vi "MAIN.vi"() -> ()   [LabVIEW 2015]
doc: "Use this template to create an application that executes repeatedly until you click the Stop button. This template polls the state of the Stop button and does not use events. Use the Top-Level Application template (not available in the Base package) to create a single-loop application with event handling."
uses:
  Control-CDC data.ctl
  Control-IMU data.ctl
  Control-Operation Test State FTS.ctl
  Lib_Bled112 toolkit/type_def/connection_status_bundle.ctl
  Lib_Bled112 toolkit/type_def/address_type.ctl
  Control-BLED Rx (EVENT-Attribute Client).ctl
  Lib_Bled112 toolkit/type_def/message_type.ctl
  Lib_Bled112 toolkit/type_def/message_class.ctl
  sub/Operation mode.ctl
  sub/Linerity State.ctl
  <vilib>/Utility/miscctls.llb/LVPointTypeDef.ctl
  SUB_Load and Save Controls.llb/RWC_Actions.ctl
  <vilib>/Utility/miscctls.llb/LVRowAndColumnTypeDef.ctl
  Type definition/write_mode.ctl
  Control-Operation State Mark10.ctl
  <vilib>/event_ctls.llb/eventvkey.ctl
  sub/File Control/File_Control_mode.ctl
  sub/Power supply/382280_mode.ctl
  <vilib>/Analysis/baseanly.llb/Mean (DBL).vi
  <vilib>/Utility/config.llb/Read Key (String).vi
  <vilib>/Utility/config.llb/Read Key (I32).vi
  Lib_Bled112 toolkit/ble_functions/ble_write_by_handle_uint8array.vi
  <vilib>/Utility/config.llb/Write Key (String).vi
  <vilib>/Utility/config.llb/Write Key (U32).vi
  <vilib>/Utility/config.llb/NI_LVConfig.lvlib
  <vilib>/Analysis/NI_AALBase.lvlib
  <vilib>/Utility/sysdir.llb/System Directory Type.ctl
  <vilib>/Utility/NIReport.llb/NI_report.lvclass
  <vilib>/addons/_office/NI_ReportGenerationToolkit.lvlib
  <vilib>/addons/_office/excel.llb/Excel Easy Table (str).vi
  <vilib>/Utility/NIReport.llb/Excel/NI_Excel.lvclass
  <vilib>/addons/_office/_exclsub.llb/font.ctl
panel:
  in  "PWR OFF":bool
  in  "File Path Done":bool
  in  "Linerity State":T1
  in  "Mode":bool=TRUE
  out "Bat(raw)":u16 format="%04x"
  out "Disconnection ocurrence":refnum<k4>
  out "Test Data table for Load Accuarcy Test":string[][](table)=[["-", "-", "-", "-", "-", "-", "-"], ["-", "-", "-", "-", "-", "-", "-"], ["-", "-", "-", "-", "-", "-", "-"], ["-", "-", "-", "-", "-", "-", "-"], ["-", "-", "-", "-", "-", "-", "-"], ["-", "-", "-", "-", "-", "-", "-"], ["-", "-", "-", "-", "-", "-", "-"], ["-", "-", "-", "-", "-", "-", "-"], ["-", "-", "-", "-", "-", "-", "-"]]
  out "Packet No.":u16
  out "Rx-debug":bool
  out "FTS table index":i32
  out "ms timer 5":u32=38996702
  out "ms timer 4":u32=27271323
  out "ms timer 3":u32=38996702
  in  "Update(ms)":u16=100
  out "ms timer 2":u32=38996702
  out "Rx-ROM":bool
  out "BLE Packet (mon)":u8[](array[numeric])=[119, 32, 48, 163, 32, 0, 45, 32, 53, 143, 30, 162, 83, 32, 86, 151, 32, 67, 185, 208, 89, 94, 66, 75, 91, 193, 107, 187, 98, 158, 102, 165, 208]
  out "Timer-ble log":u32=38996556
  in  "log data1":bool
  out "log ble buf":string
  out "Packet Detect":bool
  out "Disconnected":bool
  out "Rx buf 1":string
  out "Rx Cnt":i32
  out "Rx Packet Structure":T2={"Message Type (Response)"=128, "Payload length"=25, "Command Class (System)"=4, "Message ID"=5, "Connection handle"=0, "Attribute handle"=11, "Attribute type"=1, "Attribute value (data)"=[119, 32, 48, 110, 31, 255, 217, 32, 53, 83, 30, 161, 69, 32, 87, 130, 32, 68, 21, 209]} {"Attribute type" format="%02x" items=["read", "notify", "indicate", "read_by_type", "read_blob", "indicate_rsp_req"]; "Attribute value (data)" format="%02x"; "Attribute handle" format="%04x"; "Connection handle" format="%02x"; "Message ID" format="%02x"; "Message Type (Response)" format="%02x" items=["Command / Response"=0, "Event"=128]; "Command Class (System)" format="%02x" items=["System", "Persistent Store", "Attribute database", "Connection", "Attribute client", "Security Manager", "Generic Access Profile", "Hardware"]}
  out "Device Name":string="GEN4_PERSONA_3rd_jun"
  out "Connection Status":T5={"MAC Address"="F8:B8:54:EF:76:8D", "cnx handle"=0, "cnx flags"=5, "Address Type"=1, "Connection Interval (ms)"=8, "Timeout(ms)"=1000, "Latency"=0, "bonding handle"=255} {"Address Type" items=["Public", "Random"]}
  in  "Log no":string="1" caption="No."
  in  "FTS OP status":T7="Test_Start"
  out "Test profile":string[][](array[string])=[["Load(1)-0lb", "0", "1000", "0", "0"], ["Init(1)-70lb", "70", "1000", "0", "0"], ["Init(2)-140lb", "140", "1000", "0", "0"], ["Init(1)-70lb", "70", "1000", "0", "0"], ["Init(2)-140lb", "140", "1000", "0", "0"], ["Load(1)-0lb", "0", "10000", "1", "1"], ["Load(2)-10lb", "10", "3000", "0", "1"], ["Load(3)-20lb", "20", "3000", "0", "1"], ["Load(4)-40lb", "40", "3000", "0", "1"], ["Load(5)-60lb", "60", "3000", "0", "1"], ["Load(6)-80lb", "80", "3000", "0", "1"]]
  out "log refnum":refnum<file> caption="참조 번호 복제"
  out "ms timer":u32=38996556
  out "Logging No.":u32
  in  "Data Logging":bool caption="Data Logging (Desktop folder)"
  out "RxD":string
  out "Graph timer 2":u32=38996702
  out "Maximize window":bool
  out "Comm err cnt 1":i32
  out "Graph timer 1":u32=38996702
  in  "Setting load":bool=TRUE
  out "ACT-Comm":bool
  in  "Comm con 1":bool
  in  "Port close 1":bool
  in  "Port open 1":bool
  in  "탭-Top":T8(tab)
  in  "CDC Graph plot":bool
  in  "Offset Souce":enum32{"Normal", "Raw"}(radio)
  out "CDC Offet":T9 caption="CDC Offset data" {"Right Wing-C, C6/C0" format="%#.9f"; "Right Wing-B, C5/C0" format="%#.9f"; "Right Wing-A, C4/C0" format="%#.9f"; "Left Wing-C, C3/C0" format="%#.9f"; "Left Wing-B, C2/C0" format="%#.9f"; "Left Wing-A, C1/C0" format="%#.9f"}
  in  "Export graph 1":bool
  in  "Clear graph 1":bool
  out "CDC(PCAP02) Graph":waveform(dbl)[](graph)=[{"t0"=timestamp(3566271640.952271 s since 1904-01-01), "dt"=0.10400000000000001, "Y"=[22878.0]}, {"t0"=timestamp(3566271640.952271 s since 1904-01-01), "dt"=0.10400000000000001, "Y"=[16971.0]}, {"t0"=timestamp(3566271640.952271 s since 1904-01-01), "dt"=0.10400000000000001, "Y"=[23489.0]}, {"t0"=timestamp(3566271640.952271 s since 1904-01-01), "dt"=0.10400000000000001, "Y"=[27579.0]}, {"t0"=timestamp(3566271640.952271 s since 1904-01-01), "dt"=0.10400000000000001, "Y"=[25246.0]}, {"t0"=timestamp(3566271640.952271 s since 1904-01-01), "dt"=0.10400000000000001, "Y"=[26279.0]}, {"t0"=timestamp(3566271640.952271 s since 1904-01-01), "dt"=0.10400000000000001, "Y"=[1.0058650970458984]}, {"t0"=timestamp(3566271640.952271 s since 1904-01-01), "dt"=0.10400000000000001, "Y"=[0.9999599456787109]}, {"t0"=timestamp(3566271640.952271 s since 1904-01-01), "dt"=0.10400000000000001, "Y"=[1.0064787864685059]}, {"t0"=timestamp(3566271640.952271 s since 1904-01-01), "dt"=0.10400000000000001, "Y"=[0.9571785926818848]}, {"t0"=timestamp(3566271640.952271 s since 1904-01-01), "dt"=0.10400000000000001, "Y"=[1.0106620788574219]}, {"t0"=timestamp(3566271640.952271 s since 1904-01-01), "dt"=0.10400000000000001, "Y"=[1.0083107948303223]}]
  out "CDC data":T9 caption="CDC Monitoring data" {"Right Wing-C, C6/C0" format="%#.9f"; "Right Wing-B, C5/C0" format="%#.9f"; "Right Wing-A, C4/C0" format="%#.9f"; "Left Wing-C, C3/C0" format="%#.9f"; "Left Wing-B, C2/C0" format="%#.9f"; "Left Wing-A, C1/C0" format="%#.9f"}
  in  "Offset 1":bool
  out "IMU Offet":T10 caption="IMU Offset data" {"Accelerometer Z" format="%#.9f"; "Accelerometer Y" format="%#.9f"; "Accelerometer X" format="%#.9f"; "Gyroscope Z" format="%#.9f"; "Gyroscope Y" format="%#.9f"; "Gyroscope X" format="%#.9f"}
  out "IMU Graph":waveform(dbl)[](graph)=[{"t0"=timestamp(3566271136.852438 s since 1904-01-01), "dt"=0.108, "Y"=[-1.063125]}, {"t0"=timestamp(3566271136.852438 s since 1904-01-01), "dt"=0.108, "Y"=[0.118125]}, {"t0"=timestamp(3566271136.852438 s since 1904-01-01), "dt"=0.108, "Y"=[0.20125]}, {"t0"=timestamp(3566271136.852438 s since 1904-01-01), "dt"=0.108, "Y"=[-0.014029999999999999]}, {"t0"=timestamp(3566271136.852438 s since 1904-01-01), "dt"=0.108, "Y"=[-0.00366]}, {"t0"=timestamp(3566271136.852438 s since 1904-01-01), "dt"=0.108, "Y"=[1.0149789999999999]}]
  in  "Clear graph 2":bool
  in  "Export graph2":bool
  out "IMU data":T10 caption="IMU Monitoring data" {"Accelerometer Z" format="%#.9f"; "Accelerometer Y" format="%#.9f"; "Accelerometer X" format="%#.9f"; "Gyroscope Z" format="%#.9f"; "Gyroscope Y" format="%#.9f"; "Gyroscope X" format="%#.9f"}
  in  "Offset 2":bool
  out "Full ROM data":bool
  in  "Flash Map":enum32{"Data Map", "Raw Data"}(tab)
  out "ROM Table":string[][](table)=[["Device ID", "-", "-"], ["YEAR", "-", "-"], ["Month", "-", "-"], ["Day", "-", "-"], ["Device Type", "-", "-"], ["Manufacturer ID", "-", "-"], ["Cal_Scale A", "-", "-"], ["Cal_Scale B", "-", "-"], ["Cal_Acc. X", "-", "-"], ["Cal_Acc. Y", "-", "-"], ["Cal_Acc. Z", "-", "-"], ["Cal_Gy. X", "-", "-"], ["Cal_Gy. Y", "-", "-"], ["Cal_Gy. Z", "-", "-"], ["Cal_Vol H", "-", "-"], ["Cal_Vol L", "-", "-"], ["Cal_CDC Off 1", "-", "-"], ["Cal_CDC Off 2", "-", "-"], ["Cal_CDC Off 3", "-", "-"], ["Cal_CDC Off 4", "-", "-"], ["Cal_CDC Off 5", "-", "-"], ["Cal_CDC Off 6", "-", "-"], ["Cal_CDC Off 7", "-", "-"], ["Cal_CDC Off 8", "-", "-"]]
  out "Rx ROM-log":string
  out "ROM Data":T11(array[cluster]) {"Index" format="%02x"; "ROM Data" format="%02x"}
  in  "Operation Mode":T12
  in  "Mode Selection":bool
  in  "Data Log":string
  out "Data_mon(h)":string
  in  "Data(h)":string="\u0001"
  in  "Send":bool
  in  "Handle":u8=16 format="%02x"
  in  "Mode Protocol":enum32{"Normal", "Debugging 1", "Debugging 2"}(tab)
  in  "File path":path
  in  "All Graph data save":bool
  in  "Set Inverval Time":bool
  in  "Grahp Clear":bool
  out "BLE RSSI buf":i16(graph)=-63
  out "BLE RSSI Graph":dbl(graph)=-65.56666666666666
  out "BLE RSSI (dBm)":dbl format="%.1f"
  out "BLE AVG-Interval Graph":dbl(graph)=11.355
  out "BLE Interval Time(ms)":dbl format="%.1f"
  out "BLE Interval buf":u32(graph)=11
  in  "Interval Time":enum16{"10ms", "33ms", "50ms"}(ring)
  out "Port Error":bool
  in  "ADC Linearity Stop":bool
  in  "Power Supply Port":refnum<visa-resource-name>
  out "Linearity monitoring graph":cluster{dbl[], dbl[]}(graph)
  in  "ADC Linearity Start":bool
  in  "Cal/Test select":bool=TRUE
  in  "Head Up":bool
  in  "Load(lb)":dbl=10.0 min=0.0 max=150.0 step=0.1
  in  "Test name":string="Noname"
  out "Load Graph":cluster{dbl[], dbl[]}(graph)
  out "Mark10 Gauge (lb)":dbl format="%.2f"
  out "Test Status":string
  out "Test Data table":string[][](table)=[["-", "-", "-", "-", "-", "-", "-"], ["-", "-", "-", "-", "-", "-", "-"], ["-", "-", "-", "-", "-", "-", "-"], ["-", "-", "-", "-", "-", "-", "-"], ["-", "-", "-", "-", "-", "-", "-"], ["-", "-", "-", "-", "-", "-", "-"], ["-", "-", "-", "-", "-", "-", "-"], ["-", "-", "-", "-", "-", "-", "-"], ["-", "-", "-", "-", "-", "-", "-"]]
  in  "Test Start":bool
  in  "Port-FTS":refnum<visa-resource-name>="COM6" caption="FTS \nCOM port"
  in  "FTS Testing":bool
  out "FTS comm.":bool
  in  "Force Set":bool
  in  "Save":bool
  in  "ROM Table 2":string[][](table)=[["Device ID", "-", "-"], ["YEAR", "-", "-"], ["Month", "-", "-"], ["Day", "-", "-"], ["Device Type", "-", "-"], ["Manufacturer ID", "-", "-"], ["Cal_Scale A", "-", "-"], ["Cal_Scale B", "-", "-"], ["Check sum", "-", "-"], ["Cal_Acc. X", "-", "-"], ["Cal_Acc. Y", "-", "-"], ["Cal_Acc. Z", "-", "-"], ["Cal_Gy. X", "-", "-"], ["Cal_Gy. Y", "-", "-"], ["Cal_Gy. Z", "-", "-"], ["Cal_Vol H", "-", "-"], ["Cal_Vol L", "-", "-"], ["Cal_CDC Off 1", "-", "-"], ["Cal_CDC Off 2", "-", "-"], ["Cal_CDC Off 3", "-", "-"], ["Cal_CDC Off 4", "-", "-"], ["Cal_CDC Off 5", "-", "-"], ["Cal_CDC Off 6", "-", "-"]] caption="ROM Table"
  out "Rx-mon":bool
  out "Comm con status 1":bool caption="Status"
  out "*Board ID1":string="None...." caption="S/N"
  in  "Port-set 1":refnum<visa-resource-name>="COM8" caption="COM port"
  out "Port-act 1":refnum<visa-resource-name>="COM8"
  in  "stop":bool=TRUE
  out "Data trx(led)":bool
  in  "Setting load(led)":bool
  out "status string":string="Ready (available after the communication connection)"
  # "GEN4 PP4 - GUI Program"
  # "Ver. 170428D"
  # "Comm. Connection"
  # "(Connection)"
  # "Serial port"
  # "Reserved"
  # "Gyroscope X"
  # "Gyroscope Y"
  # "Gyro. (dps)"
  # "Gyroscope Z"
  # "Accelerometer X"
  # "Accelerometer Y"
  # "Acc. (g)"
  # "Accelerometer Z"
  # "Unless otherwise specified, Maximum value is 65535(FFFFh)."
  # "* Normal Operation Mode\nHandler : 0x000B\nWrite : 0x69 0x6D 0x74"
  # "* Debugging Mode 1\nHandler : 0x000B\nWrite : 0x4A 0x73 0x50"
  # "* Debugging Mode 2\nHandler : 0x000B\nWrite : 0x4E 0x46 0x54"
  # "Linearity Inspection"
  # "ESM301: 115200bps\nMARK10: 9600bps"
  # "Unless otherwise specified, Maximum value is 65535 (FFFFh)."
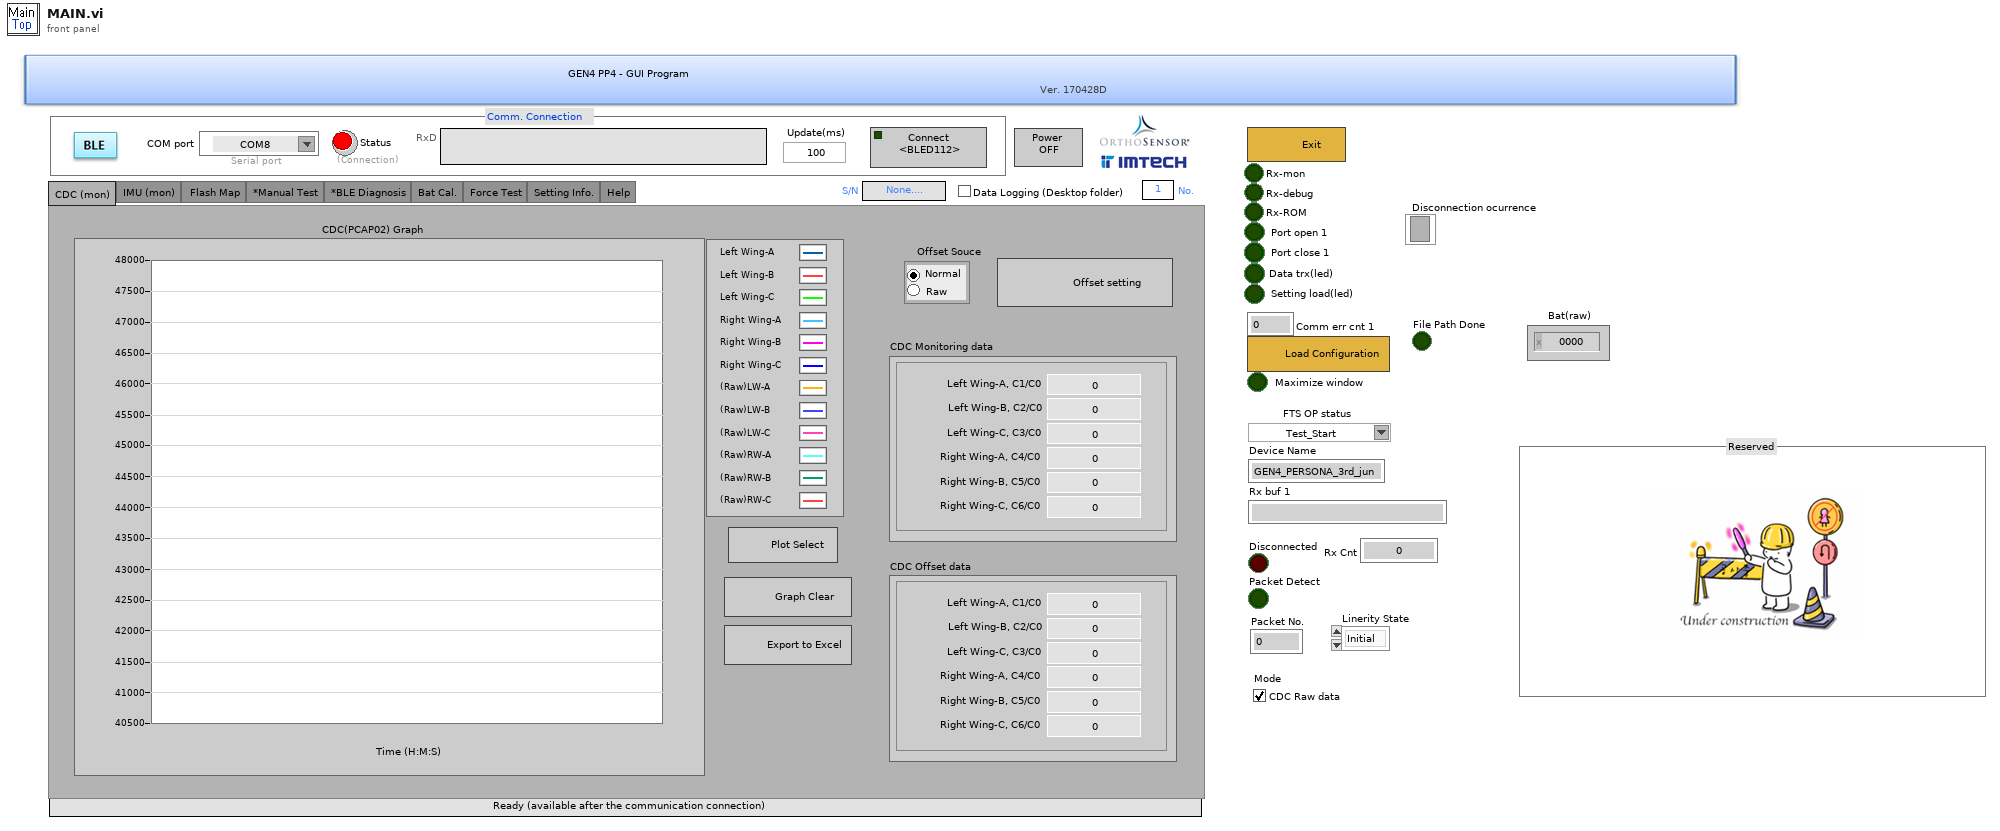
[diagram p1: front panel]
types:
  T1 = typedef "Linerity State.ctl" = enum16{"Initial", "Measurement", "End"}
  T2 = typedef "Control-BLED Rx (EVENT-Attribute Client).ctl" = cluster{"Message Type (Response)":T3, "Payload length":u8, "Command Class (System)":T4, "Message ID":u8, "Connection handle":u8, "Attribute handle":u16, "Attribute type":T4, "Attribute value (data)":u8[]}
  T3 = typedef "message_type.ctl" = u8
  T4 = typedef "message_class.ctl" = u8
  T5 = typedef "connection_status_bundle.ctl" = cluster{"MAC Address":string, "cnx handle":u8, "cnx flags":u8, "Address Type":T6, "Connection Interval (ms)":u16, "Timeout(ms)":u16, "Latency":u16, "bonding handle":u8}
  T6 = typedef "address_type.ctl" = u8
  T7 = typedef "Control-Operation Test State FTS.ctl" = string
  T8 = enum32{"CDC (mon)", "IMU (mon)", "Flash Map ", "*Manual Test", "*BLE Diagnosis", "Bat Cal.", "Force Test", "Setting Info.", "Help"}
  T9 = typedef "Control-CDC data.ctl" = cluster{"Left Wing-A, C1/C0":dbl, "Left Wing-B, C2/C0":dbl, "Left Wing-C, C3/C0":dbl, "Right Wing-A, C4/C0":dbl, "Right Wing-B, C5/C0":dbl, "Right Wing-C, C6/C0":dbl}
  T10 = typedef "Control-IMU data.ctl" = cluster{"Gyroscope X":dbl, "Gyroscope Y":dbl, "Gyroscope Z":dbl, "Accelerometer X":dbl, "Accelerometer Y":dbl, "Accelerometer Z":dbl}
  T11 = cluster{"RxOK":bool, "ROM Data":u8[], "Index":u8}[]
  T12 = typedef "Operation mode.ctl" = enum16{"Normal Operation", "Debugging 1", "Debugging 2"}
  T13 = enum8{"Enabled", "Disabled", "Disabled and Grayed Out"}
  T14 = typedef "RWC_Actions.ctl" = enum16{"Read", "Write", "Read and Create"}
  T15 = enum16{"Always On", "Always Off", "Off While Running"}
  T16 = typedef "LVPointTypeDef.ctl" = cluster{"Horizontal":i16, "Vertical":i16}
  T17 = cluster{"RxOK":bool, "ROM Data":u8[], "Index":u8}
  T18 = typedef "LVRowAndColumnTypeDef.ctl" = cluster{"Row":i32, "Column":i32}
  T19 = enum16{"Standard Report", "HTML", "Word", "Excel"}
  T20 = enum16{"maximized", "minimized", "normal", "no change"}
  T21 = typedef "NI_ReportGenerationToolkit.lvlib/font.ctl" = cluster{"font name":string, "font size":dbl, "bold":u16, "italic":u16, "underline":u16, "strike through":u16, "font color":u32}
  T22 = cluster{"on/off":bool, "weight":i32, "color":u32}
  T23 = typedef "write_mode.ctl" = enum16{"Save Flash", "Visa save", "Interval Change"}
  T24 = typedef "Control-Operation State Mark10.ctl" = string
  T25 = typedef "eventvkey.ctl" = enum16{"ASCII", "Enter", "Return", "Shift", "Ctrl", "Alt", "Cmd", "Opt", "Caps", "NumLock", "Clear", "Break", "Up", "Down", "Left", "Right", "Insert", "Delete", "Home", "End", "PageUp", "PageDown", "Escape", "Help", "Pause", "ScrollLock", "F1", "F2", "F3", "F4", "F5", "F6", "F7", "F8", "F9", "F10", "F11", "F12", "F13", "F14", "F15", "F16", "F17", "F18", "F19", "F20", "F21", "F22", "F23", "F24", "Play", "VolumeUp", "VolumeDown", "Mute", "Two Byte Char"}
  T26 = typedef "File_Control_mode.ctl" = enum16{"Open", "Write", "Close"}
  T27 = cluster{"LWA":dbl[], "LWB":dbl[], "LWC":dbl[], "RWA":dbl[], "RWB":dbl[], "RWC":dbl[], "Bat":u16[]}
  T28 = typedef "382280_mode.ctl" = enum16{"Open", "Close", "STBY", "OPER", "V SET", "A SET", "STATUS", "V Read", "A Read"}
  T29 = enum16{"open", "replace", "create", "open or create", "replace or create", "replace or create with confirmation"}
  T30 = typedef "NI_LVConfig.lvlib/Config Data RefNum.ctl" = refnum<k1>
  T31 = typedef "System Directory Type.ctl" = i32
  T32 = typedef "LVRectTypeDef.ctl" = cluster{"Left":i16, "Top":i16, "Right":i16, "Bottom":i16}
  T33 = typedef "PCAP zero information.ctl" = cluster{"Packet ID":u8, "Sensor 1":u16, "Sensor 2":u16, "Sensor 3":u16, "Sensor 4":u16, "Sensor 5":u16, "Sensor 6":u16, "Sensor 7":u16, "Sensor 8":u16}
  T34 = typedef "Cal information.ctl" = cluster{"Packet ID":u8, "Acc X_H_Cal":u8, "Acc X_L_Cal":u8, "Acc Y_H_Cal":u8, "Acc Y_L_Cal":u8, "Acc Z_H_Cal":u8, "Acc Z_L_Cal":u8, "Gyro X_H_Cal":u8, "Gyro X_L_Cal":u8, "Gyro Y_H_Cal":u8, "Gyro Y_L_Cal":u8, "Gyro Z_H_Cal":u8, "Gyro Z_L_Cal":u8, "Voltage H 3.1V":u8, "Voltage L 3.1V":u8, "Voltage H 2.8V":u8, "Voltage L 2.8V":u8}
  T35 = typedef "Device information.ctl" = cluster{"Packet ID":u8, "Device ID 1":u8, "Device ID 2":u8, "Device ID 3":u8, "Device ID 4":u8, "Year":u8, "Month":u8, "Day":u8, "Device Type H":u8, "Device Type L":u8, "Manufacturer Lot ID 1":u8, "Manufacturer Lot ID 2":u8, "Manufacturer Lot ID 3":u8, "Manufacturer Lot ID 4":u8, "Scale A":u8, "Scale B":u8, "Check sum":u8}
  T36 = typedef "Control-BLED Rx (EVENT-Connection status).ctl" = cluster{"Message Type (Response)":T3, "Payload length":u8, "Command Class (System)":T4, "Message ID":u8, "Connection handle":u8, "flags":u8, "Bluetooth address":u8[], "address type":T4, "conn_interval(ms)":dbl, "timeout(ms)":dbl, "latency":u16, "bonding(0xFF)":u8}
  T37 = typedef "Control-BLED Rx (Get RSSI).ctl" = cluster{"Message Type (Response)":T3, "Payload length":u8, "Message class":u8, "Message ID":u8, "connection":u8, "rssi":i16}
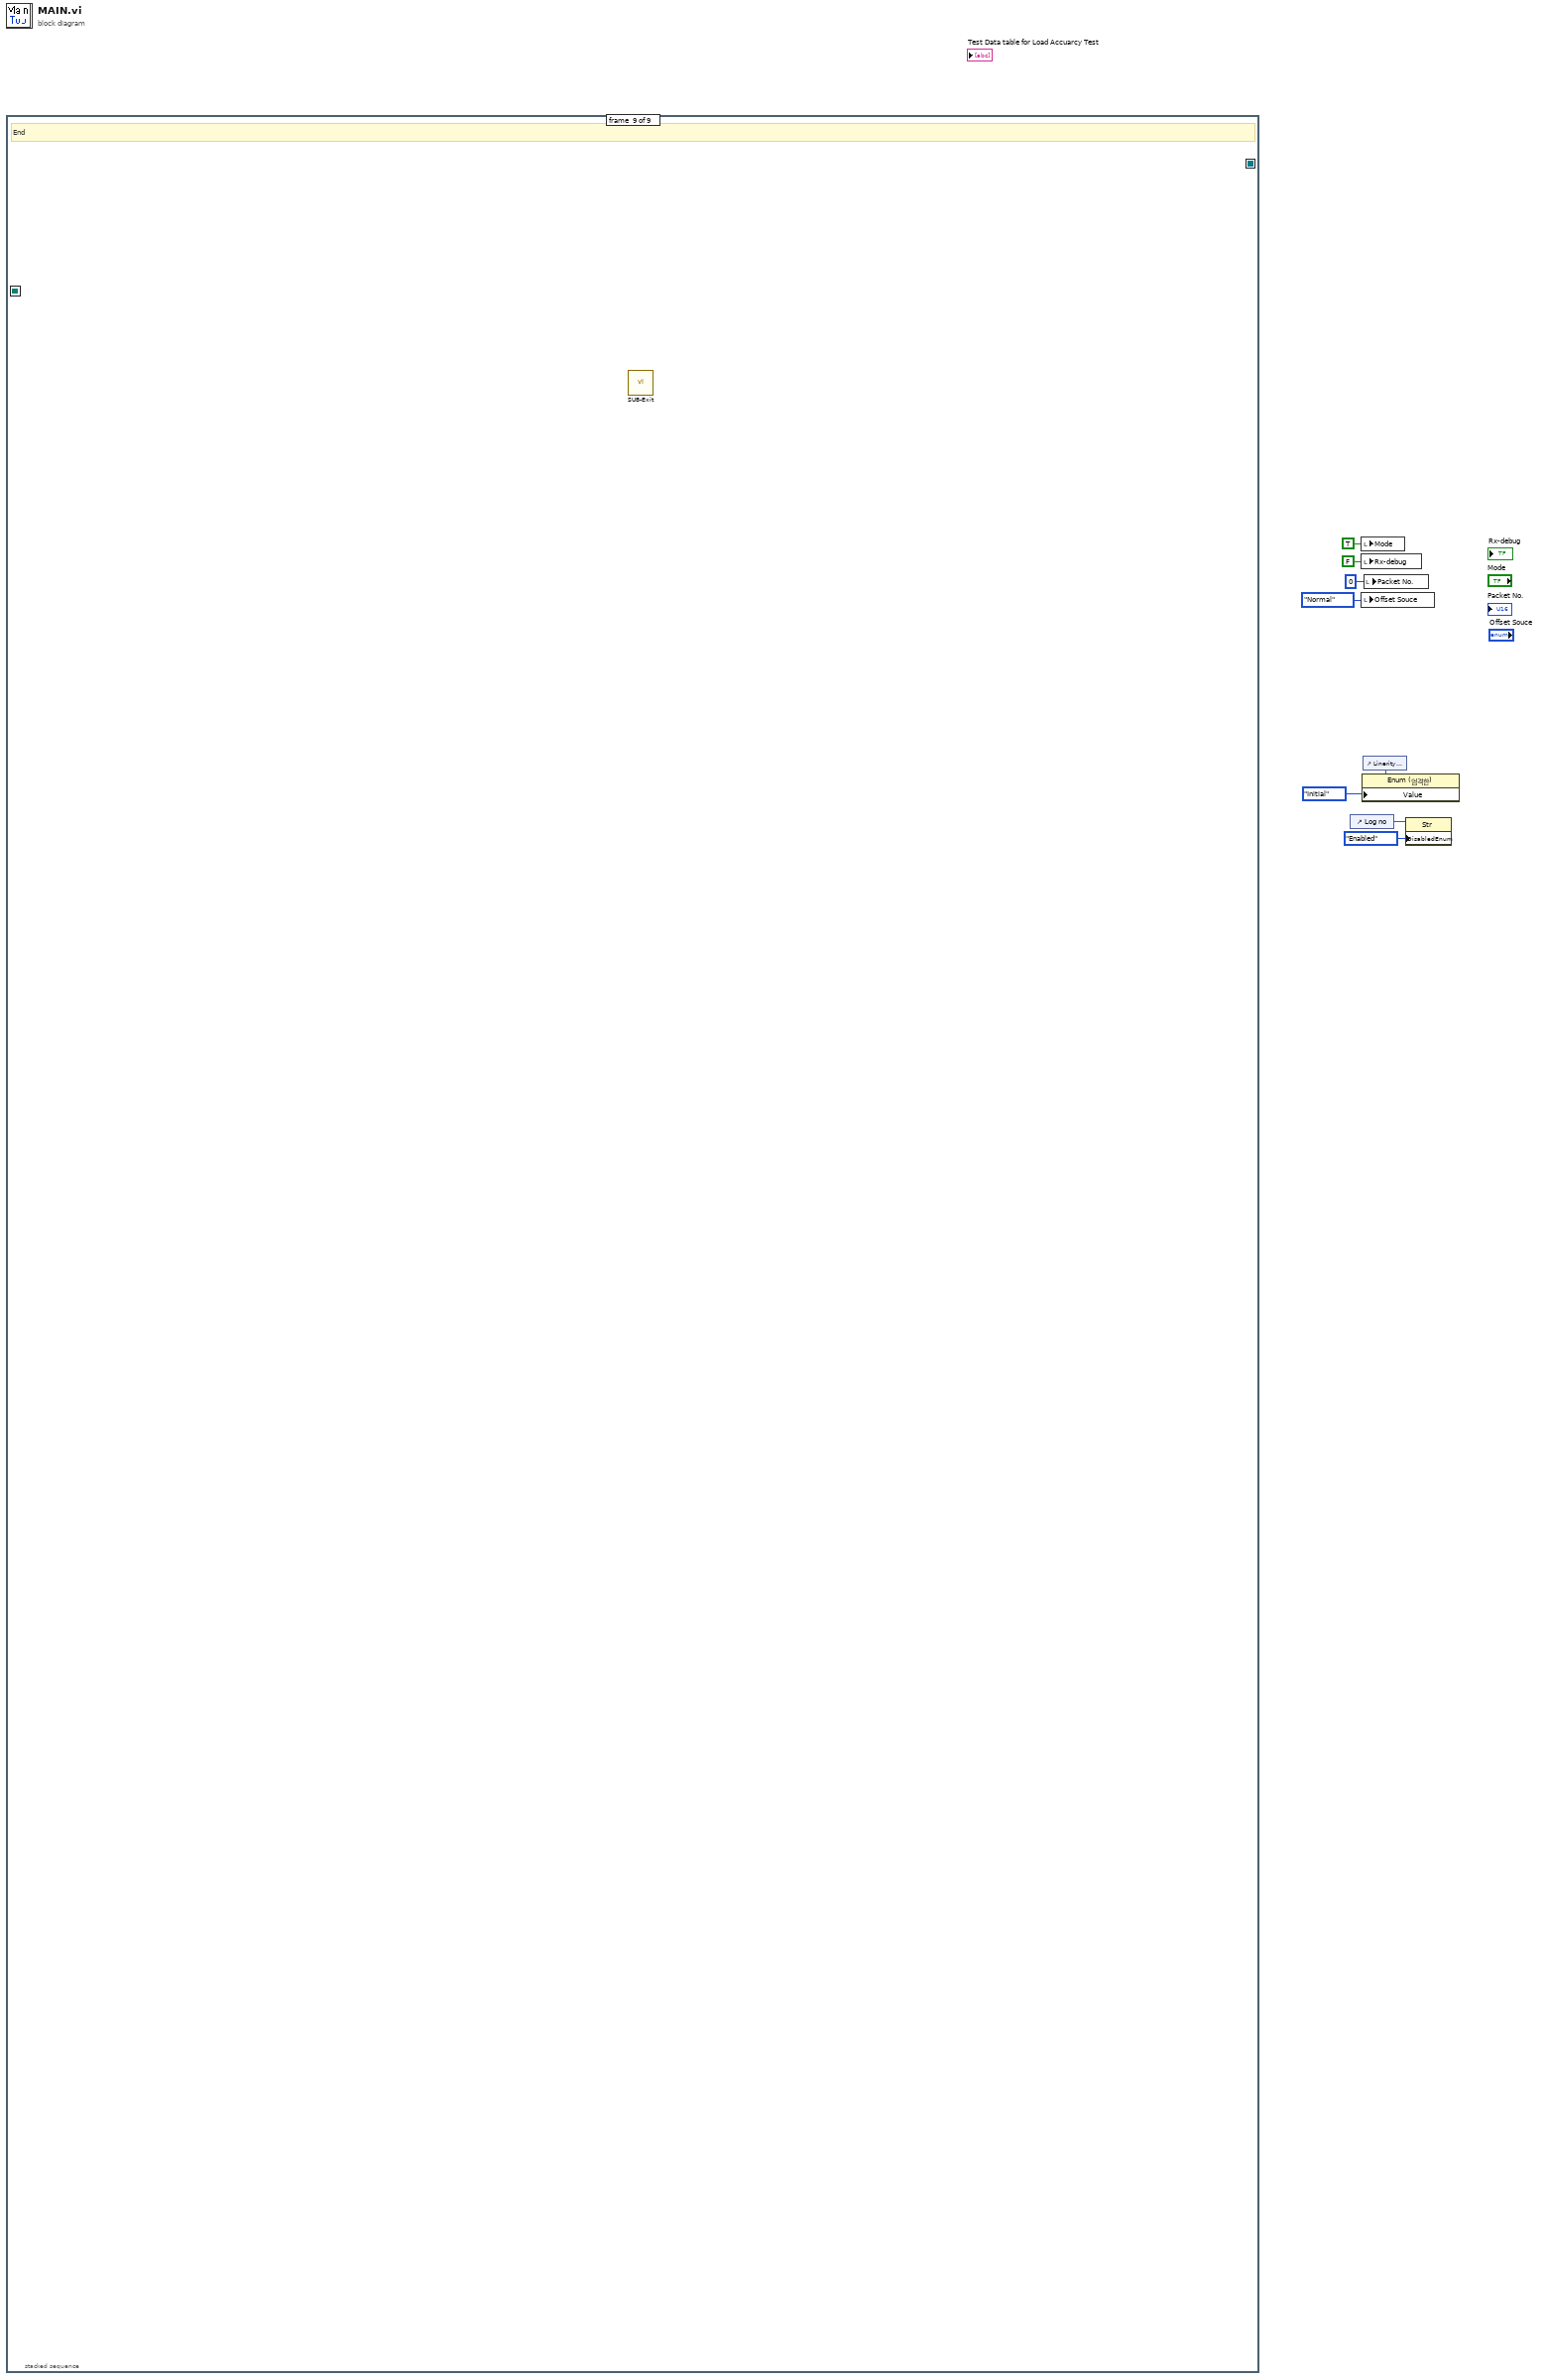
[diagram p0: block diagram]
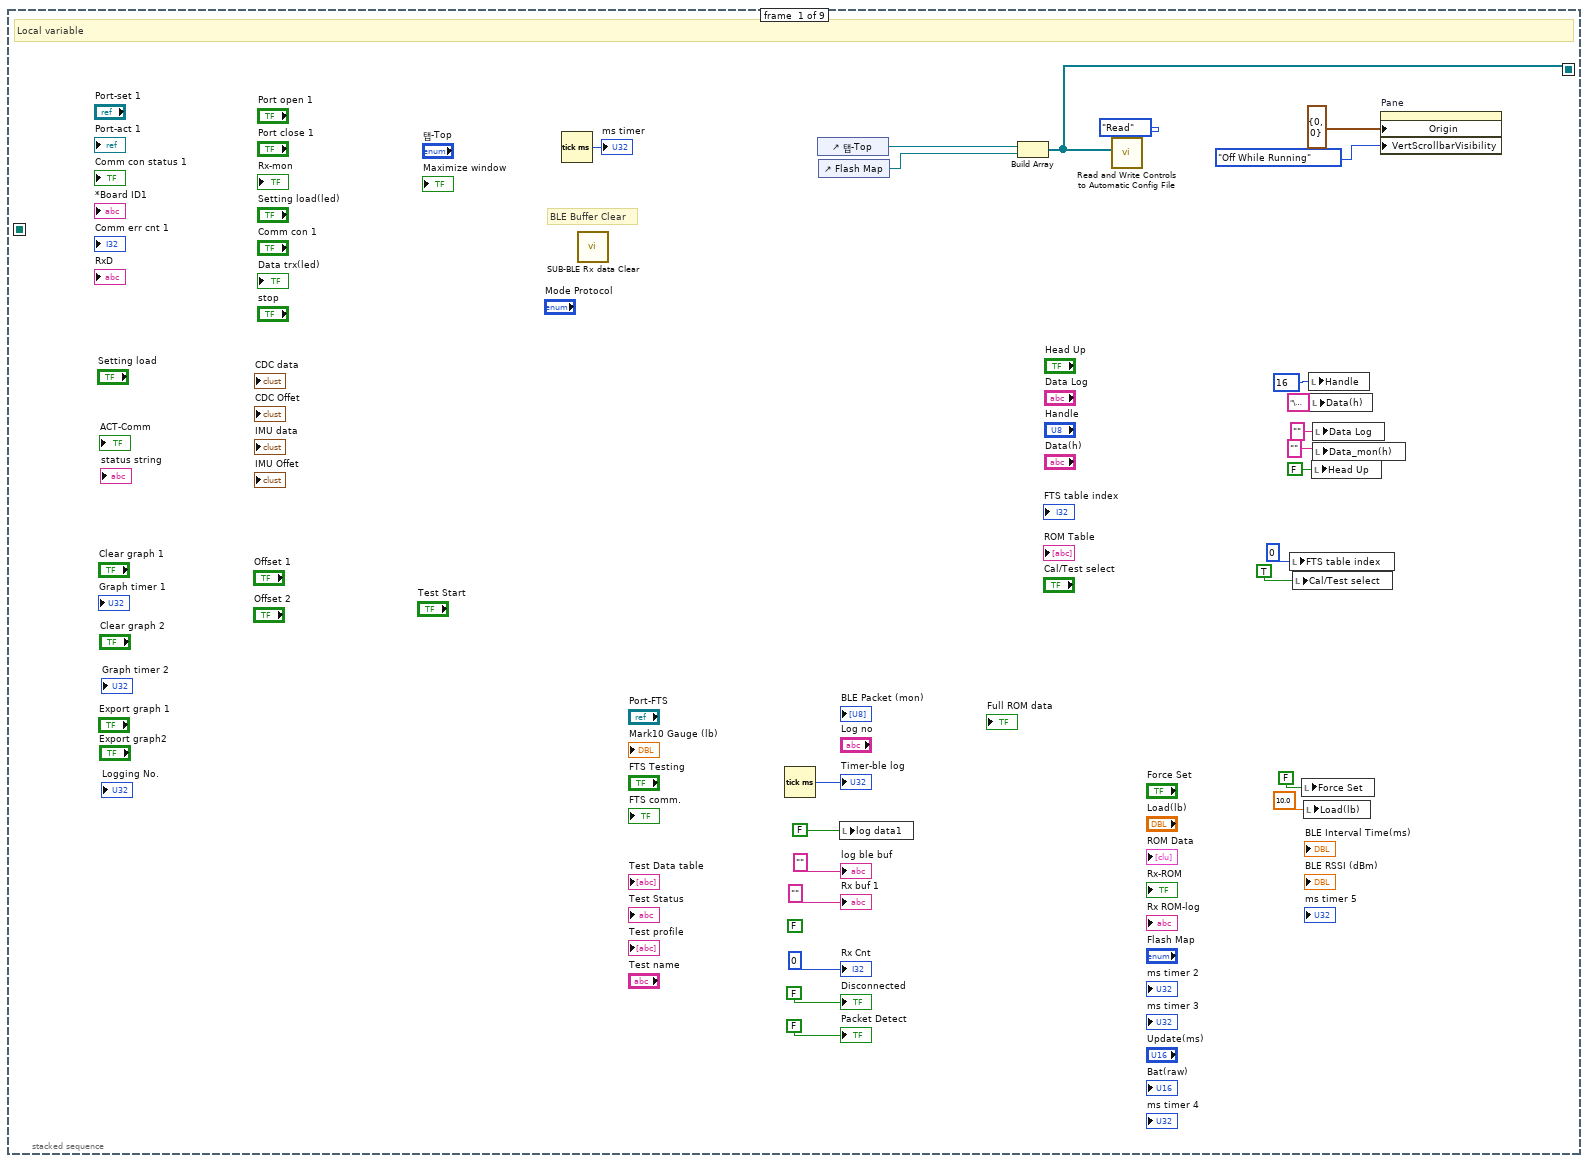
[diagram p2: hidden frame]
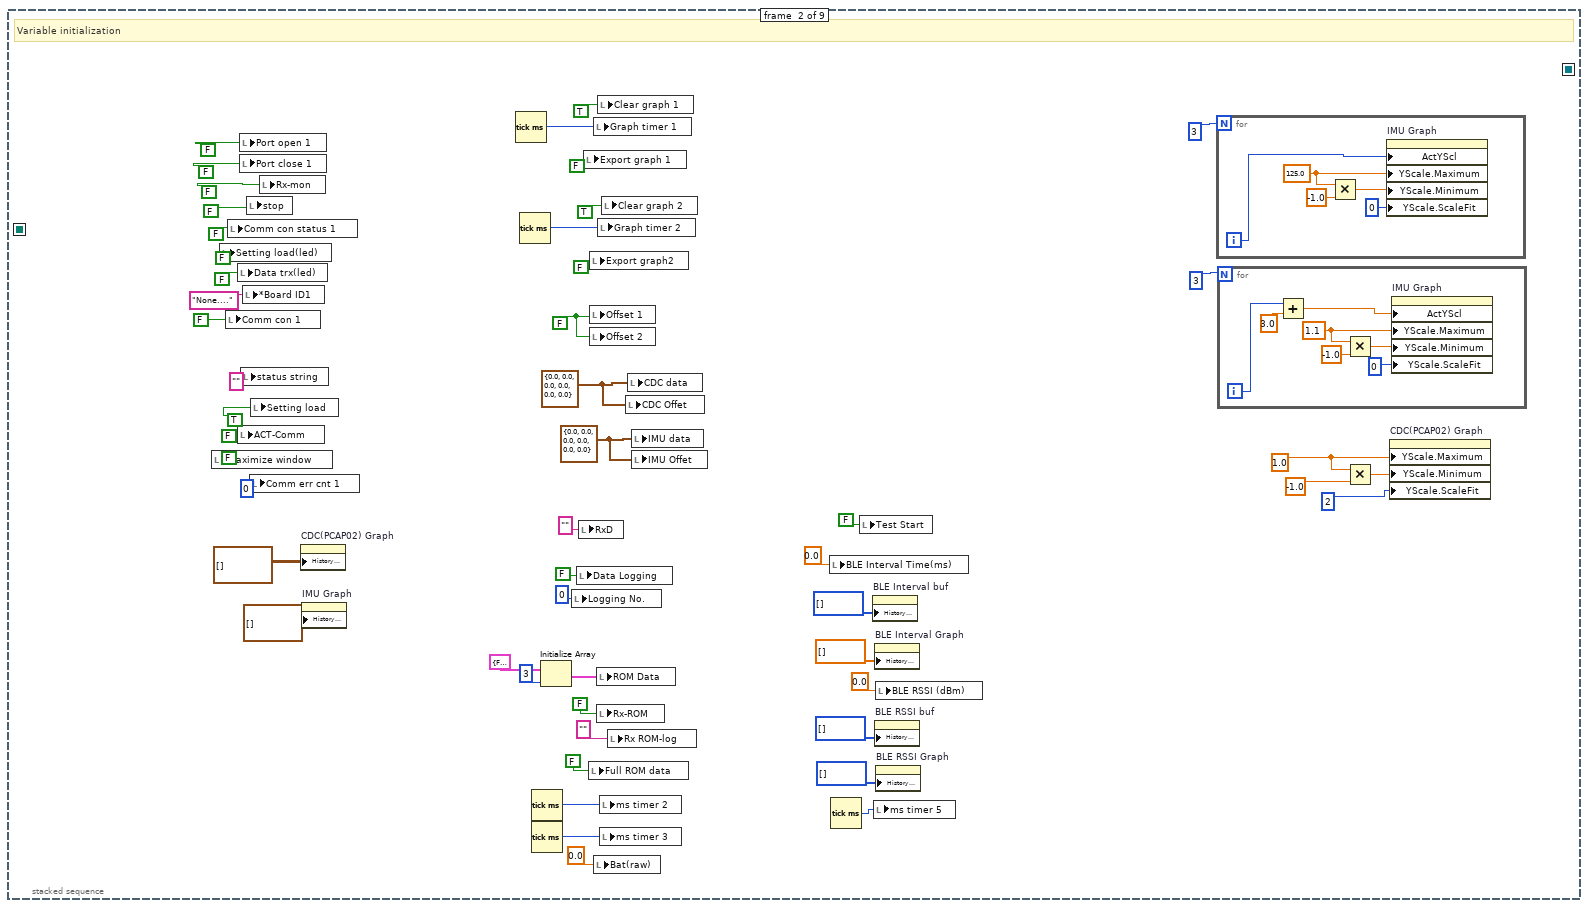
[diagram p3: hidden frame]
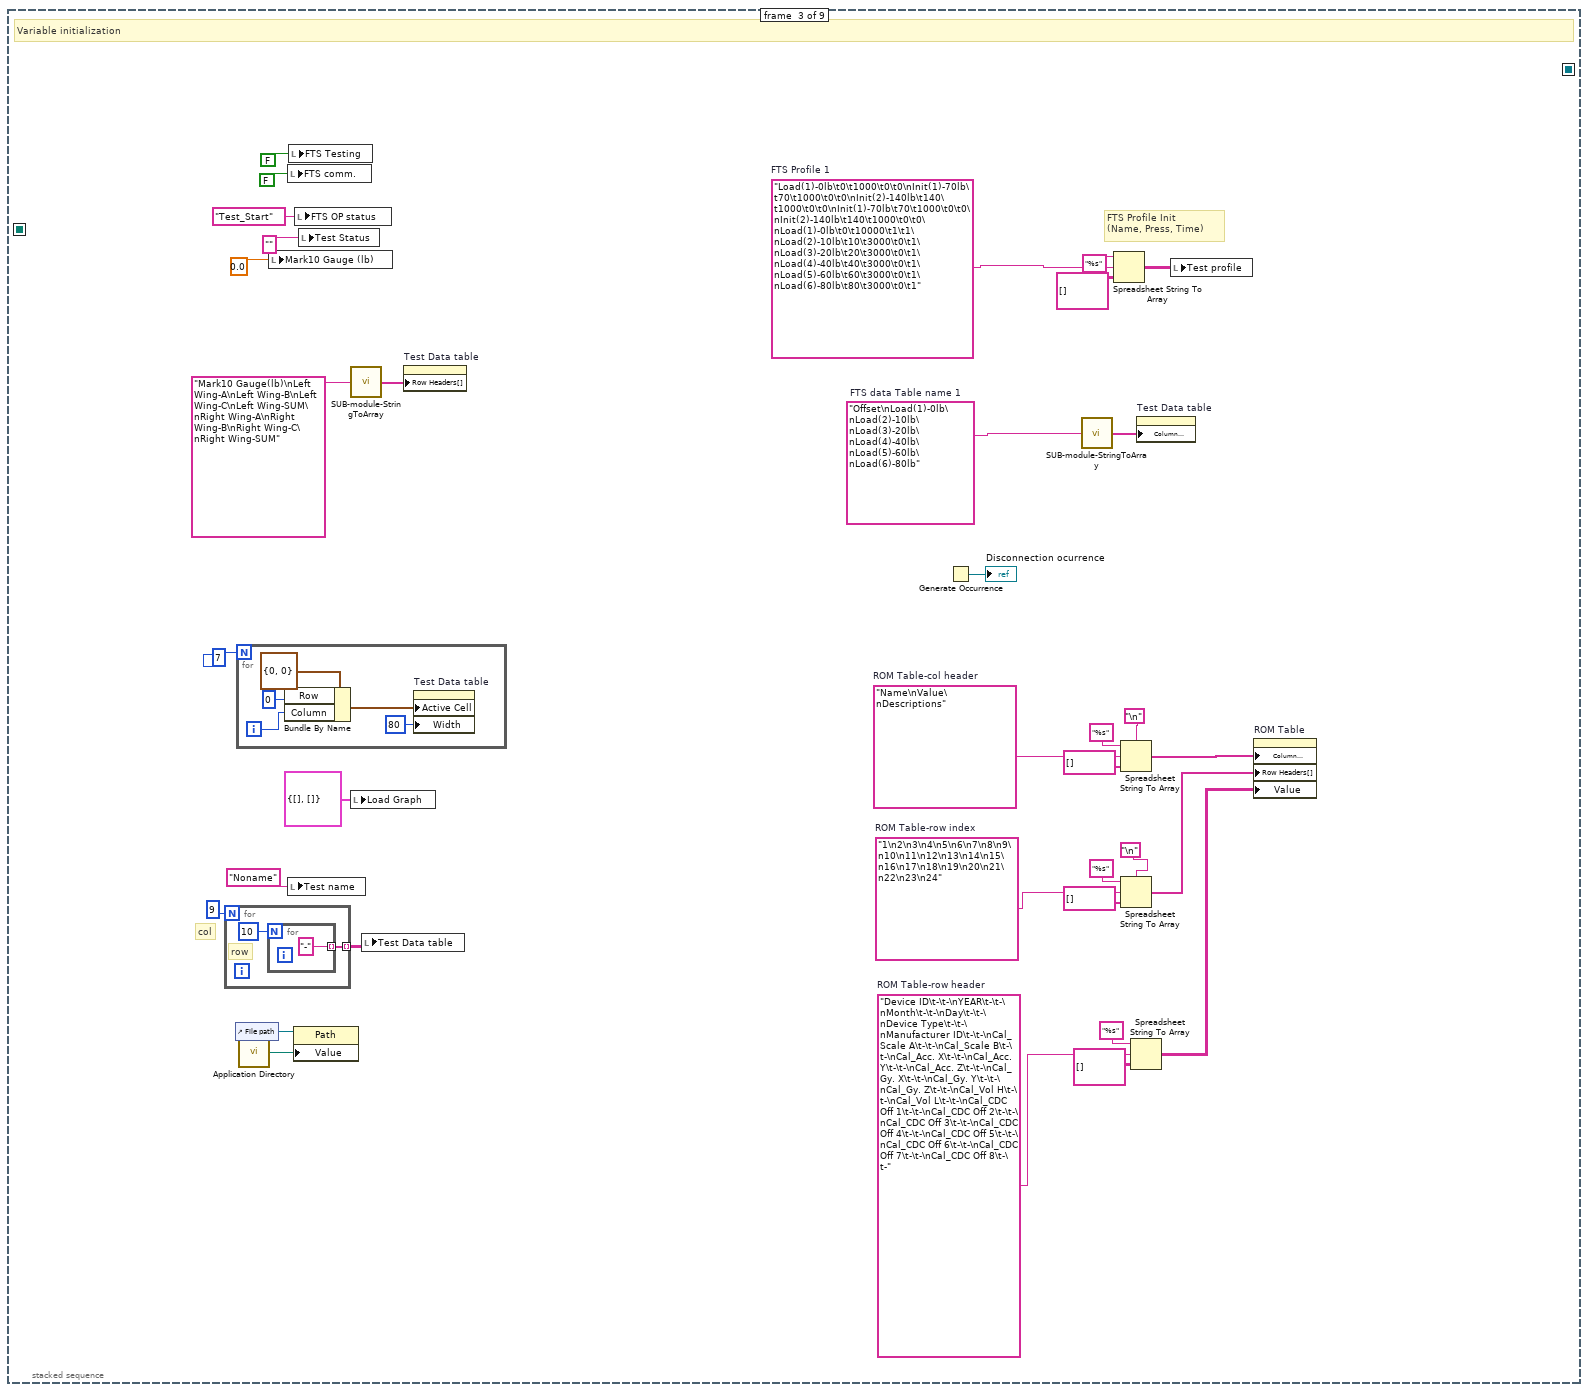
[diagram p4: hidden frame]
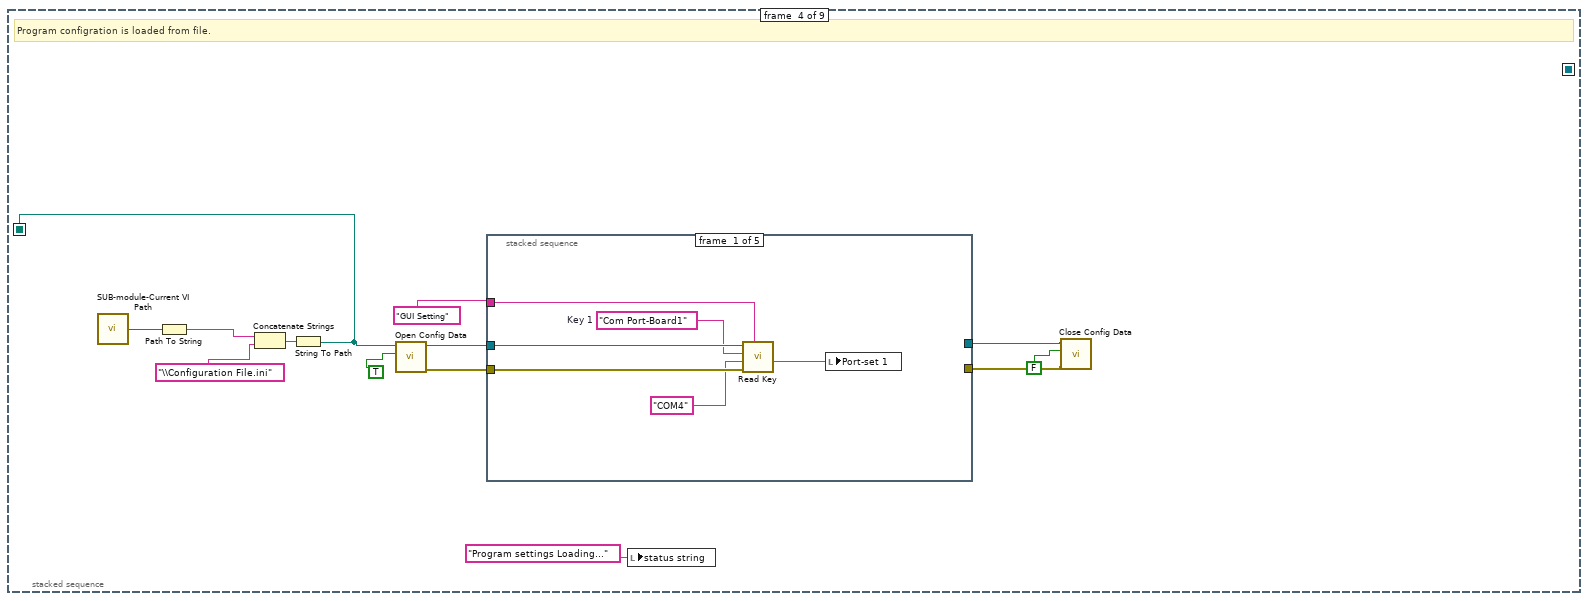
[diagram p5: hidden frame]
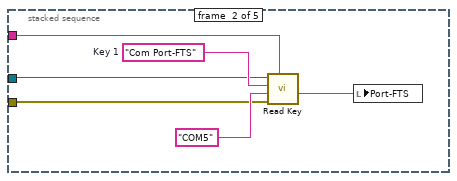
[diagram p6: hidden frame]
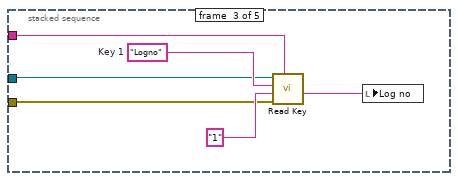
[diagram p7: hidden frame]
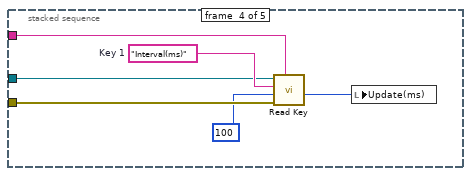
[diagram p8: hidden frame]
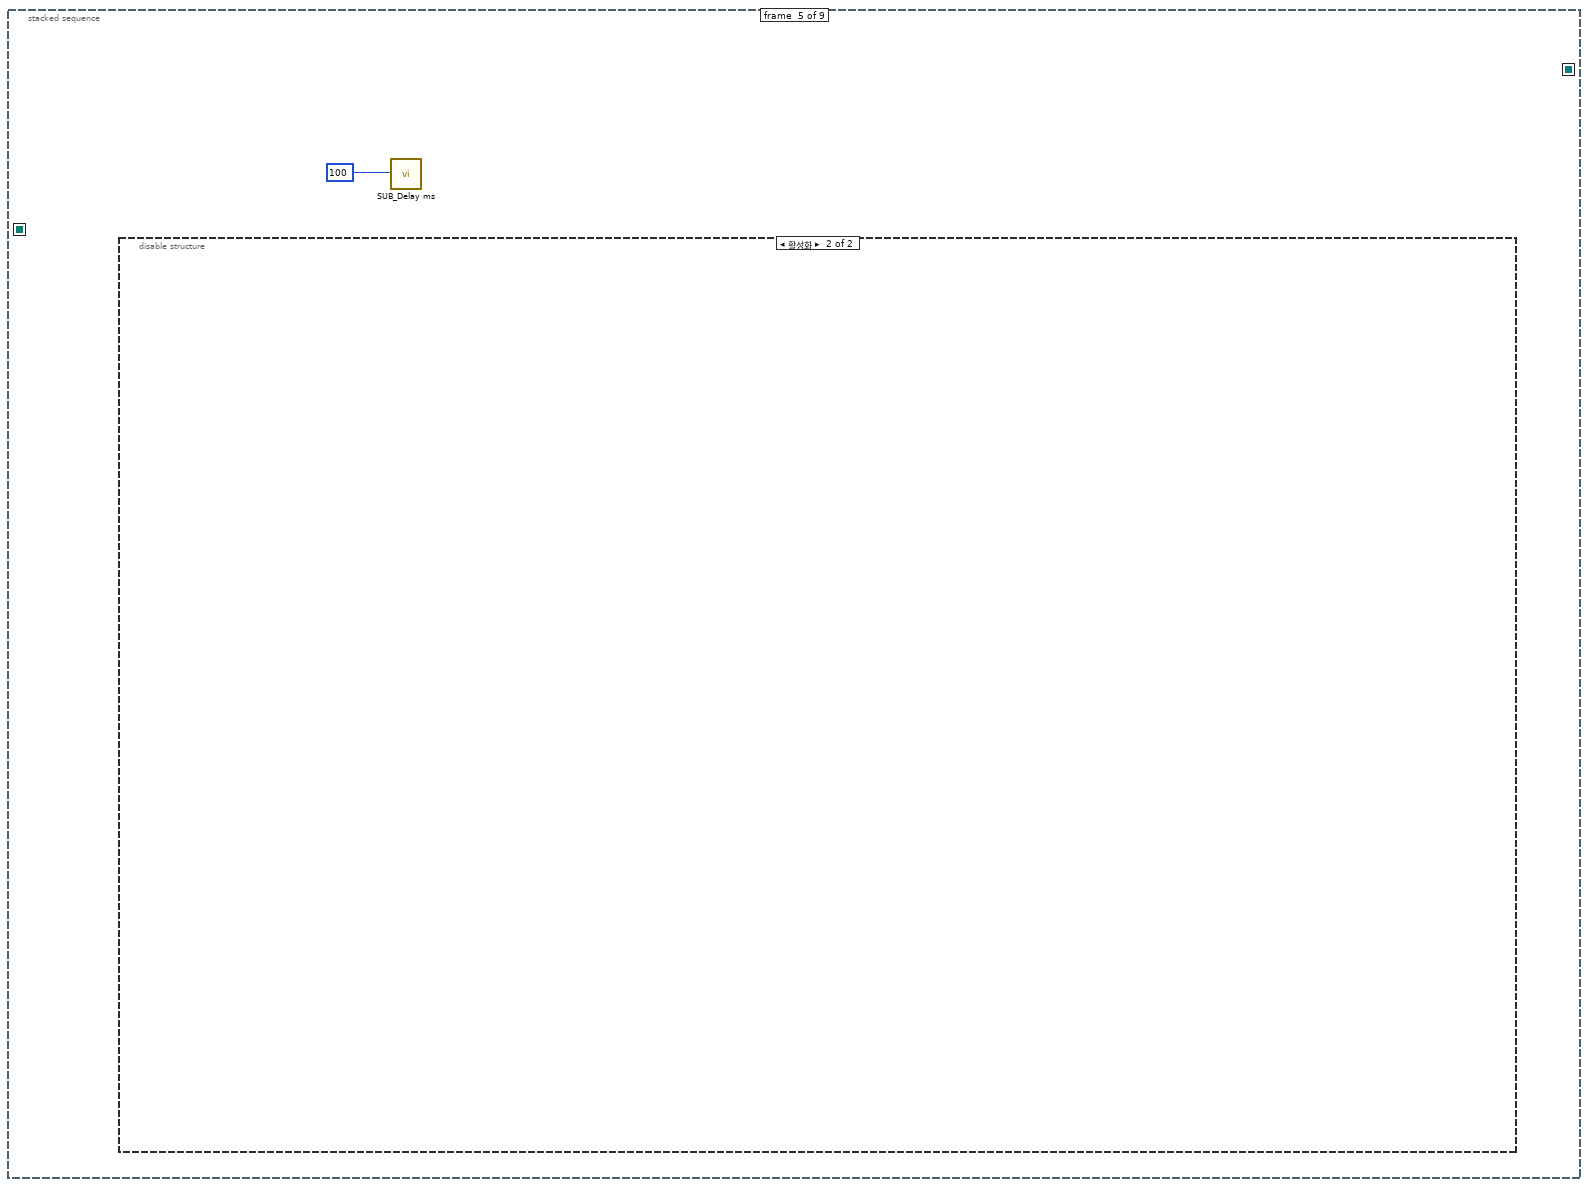
[diagram p10: hidden frame]
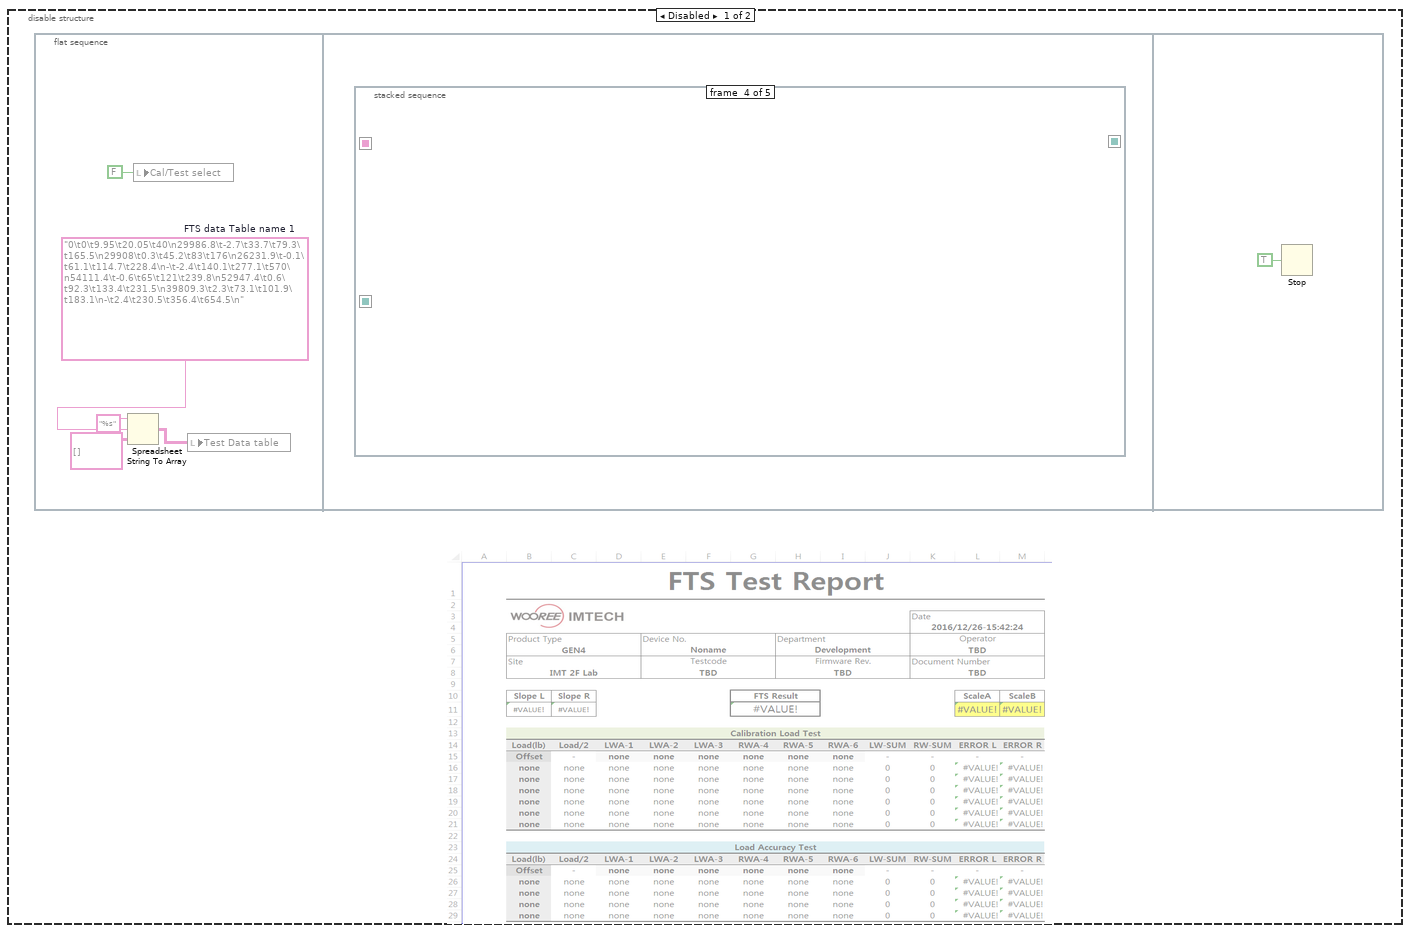
[diagram p11: hidden frame]
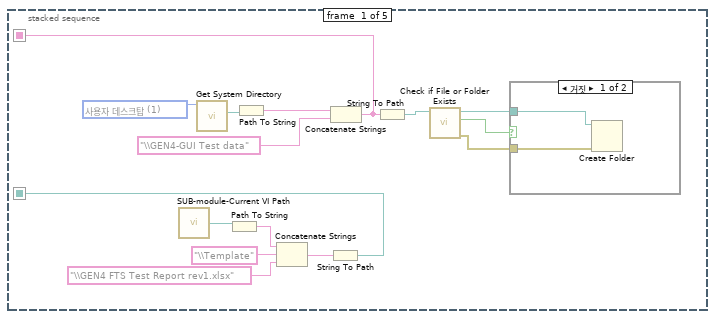
[diagram p12: hidden frame]
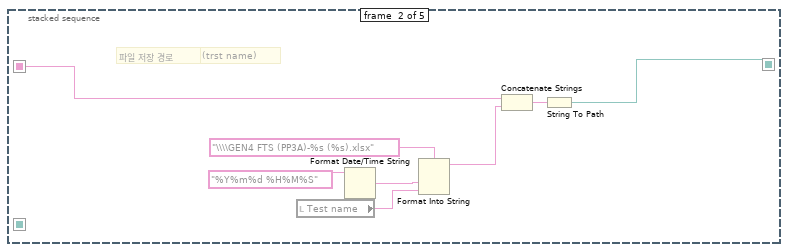
[diagram p14: hidden frame]
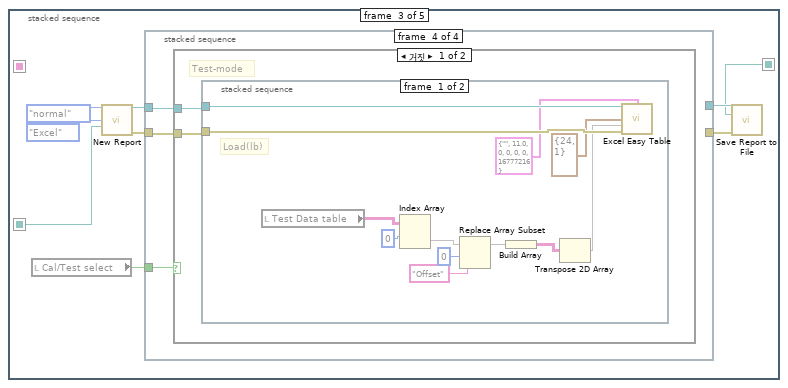
[diagram p15: hidden frame]
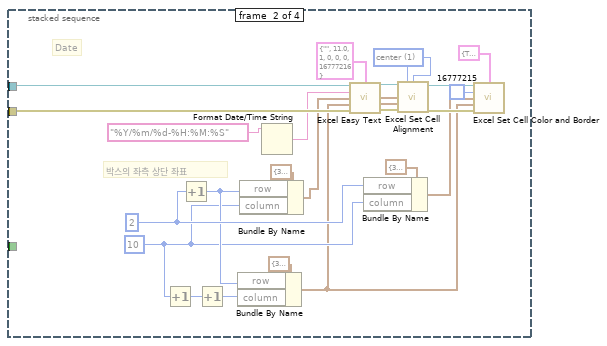
[diagram p17: hidden frame]
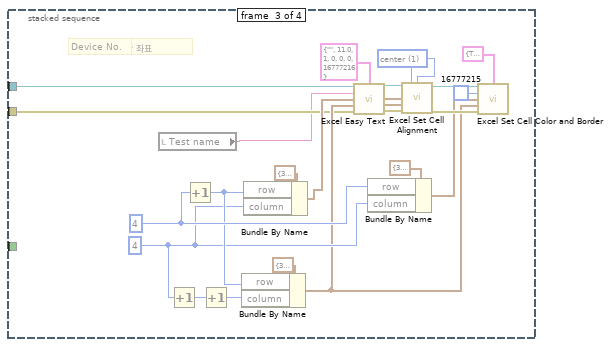
[diagram p18: hidden frame]
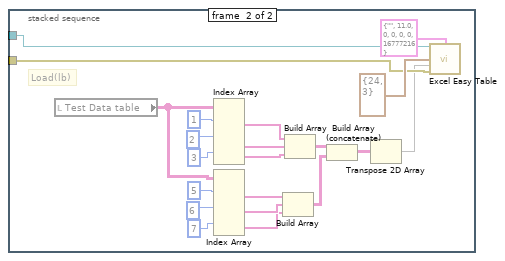
[diagram p19: hidden frame]
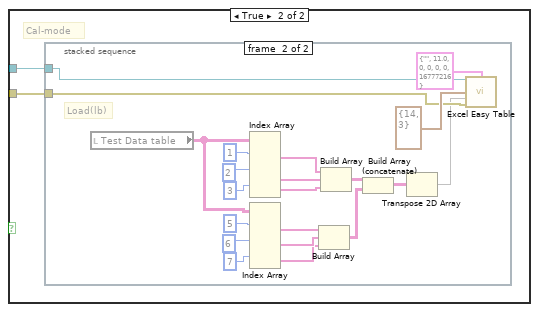
[diagram p20: hidden frame]
diagram:
  n1 = stacked-sequence {
    seq-local: [_ _ _ w142 _ _ _ _ _] -> [_ _ _ _ _ _ _ w1809 _]
    seq-local: [w29 _ _ _ _ _ _ _ _] -> [_ _ _ _ _ _ _ w1805 _]
    frame #0 {
      (unwired) FALSE ("Rx OK")
      # "BLE Buffer Clear"
      # "Local variable"
      n2 = Tick Count (ms)() -> (millisecond timer value=→"ms timer":u32)
      n3 = call "SUB-BLE Rx data Clear.vi"() -> ()  [unwired: 6 in]
      n4 = Tick Count (ms)() -> (millisecond timer value=→"Timer-ble log":u32)
      n5 = control-ref of="탭-Top"() -> (w27:refnum<vi>)
      n6 = control-ref of="Flash Map"() -> (w12:refnum<vi>)
      n7 = local write "log data1"(FALSE ("log data1")) -> ()
      n8 = Build Array(w27, w12) -> (w29:refnum<vi>[])
      n9 = call "Read and Write Controls to Automatic Config File.vi"("Action"=RWC_Actions."Read", "Control References"=w29) -> ()  [unwired: 9 in, 1 out]
      n10 = local write "FTS table index"(0 ("FTS table index")) -> ()
      n11 = local write "Cal/Test select"(TRUE ("Cal select")) -> ()
      n12 = local write "Force Set"(FALSE ("Force Set")) -> ()
      n13 = local write "Load(lb)"(10.0 ("Load(lb)")) -> ()
      n14 = local write "Handle"(u16 16 ("Handle")) -> ()
      n15 = local write "Data(h)"("\u0001" ("Data")) -> ()
      n16 = local write "Head Up"(FALSE ("Head Up")) -> ()
      n17 = local write "Data Log"("" ("Data Log")) -> ()
      n18 = local write "Data_mon(h)"("" ("Data_mon")) -> ()
      n19 = property on="Pane" class="Pane"("Origin"=T16 {"Horizontal"=0, "Vertical"=0} ("원점"), "VertScrollbarVisibility"=T15."Off While Running" ("수직 스크롤 막대 보이기")) -> ()  [unwired: 2 in, 2 out]
      "Rx Cnt" <- 0 ("Rx Cnt")
      "Rx buf 1" <- "" ("Rx 문자열 1")
      "Disconnected" <- FALSE ("Disconnected")
      "Packet Detect" <- FALSE ("Packet Detect")
      "log ble buf" <- "" ("log ble buf")
    }
    frame #1 {
      w53 = 1.0 ("Y 스케일.범위:최대값")
      w59 = T10 {"Gyroscope X"=0.0, "Gyroscope Y"=0.0, "Gyroscope Z"=0.0, "Accelerometer X"=0.0, "Accelerometer Y"=0.0, "Accelerometer Z"=0.0} ("IMU data")
      w60 = T9 {"Left Wing-A, C1/C0"=0.0, "Left Wing-B, C2/C0"=0.0, "Left Wing-C, C3/C0"=0.0, "Right Wing-A, C4/C0"=0.0, "Right Wing-B, C5/C0"=0.0, "Right Wing-C, C6/C0"=0.0} ("CDC data")
      w61 = FALSE ("Offset 1")
      # "Variable initialization"
      n20 = local write "Maximize window"(FALSE ("창크게")) -> ()
      n21 = local write "Setting load(led)"(FALSE ("Power On Flag")) -> ()
      n22 = local write "Comm con 1"(FALSE ("포트 연결")) -> ()
      n23 = local write "Comm con status 1"(FALSE ("Connected")) -> ()
      n24 = local write "Data trx(led)"(FALSE ("Rx")) -> ()
      n25 = local write "ACT-Comm"(FALSE ("ACT-RS422")) -> ()
      n26 = local write "Port open 1"(FALSE) -> ()
      n27 = local write "Port close 1"(FALSE) -> ()
      n28 = local write "status string"("" ("status string")) -> ()
      n29 = local write "*Board ID1"("None...." ("*Board ID")) -> ()
      n30 = local write "stop"(FALSE ("stop")) -> ()
      n31 = local write "Comm err cnt 1"(0 ("통신에러카운트")) -> ()
      n32 = local write "Setting load"(TRUE ("설정값 불러오기")) -> ()
      n33 = local write "Rx-mon"(FALSE) -> ()
      n34 = property on="CDC(PCAP02) Graph" class="WFChart (엄격한)"("History Data"=waveform(dbl)[][] [] ("히스토리 데이터")) -> ()  [unwired: 2 in, 2 out]
      n35 = property on="IMU Graph" class="WFChart (엄격한)"("History Data"=waveform(dbl)[][] [] ("히스토리 데이터")) -> ()  [unwired: 2 in, 2 out]
      n36 = Tick Count (ms)() -> (millisecond timer value=w70:u32)
      n37 = Tick Count (ms)() -> (millisecond timer value=w63:u32)
      n38 = Tick Count (ms)() -> (millisecond timer value=w45:u32)
      n39 = Tick Count (ms)() -> (millisecond timer value=w46:u32)
      n40 = Initialize Array(T17 {"RxOK"=FALSE, "ROM Data"=[], "Index"=0} ("클러스터"), 3 ("차원 크기")) -> (w41:T11)
      n41 = local write "Logging No."(u32 0 ("Logging No.")) -> ()
      n42 = local write "Data Logging"(FALSE ("Data Logging")) -> ()
      n43 = local write "RxD"("" ("RxD")) -> ()
      n44 = local write "Export graph 1"(FALSE ("그래프 반출")) -> ()
      n45 = local write "Full ROM data"(FALSE ("Full ROM data")) -> ()
      n46 = local write "Export graph2"(FALSE ("그래프 반출")) -> ()
      n47 = local write "Offset 1"(w61) -> ()
      n48 = local write "Offset 2"(w61) -> ()
      n49 = local write "Graph timer 1"(w70) -> ()
      n50 = local write "Bat(raw)"(0.0 ("Bat(raw)")) -> ()
      n51 = local write "ROM Data"(w41) -> ()
      n52 = local write "Rx-ROM"(FALSE ("Rx-ROM")) -> ()
      n53 = local write "Clear graph 1"(TRUE ("그래프 지우기")) -> ()
      n54 = local write "Graph timer 2"(w63) -> ()
      n55 = local write "ms timer 2"(w45) -> ()
      n56 = local write "ms timer 3"(w46) -> ()
      n57 = local write "Clear graph 2"(TRUE ("그래프 지우기")) -> ()
      n58 = local write "Rx ROM-log"("" ("문자열-Rx ROM")) -> ()
      n59 = local write "CDC Offet"(w60) -> ()
      n60 = local write "CDC data"(w60) -> ()
      n61 = local write "IMU data"(w59) -> ()
      n62 = local write "IMU Offet"(w59) -> ()
      n63 = local write "BLE Interval Time(ms)"(0.0 ("BLE Interval Time(ms)")) -> ()
      n64 = Tick Count (ms)() -> (millisecond timer value=w38:u32)
      n65 = local write "Test Start"(FALSE ("Test Start")) -> ()
      n66 = property on="BLE Interval buf" class="WFChart (엄격한)"("History Data"=u32[] [] ("히스토리 데이터")) -> ()  [unwired: 2 in, 2 out]
      n67 = local write "ms timer 5"(w38) -> ()
      n68 = property on="BLE Interval Graph" class="WFChart (엄격한)"("History Data"=dbl[] [] ("히스토리 데이터")) -> ()  [unwired: 2 in, 2 out]
      n69 = property on="BLE RSSI buf" class="WFChart (엄격한)"("History Data"=i16[] [] ("히스토리 데이터")) -> ()  [unwired: 2 in, 2 out]
      n70 = local write "BLE RSSI (dBm)"(0.0 ("BLE RSSI (dBm)")) -> ()
      n71 = property on="BLE RSSI Graph" class="WFChart (엄격한)"("History Data"=i16[] [] ("히스토리 데이터")) -> ()  [unwired: 2 in, 2 out]
      n72 = for {
        N: 3 -> [_]
        i -> [w91]
        w92 = 125.0 ("Y 스케일.범위:최대값")
        n73 = Multiply(x=w92, y=-1.0 ("Y 스케일.범위:최대값")) -> (x*y=w94:dbl)
        n74 = property on="IMU Graph" class="WFChart (엄격한)"("ActYScl"=w91, "YScale.Maximum"=w92, "YScale.Minimum"=w94, "YScale.ScaleFit"=u8 0 ("Y 스케일.스케일 맞춤")) -> ()  [unwired: 2 in, 2 out]
      }
      n75 = for {
        N: 3 -> [_]
        i -> [w86]
        w87 = 1.1 ("Y 스케일.범위:최대값")
        n76 = Add(x=w86, y=3.0 ("Y 스케일.범위:최대값")) -> (x+y=w84:dbl)
        n77 = Multiply(x=w87, y=-1.0 ("Y 스케일.범위:최대값")) -> (x*y=w89:dbl)
        n78 = property on="IMU Graph" class="WFChart (엄격한)"("ActYScl"=w84, "YScale.Maximum"=w87, "YScale.Minimum"=w89, "YScale.ScaleFit"=u8 0 ("Y 스케일.스케일 맞춤")) -> ()  [unwired: 2 in, 2 out]
      }
      n79 = Multiply(x=w53, y=-1.0 ("Y 스케일.범위:최대값")) -> (x*y=w52:dbl)
      n80 = property on="CDC(PCAP02) Graph" class="WFChart (엄격한)"("YScale.Maximum"=w53, "YScale.Minimum"=w52, "YScale.ScaleFit"=u8 2 ("Y 스케일.스케일 맞춤")) -> ()  [unwired: 2 in, 2 out]
    }
    frame #2 {
      w100 = "Device ID\t-\t-\nYEAR\t-\t-\nMonth\t-\t-\nDay\t-\t-\nDevice Type\t-\t-\nManufacturer ID\t-\t-\nCal_Scale A\t-\t-\nCal_Scale B\t-\t-\nCal_Acc. X\t-\t-\nCal_Acc. Y\t-\t-\nCal_Acc. Z\t-\t-\nCal_Gy. X\t-\t-\nCal_Gy. Y\t-\t-\nCal_Gy. Z\t-\t-\nCal_Vol H\t-\t-\nCal_Vol L\t-\t-\nCal_CDC Off 1\t-\t-\nCal_CDC Off 2\t-\t-\nCal_CDC Off 3\t-\t-\nCal_CDC Off 4\t-\t-\nCal_CDC Off 5\t-\t-\nCal_CDC Off 6\t-\t-\nCal_CDC Off 7\t-\t-\nCal_CDC Off 8\t-\t-"  # ROM Table-row header
      w107 = "1\n2\n3\n4\n5\n6\n7\n8\n9\n10\n11\n12\n13\n14\n15\n16\n17\n18\n19\n20\n21\n22\n23\n24"  # ROM Table-row index
      w111 = "Name\nValue\nDescriptions"  # ROM Table-col header
      w114 = "Load(1)-0lb\t0\t1000\t0\t0\nInit(1)-70lb\t70\t1000\t0\t0\nInit(2)-140lb\t140\t1000\t0\t0\nInit(1)-70lb\t70\t1000\t0\t0\nInit(2)-140lb\t140\t1000\t0\t0\nLoad(1)-0lb\t0\t10000\t1\t1\nLoad(2)-10lb\t10\t3000\t0\t1\nLoad(3)-20lb\t20\t3000\t0\t1\nLoad(4)-40lb\t40\t3000\t0\t1\nLoad(5)-60lb\t60\t3000\t0\t1\nLoad(6)-80lb\t80\t3000\t0\t1"  # FTS Profile 1
      w119 = "Offset\nLoad(1)-0lb\nLoad(2)-10lb\nLoad(3)-20lb\nLoad(4)-40lb\nLoad(5)-60lb\nLoad(6)-80lb"  # FTS data Table name 1
      # "FTS Profile Init\n(Name, Press, Time)"
      # "col"
      # "Variable initialization"
      n81 = for {
        N: 9 -> [_]
        tunnel: [w130] -> w121 mode=indexing
        # "row"
        n82 = for {
          N: 10 -> [_]
          tunnel: ["-"] -> w130 mode=indexing
        }
      }
      n83 = control-ref of="File path"() -> (w98:refnum<vi>)
      n84 = for {
        N: 7 -> [_]
        i -> [w134]
        n85 = Bundle By Name(cluster=T18 {"Row"=0, "Column"=0} ("활성 셀:활성 셀"), "Row"=0, "Column"=w134) -> (w136:T18)
        n86 = property on="Test Data table" class="Tbl (엄격한)"("Active Cell"=w136, "Width"=u32 80 ("활성 셀:셀 크기:폭")) -> ()  [unwired: 2 in, 2 out]
      }
      n87 = call <vilib>:"Application Directory.vi"() -> ("Application Directory"=w97:path)
      n88 = local write "Mark10 Gauge (lb)"(0.0 ("Mark10 Gauge")) -> ()
      n89 = local write "FTS comm."(FALSE ("FTS 수신 정상")) -> ()
      n90 = local write "Test name"("Noname" ("Test name")) -> ()
      n91 = local write "FTS Testing"(FALSE ("FTS 시험 진행")) -> ()
      n92 = property class="Path"(reference=w98, "Value"=w97) -> ()  [unwired: 1 in, 2 out]
      n93 = local write "FTS OP status"(T7 "Test_Start" ("FTS OP status")) -> ()
      n94 = local write "Test Status"("" ("Force Test Status")) -> ()
      n95 = call "SUB-module-StringToArray.vi"("String"="Mark10 Gauge(lb)\nLeft Wing-A\nLeft Wing-B\nLeft Wing-C\nLeft Wing-SUM\nRight Wing-A\nRight Wing-B\nRight Wing-C\nRight Wing-SUM" ("문자열")) -> ("Arrary"=w116:string[])
      n96 = local write "Load Graph"(cluster{dbl[], dbl[]} {[], []} ("Load Graph")) -> ()
      n97 = local write "Test Data table"(w121) -> ()
      n98 = property on="Test Data table" class="Tbl (엄격한)"("Row Headers[]"=w116) -> ()  [unwired: 2 in, 2 out]
      n99 = Generate Occurrence() -> (→"Disconnection ocurrence":refnum<k4>)
      n100 = call "SUB-module-StringToArray.vi"("String"=w119) -> ("Arrary"=w118:string[])
      n101 = Spreadsheet String To Array(format string="%s" ("포맷 문자열"), spreadsheet string=w114, array type (2D Dbl)=string[][] [] ("배열 타입(2D Dbl)")) -> (array=w125:string[][])  [unwired: 1 in]
      n102 = Spreadsheet String To Array(delimiter (Tab)="\n", format string="%s" ("포맷 문자열"), spreadsheet string=w111, array type (2D Dbl)=string[] [] ("배열 타입(2D Dbl)")) -> (array=w110:string[])
      n103 = Spreadsheet String To Array(delimiter (Tab)="\n", format string="%s" ("포맷 문자열"), spreadsheet string=w107, array type (2D Dbl)=string[] [] ("배열 타입(2D Dbl)")) -> (array=w106:string[])
      n104 = Spreadsheet String To Array(format string="%s" ("포맷 문자열"), spreadsheet string=w100, array type (2D Dbl)=string[][] [] ("배열 타입(2D Dbl)")) -> (array=w101:string[][])  [unwired: 1 in]
      n105 = property on="Test Data table" class="Tbl (엄격한)"("Column Headers[]"=w118) -> ()  [unwired: 2 in, 2 out]
      n106 = local write "Test profile"(w125) -> ()
      n107 = property on="ROM Table" class="Tbl (엄격한)"("Column Headers[]"=w110, "Row Headers[]"=w106, "Value"=w101) -> ()  [unwired: 2 in, 2 out]
    }
    frame #3 {
      # "Program configration is loaded from file."
      n108 = call "SUB-module-Current VI Path.vi"() -> ("현재 VI 경로"=w143:path)
      n109 = Path To String(path=w143) -> (string=w145:string)
      n110 = Concatenate Strings(w145, "\\Configuration File.ini") -> (w144:string)
      n111 = String To Path(string=w144) -> (path=w142:path)
      n112 = call <vilib>:"Open Config Data.vi"("create file if necessary (T)"=TRUE, "configuration file path"=w142) -> ("error out"=w149:errorcluster, "refnum"=w148:T30)  [unwired: 7 in, 1 out]
      n113 = stacked-sequence {
        tunnel: w148 -> [w156 w158 w164 w171 w176]
        tunnel: w149 -> [w155 w157 w163 w170 w175]
        tunnel: "GUI Setting" ("section") -> [w154 w159 w165 w172 _]
        tunnel: [_ _ _ _ w176] -> w140
        tunnel: [_ _ _ _ w175] -> w139
        frame #0 {
          w153 = "Com Port-Board1"  # Key 1
          n114 = call-poly <vilib>:"Read Key.vi"("section"=w154, "error in (no error)"=w155, "default value"="COM4" ("output string"), "key"=w153, "refnum"=w156) -> ("value"=w152:string)  [unwired: 3 in, 3 out]
          n115 = local write "Port-set 1"(w152) -> ()
        }
        frame #1 {
          w162 = "Com Port-FTS"  # Key 1
          n116 = call-poly <vilib>:"Read Key.vi"("section"=w159, "error in (no error)"=w157, "default value"="COM5" ("output string"), "key"=w162, "refnum"=w158) -> ("value"=w161:string)  [unwired: 3 in, 3 out]
          n117 = local write "Port-FTS"(w161) -> ()
        }
        frame #2 {
          w168 = "Logno"  # Key 1
          n118 = call-poly <vilib>:"Read Key.vi"("section"=w165, "error in (no error)"=w163, "default value"="1" ("output string"), "key"=w168, "refnum"=w164) -> ("value"=w167:string)  [unwired: 3 in, 3 out]
          n119 = local write "Log no"(w167) -> ()
        }
        frame #3 {
          w174 = "Interval(ms)"  # Key 1
          n120 = call-poly <vilib>:"Read Key.vi"("section"=w172, "error in (no error)"=w170, "default value"=100, "key"=w174, "refnum"=w171) -> ("value"=w173:i32)  [unwired: 3 in, 3 out]
          n121 = local write "Update(ms)"(w173) -> ()
        }
        frame #4 {
        }
      }
      n122 = local write "status string"("Program settings Loading..." ("status string")) -> ()
      n123 = call <vilib>:"Close Config Data.vi"("error in (no error)"=w139, "write file if changed (T)"=FALSE ("write configuration file? (T)"), "refnum"=w140) -> ()  [unwired: 9 out]
    }
    frame #4 {
      n124 = disable-structure shown="활성화" {
        frame Disabled {
          n125 = flat-sequence {
            frame #0 {
              w180 = "0\t0\t9.95\t20.05\t40\n29986.8\t-2.7\t33.7\t79.3\t165.5\n29908\t0.3\t45.2\t83\t176\n26231.9\t-0.1\t61.1\t114.7\t228.4\n-\t-2.4\t140.1\t277.1\t570\n54111.4\t-0.6\t65\t121\t239.8\n52947.4\t0.6\t92.3\t133.4\t231.5\n39809.3\t2.3\t73.1\t101.9\t183.1\n-\t2.4\t230.5\t356.4\t654.5\n"  # FTS data Table name 1
              n126 = Spreadsheet String To Array(format string="%s" ("포맷 문자열"), spreadsheet string=w180, array type (2D Dbl)=string[][] [] ("배열 타입(2D Dbl)")) -> (array=w179:string[][])  [unwired: 1 in]
              n127 = local write "Cal/Test select"(FALSE ("Cal/Test select")) -> ()
              n128 = local write "Test Data table"(w179) -> ()
            }
            frame #1 {
              n129 = stacked-sequence {
                seq-local: [_ w201 _ _ _] -> [_ _ w210 _ _]
                seq-local: [w189 _ _ _ _] -> [_ w200 _ _ _]
                seq-local: [w183 _ _ _ _] -> [_ _ w209 _ _]
                frame #0 {
                  w197 = T31 1 items=["사용자 홈"=0, "사용자 데스크탑"=1, "사용자 문서"=2, "사용자 어플리케이션 데이터"=3, "사용자 환경"=4, "사용자 임시"=5, "퍼블릭 문서"=6, "퍼블릭 어플리케이션 데이터"=7, "퍼블릭 환경"=8, "퍼블릭 캐시"=13, "시스템 코어 라이브러리"=9, "시스템 설치된 라이브러리"=10, "어플리케이션 파일"=11, "부팅 볼륨 루트"=12] ("system directory type")
                  n130 = call "SUB-module-Current VI Path.vi"() -> ("현재 VI 경로"=w186:path)
                  n131 = call <vilib>:"Get System Directory.vi"("system directory type"=w197) -> ("system directory"=w196:path)  [unwired: 10 in]
                  n132 = Path To String(path=w186) -> (string=w185:string)
                  n133 = Path To String(path=w196) -> (string=w195:string)
                  n134 = Concatenate Strings(w185, "\\Template" ("이름 또는 상대 경로"), "\\GEN4 FTS Test Report rev1.xlsx" ("이름 또는 상대 경로")) -> (w184:string)
                  n135 = String To Path(string=w184) -> (path=w183:path)
                  n136 = Concatenate Strings(w195, "\\GEN4-GUI Test data" ("상태")) -> (w189:string)
                  n137 = String To Path(string=w189) -> (path=w193:path)
                  n138 = call <vilib>:"Check if File or Folder Exists.vi"("path"=w193) -> ("error out"=w190:errorcluster, "file or folder exists?"=w192:bool, "dup path"=w191:path)  [unwired: 8 in]
                  n139 = case shown="거짓" w192 {
                    tunnel: w191 -> [w199 _]
                    tunnel: w190 -> [w198 _]
                    frame False {
                      n140 = Create Folder(path (use dialog)=w199, error in=w198) -> ()  [unwired: 1 in, 3 out]
                    }
                    frame True {
                    }
                  }
                }
                frame #1 {
                  # "* 파일명(rev)-date (trst name)"
                  # "파일 저장 경로"
                  n141 = local read "Test name"() -> (w206:string)
                  n142 = Format Date/Time String(time format string (%c)="%Y%m%d %H%M%S" ("상태")) -> (date/time string=w205:string)  [unwired: 2 in]
                  n143 = Format Into String(format string="\\\\GEN4 FTS (PP3A)-%s (%s).xlsx" ("상태"), w205, w206) -> (resulting string=w202:string)  [unwired: 2 in, 1 out]
                  n144 = Concatenate Strings(w200, w202) -> (w207:string)
                  n145 = String To Path(string=w207) -> (path=w201:path)
                }
                frame #2 {
                  n146 = local read "Cal/Test select"() -> (w208:bool)
                  n147 = call <vilib>:"New Report.vi"("window state (normal)"=T20."normal", "report type"=T19."Excel", "template (empty)"=w209) -> ("report out"=w213:refnum<class "NI_report.lvclass">, "error out"=w214:errorcluster)  [unwired: 11 in]
                  n148 = stacked-sequence {
                    tunnel: w213 -> [w218 w243 w245 w270]
                    tunnel: w214 -> [w217 w242 w246 w269]
                    tunnel: [w218 _ _ _] -> w216
                    tunnel: [w217 _ _ _] -> w215
                    tunnel: w208 -> [_ _ _ w268]
                    frame #0 {
                    }
                    frame #1 {
                      w221 = 10 ("column")
                      w228 = 2 ("row")
                      w235 = 1 items=["top", "center", "bottom"] ("vertical alignment (top)")
                      # "Date"
                      # "박스의 좌측 상단 좌표"
                      n149 = Increment(x=w221) -> (x+1=w220:i32)
                      n150 = Increment(x=w228) -> (x+1=w223:i32)
                      n151 = Increment(x=w220) -> (x+1=w222:i32)
                      n152 = Bundle By Name(cluster=cluster{"row":i32, "column":i32} {"row"=3, "column"=10} ("start (-1, -1)"), "row"=w223, "column"=w222) -> (w219:cluster{"row":i32, "column":i32})
                      n153 = Bundle By Name(cluster=cluster{"row":i32, "column":i32} {"row"=3, "column"=10} ("start (-1, -1)"), "row"=w223, "column"=w221) -> (w229:cluster{"row":i32, "column":i32})
                      n154 = Format Date/Time String(time format string (%c)="%Y/%m/%d-%H:%M:%S" ("상태")) -> (date/time string=w241:string)  [unwired: 2 in]
                      n155 = call <vilib>:"Excel Easy Text.vi"("report in"=w243, "font"=T21 {"font name"="", "font size"=11.0, "bold"=1, "italic"=0, "underline"=0, "strike through"=0, "font color"=16777216}, "text"=w241, "start (-1, -1)"=w229, "end (-1, -1)"=w219, "error in (no error)"=w242) -> ("report out"=w239:refnum<class "NI_report.lvclass">, "next cell bottom-left"=w237:cluster{"row":i32, "column":i32}, "next cell top-right"=w236:cluster{"row":i32, "column":i32}, "error out"=w238:errorcluster)  [unwired: 5 in, 1 out]
                      n156 = Bundle By Name(cluster=cluster{"row":i32, "column":i32} {"row"=3, "column"=10} ("start (-1, -1)"), "row"=w228, "column"=w221) -> (w227:cluster{"row":i32, "column":i32})
                      n157 = call <vilib>:"Excel Set Cell Alignment.vi"("report in"=w239, "vertical alignment (top)"=w235, "horizontal alignment (left)"=w235, "start (-1, -1)"=w237, "end (-1, -1)"=w236, "error in (no error)"=w238) -> ("report out"=w234:refnum<class "NI_report.lvclass">, "error out"=w233:errorcluster)  [unwired: 8 in]
                      n158 = call <vilib>:"Excel Set Cell Color and Border.vi"("report in"=w234, "outside border"=T22 {"on/off"=TRUE, "weight"=2, "color"=0}, "background color (w)"=u32 16777215, "start (-1, -1)"=w227, "end (-1, -1)"=w219, "error in (no error)"=w233) -> ()  [unwired: 8 in, 2 out]
                    }
                    frame #2 {
                      w249 = 4 ("column")
                      w256 = 4 ("row")
                      w263 = 1 items=["top", "center", "bottom"] ("vertical alignment (top)")
                      # "Device No."
                      # "박스의 좌측 상단 좌표"
                      n159 = local read "Test name"() -> (w244:string)
                      n160 = Increment(x=w249) -> (x+1=w248:i32)
                      n161 = Increment(x=w256) -> (x+1=w251:i32)
                      n162 = Increment(x=w248) -> (x+1=w250:i32)
                      n163 = Bundle By Name(cluster=cluster{"row":i32, "column":i32} {"row"=3, "column"=10} ("start (-1, -1)"), "row"=w251, "column"=w250) -> (w247:cluster{"row":i32, "column":i32})
                      n164 = Bundle By Name(cluster=cluster{"row":i32, "column":i32} {"row"=3, "column"=10} ("start (-1, -1)"), "row"=w251, "column"=w249) -> (w257:cluster{"row":i32, "column":i32})
                      n165 = call <vilib>:"Excel Easy Text.vi"("report in"=w245, "font"=T21 {"font name"="", "font size"=11.0, "bold"=1, "italic"=0, "underline"=0, "strike through"=0, "font color"=16777216}, "text"=w244, "start (-1, -1)"=w257, "end (-1, -1)"=w247, "error in (no error)"=w246) -> ("report out"=w267:refnum<class "NI_report.lvclass">, "next cell bottom-left"=w265:cluster{"row":i32, "column":i32}, "next cell top-right"=w264:cluster{"row":i32, "column":i32}, "error out"=w266:errorcluster)  [unwired: 5 in, 1 out]
                      n166 = Bundle By Name(cluster=cluster{"row":i32, "column":i32} {"row"=3, "column"=10} ("start (-1, -1)"), "row"=w256, "column"=w249) -> (w255:cluster{"row":i32, "column":i32})
                      n167 = call <vilib>:"Excel Set Cell Alignment.vi"("report in"=w267, "vertical alignment (top)"=w263, "horizontal alignment (left)"=w263, "start (-1, -1)"=w265, "end (-1, -1)"=w264, "error in (no error)"=w266) -> ("report out"=w262:refnum<class "NI_report.lvclass">, "error out"=w261:errorcluster)  [unwired: 8 in]
                      n168 = call <vilib>:"Excel Set Cell Color and Border.vi"("report in"=w262, "outside border"=T22 {"on/off"=TRUE, "weight"=2, "color"=0}, "background color (w)"=u32 16777215, "start (-1, -1)"=w255, "end (-1, -1)"=w247, "error in (no error)"=w261) -> ()  [unwired: 8 in, 2 out]
                    }
                    frame #3 {
                      n169 = case shown="거짓" w268 {
                        tunnel: w270 -> [w272 w307]
                        tunnel: w269 -> [w271 w306]
                        frame False {
                          # "Test-mode"
                          n170 = stacked-sequence {
                            tunnel: w272 -> [w284 w303]
                            tunnel: w271 -> [w283 w302]
                            frame #0 {
                              # "Load(lb)"
                              n171 = local read "Test Data table"() -> (w282:string[][])
                              n172 = Index Array(array=w282, index (row)=0 ("인덱스 (행)")) -> (element=w279:string[])  [unwired: 1 in]
                              n173 = Replace Array Subset(array=w279, new element="Offset" ("새 원소/부분배열"), index=0 ("인덱스")) -> (w276:string[])
                              n174 = Build Array(w276) -> (w275:string[][])
                              n175 = Transpose 2D Array(2D array=w275) -> (transposed array=w274:string[][])
                              n176 = call-poly <vilib>:"Excel Easy Table.vi"("report in"=w284, "font"=T21 {"font name"="", "font size"=11.0, "bold"=0, "italic"=0, "underline"=0, "strike through"=0, "font color"=16777216}, "start (0, 0)"=cluster{"row":i32, "column":i32} {"row"=24, "column"=1}, "text data"=w274, "error in (no error)"=w283) -> ()  [unwired: 6 in, 5 out]
                            }
                            frame #1 {
                              # "Load(lb)"
                              n177 = local read "Test Data table"() -> (w296:string[][])
                              n178 = Index Array(array=w296, index (row) #1=1 ("인덱스 (행)"), index (row) #2=2 ("인덱스 (행)"), index (row) #3=3 ("인덱스 (행)")) -> (element #1=w295:string[], element #2=w294:string[], element #3=w293:string[])  [unwired: 3 in]
                              n179 = Index Array(array=w296, index (row) #1=5 ("인덱스 (행)"), index (row) #2=6 ("인덱스 (행)"), index (row) #3=7 ("인덱스 (행)")) -> (element #1=w292:string[], element #2=w291:string[], element #3=w290:string[])  [unwired: 3 in]
                              n180 = Build Array(w292, w291, w290) -> (w288:string[][])
                              n181 = Build Array(w295, w294, w293) -> (w289:string[][])
                              n182 = Build Array (concatenate)(w289, w288) -> (w287:string[][])
                              n183 = Transpose 2D Array(2D array=w287) -> (transposed array=w286:string[][])
                              n184 = call-poly <vilib>:"Excel Easy Table.vi"("report in"=w303, "font"=T21 {"font name"="", "font size"=11.0, "bold"=0, "italic"=0, "underline"=0, "strike through"=0, "font color"=16777216}, "start (0, 0)"=cluster{"row":i32, "column":i32} {"row"=24, "column"=3}, "text data"=w286, "error in (no error)"=w302) -> ()  [unwired: 6 in, 5 out]
                            }
                          }
                        }
                        frame True {
                          # "Cal-mode"
                          n185 = stacked-sequence {
                            tunnel: w307 -> [w319 w338]
                            tunnel: w306 -> [w318 w337]
                            frame #0 {
                              # "Load(lb)"
                              n186 = local read "Test Data table"() -> (w317:string[][])
                              n187 = Index Array(array=w317, index (row)=0 ("인덱스 (행)")) -> (element=w314:string[])  [unwired: 1 in]
                              n188 = Replace Array Subset(array=w314, new element="Offset" ("새 원소/부분배열"), index=0 ("인덱스")) -> (w311:string[])
                              n189 = Build Array(w311) -> (w310:string[][])
                              n190 = Transpose 2D Array(2D array=w310) -> (transposed array=w309:string[][])
                              n191 = call-poly <vilib>:"Excel Easy Table.vi"("report in"=w319, "font"=T21 {"font name"="", "font size"=11.0, "bold"=0, "italic"=0, "underline"=0, "strike through"=0, "font color"=16777216}, "start (0, 0)"=cluster{"row":i32, "column":i32} {"row"=14, "column"=1}, "text data"=w309, "error in (no error)"=w318) -> ()  [unwired: 6 in, 5 out]
                            }
                            frame #1 {
                              # "Load(lb)"
                              n192 = local read "Test Data table"() -> (w331:string[][])
                              n193 = Index Array(array=w331, index (row) #1=1 ("인덱스 (행)"), index (row) #2=2 ("인덱스 (행)"), index (row) #3=3 ("인덱스 (행)")) -> (element #1=w330:string[], element #2=w329:string[], element #3=w328:string[])  [unwired: 3 in]
                              n194 = Index Array(array=w331, index (row) #1=5 ("인덱스 (행)"), index (row) #2=6 ("인덱스 (행)"), index (row) #3=7 ("인덱스 (행)")) -> (element #1=w327:string[], element #2=w326:string[], element #3=w325:string[])  [unwired: 3 in]
                              n195 = Build Array(w327, w326, w325) -> (w323:string[][])
                              n196 = Build Array(w330, w329, w328) -> (w324:string[][])
                              n197 = Build Array (concatenate)(w324, w323) -> (w322:string[][])
                              n198 = Transpose 2D Array(2D array=w322) -> (transposed array=w321:string[][])
                              n199 = call-poly <vilib>:"Excel Easy Table.vi"("report in"=w338, "font"=T21 {"font name"="", "font size"=11.0, "bold"=0, "italic"=0, "underline"=0, "strike through"=0, "font color"=16777216}, "start (0, 0)"=cluster{"row":i32, "column":i32} {"row"=14, "column"=3}, "text data"=w321, "error in (no error)"=w337) -> ()  [unwired: 6 in, 5 out]
                            }
                          }
                        }
                      }
                    }
                  }
                  n200 = call-dynamic "Save Report to File.vi"("report in"=w216, "report file path"=w210, "error in (no error)"=w215) -> ()  [unwired: 11 in, 2 out]
                }
                frame #3 {
                }
                frame #4 {
                }
              }
            }
            frame #2 {
              n201 = Stop(stop? (T)=TRUE ("정지? (참)")) -> ()
            }
          }
        }
        frame Enabled {
        }
      }
      n202 = call "SUB_Delay ms.vi"("delay(ms)"=u32 100 ("ms 타이머 값")) -> ()  [unwired: 3 in]
    }
    frame #5 {
      # "Main Loop"
      n203 = while {
        i -> [w571]
        stop <- w573 stop-if-true
        n204 = stacked-sequence {
          tunnel: w571 -> [_ w646 _ _ _ _ _ _ _ _ _ _ _ _ _ _]
          frame #0 {
            # "Connection of Communication - BLE"
            n205 = local read "Port close 1"() -> (w574:bool)
            n206 = local read "Port open 1"() -> (w575:bool)
            n207 = case shown="참" w575 {
              frame False {
              }
              frame True {
                # "Connection of Communication"
                n208 = stacked-sequence {
                  frame #0 {
                    # "BLE Buffer Clear"
                    # "Initialize"
                    n209 = call "SUB-BLE Rx data Clear.vi"() -> ()  [unwired: 6 in]
                    n210 = Tick Count (ms)() -> (millisecond timer value=w577:u32)
                    n211 = local write "ACT-Comm"(TRUE ("ACT-RS422")) -> ()
                    n212 = local write "Full ROM data"(FALSE ("Full ROM data")) -> ()
                    n213 = local write "Port open 1"(FALSE) -> ()
                    n214 = Initialize Array(T17 {"RxOK"=FALSE, "ROM Data"=[], "Index"=0} ("클러스터"), 3 ("차원 크기")) -> (w581:T11)
                    n215 = local write "Data trx(led)"(TRUE ("Rx")) -> ()
                    n216 = local write "Rx ROM-log"("" ("문자열-Rx ROM")) -> ()
                    n217 = local write "Timer-ble log"(w577) -> ()
                    n218 = local write "ROM Data"(w581) -> ()
                    n219 = local write "status string"("Communication connection attempt.." ("status string")) -> ()
                  }
                  frame #1 {
                    n220 = local read "Port-set 1"() -> (w589:refnum<visa-resource-name>)
                    n221 = call "_Serial Port-Initialize.vi"("baud rate"=u32 115200, "Serial Port"=w589) -> ("Serial Port 2"=w587:refnum<visa-resource-name>, "Normal"=w591:bool)  [unwired: 2 in]
                    n222 = local write "Port-act 1"(w589) -> ()
                    n223 = call "SUB_Write_GEN4_Init_data_V2_0_1.vi"("Mode"=enum16{"Save Flash", "Visa save"}."Visa save", "Port-act 1"=w589) -> ()  [unwired: 10 in]
                    n224 = VISA Close(VISA resource name=w587) -> (error out=w586:errorcluster)  [unwired: 1 in]
                    n225 = case shown="참" w591 {
                      tunnel: w589 -> [_ w600]
                      tunnel: w586 -> [_ _]
                      frame False {
                        n226 = local write "Comm con status 1"(FALSE ("Connected")) -> ()
                        n227 = local write "Comm con 1"(FALSE ("보드 통신 연결 1")) -> ()
                        n228 = local write "Rx-mon"(TRUE ("수신 실패(T) 2")) -> ()
                        n229 = local write "RxD"("Can not find COM port" ("status string")) -> ()
                      }
                      frame True {
                        n230 = call "SUB-BLE SCAN.vi"("Port-set 1"=w600) -> ("Device Name"=→"Device Name":string, "Connection Status"=w596:T5, "Connected"=w599:bool)  [unwired: 2 in]
                        "Connection Status" <- w596
                        n231 = Not(x=w599) -> (.not. x?=w598:bool)
                        n232 = local write "Rx-mon"(w598) -> ()
                        n233 = case shown="거짓" w598 {
                          tunnel: w596 -> [_ w608]
                          frame True {
                            # "수신 데이터 에러 상태"
                            n234 = local read "Port-act 1"() -> (w604:refnum<visa-resource-name>)
                            n235 = VISA Close(VISA resource name=w604) -> ()  [unwired: 1 in, 1 out]
                            n236 = local write "Comm con status 1"(FALSE ("Connected")) -> ()
                            n237 = local write "*Board ID1"("None...." ("*Board ID")) -> ()
                            n238 = local write "Comm con 1"(FALSE ("보드 통신 연결 1")) -> ()
                            n239 = local write "Rx-mon"(TRUE ("수신 실패(T) 2")) -> ()
                          }
                          frame False {
                            w610 = T9 {"Left Wing-A, C1/C0"=0.0, "Left Wing-B, C2/C0"=0.0, "Left Wing-C, C3/C0"=0.0, "Right Wing-A, C4/C0"=0.0, "Right Wing-B, C5/C0"=0.0, "Right Wing-C, C6/C0"=0.0} ("CDC data")
                            w609 = T10 {"Gyroscope X"=0.0, "Gyroscope Y"=0.0, "Gyroscope Z"=0.0, "Accelerometer X"=0.0, "Accelerometer Y"=0.0, "Accelerometer Z"=0.0} ("IMU data")
                            # "Received data normal"
                            n240 = stacked-sequence {
                              tunnel: w608 -> [_ w624 w625 _]
                              frame #0 {
                                # "BLE 버퍼 클리어"
                                n241 = call "SUB-BLE Rx data Clear.vi"() -> ()  [unwired: 6 in]
                                n242 = Wait Until Next ms Multiple(millisecond multiple=u32 500 ("ms 타이머 값")) -> ()  [unwired: 1 out]
                              }
                              frame #1 {
                                # "Data transmission\n- Handle/0x01"
                                n243 = local read "Port-act 1"() -> (w623:refnum<visa-resource-name>)
                                n244 = Tick Count (ms)() -> (millisecond timer value=w622:u32)
                                n245 = Build Array(u16 1 ("Handle")) -> (w621:u16[])
                                n246 = local write "ms timer 4"(w622) -> ()
                                n247 = call-poly "ble_write_by_handle.vi"("Connection Status"=w624, "Handle"=u16 12, "data (uint8array)"=w621, "COM Bluegiga in"=w623) -> ()  [unwired: 6 in, 2 out]
                              }
                              frame #2 {
                                # "데이터 전송\n- 핸들/0x01"
                                n248 = local read "Port-act 1"() -> (w630:refnum<visa-resource-name>)
                                n249 = Tick Count (ms)() -> (millisecond timer value=w629:u32)
                                n250 = Build Array(u16 1 ("Handle")) -> (w628:u16[])
                                n251 = local write "ms timer 4"(w629) -> ()
                                n252 = call-poly "ble_write_by_handle.vi"("Connection Status"=w625, "Handle"=u16 16, "data (uint8array)"=w628, "COM Bluegiga in"=w630) -> ()  [unwired: 6 in, 2 out]
                              }
                              frame #3 {
                                n253 = local write "Comm con status 1"(TRUE ("Connected")) -> ()
                              }
                            }
                            n254 = local write "*Board ID1"("" ("*Board ID")) -> ()
                            n255 = local write "RxD"("Connection. OK....." ("status string")) -> ()
                            n256 = local write "Setting load(led)"(FALSE ("Power On Flag")) -> ()
                            n257 = local write "Comm err cnt 1"(0 ("통신에러카운트")) -> ()
                            n258 = local write "Clear graph 1"(TRUE ("그래프 지우기")) -> ()
                            n259 = local write "Clear graph 2"(TRUE ("그래프 지우기")) -> ()
                            n260 = local write "Data Log"("" ("Data Log")) -> ()
                            n261 = local write "Data_mon(h)"("" ("Data_mon")) -> ()
                            n262 = local write "Comm con 1"(TRUE ("포트 연결")) -> ()
                            n263 = local write "CDC Offet"(w610) -> ()
                            n264 = local write "CDC data"(w610) -> ()
                            n265 = local write "IMU data"(w609) -> ()
                            n266 = local write "IMU Offet"(w609) -> ()
                          }
                        }
                      }
                    }
                  }
                  frame #2 {
                    n267 = local write "ACT-Comm"(FALSE ("ACT-RS422")) -> ()
                    n268 = local write "Data trx(led)"(FALSE ("Rx")) -> ()
                  }
                }
              }
            }
            n269 = case shown="참" w574 {
              frame False {
              }
              frame True {
                # "END of BLE Communication"
                # "포트 닫기"
                n270 = local write "Port close 1"(FALSE ("포트닫기 1")) -> ()
                n271 = local write "Comm con status 1"(FALSE ("Connected")) -> ()
                n272 = local write "*Board ID1"("None...." ("*Board ID")) -> ()
                n273 = local write "ACT-Comm"(FALSE ("ACT-RS422")) -> ()
                n274 = local write "status string"("Close communication port." ("status string")) -> ()
                n275 = local write "Comm con 1"(FALSE ("보드 통신 연결 1")) -> ()
                n276 = local read "Port-act 1"() -> (w634:refnum<visa-resource-name>)
                n277 = local read "Connection Status"() -> (w639:T5)
                n278 = call "_Serial_buf clear.vi"("Serial Port"=w634) -> ("에러 출력"=w637:errorcluster, "Serial Port 2"=w638:refnum<visa-resource-name>)  [unwired: 3 in]
                n279 = call "ble_disconnect_device.vi"("Connection Status"=w639, "error in (no error)"=w637, "COM Bluegiga in"=w638) -> ("error out"=w636:errorcluster, "COM Bluegiga out"=w635:refnum<visa-resource-name>)  [unwired: 7 in]
                n280 = VISA Close(VISA resource name=w635, error in (no error)=w636) -> ()  [unwired: 1 out]
              }
            }
          }
          frame #1 {
            # "#BLE_Packet_data_process"
            # "BLE RX Packet data processing"
            n281 = local read "Comm con status 1"() -> (w647:bool)
            n282 = case shown="참" w647 {
              tunnel: w646 -> [_ w653]
              frame False {
              }
              frame True {
                w656 = 80 ("y")
                n283 = call "SUB-BLE Rx data (Mon)-Classify.vi"() -> ("data out"=w652:u8[], "Rx-set"=w650:bool, "Rx-debug"=w649:bool, "Rx-mon"=w651:bool, "Packet No."=w648:i32)  [unwired: 5 in]
                n284 = local write "Packet No."(w648) -> ()
                n285 = stacked-sequence {
                  tunnel: w652 -> [w660 w680 w701]
                  tunnel: w651 -> [w659 _ _]
                  tunnel: w650 -> [_ _ w702]
                  tunnel: w649 -> [_ w681 _]
                  frame #0 {
                    # "Monitoring Data"
                    n286 = case shown="참" w659 {
                      tunnel: w660 -> [_ w667]
                      frame False {
                      }
                      frame True {
                        # "Monitoring data reception complete"
                        n287 = local read "ms timer"() -> (w676:u32)
                        n288 = local write "Rx-mon"(TRUE ("Rx-mon")) -> ()
                        n289 = local write "Rx-ROM"(FALSE ("Rx-ROM")) -> ()
                        n290 = local write "Rx-debug"(FALSE ("Rx-debug")) -> ()
                        n291 = Tick Count (ms)() -> (millisecond timer value=w675:u32)
                        n292 = call <vilib>:"Space Constant.vi"() -> ("String"=w670:string)
                        n293 = Subtract(x=w675, y=w676) -> (x-y=w673:u32)
                        n294 = local write "BLE Packet (mon)"(w667) -> ()
                        n295 = Array To Spreadsheet String(delimiter (Tab)=w670, array=w667, 3:"%02X" ("포맷 문자열")) -> (spreadsheet string=w668:string)
                        n296 = local write "ms timer"(w675) -> ()
                        n297 = local write "status string"("Receive a monitoring data..." ("status string")) -> ()
                        n298 = Format Into String(format string="[%d ms] " ("포맷 문자열"), w673) -> (resulting string=w672:string)  [unwired: 2 in, 1 out]
                        n299 = local read "ms timer 2"() -> (w664:u32)
                        n300 = Tick Count (ms)() -> (millisecond timer value=w663:u32)
                        n301 = Concatenate Strings(w672, w668) -> (w671:string)
                        n302 = Subtract(x=w663, y=w664) -> (x-y=w662:u32)
                        n303 = case shown="150.." w662 {
                          tunnel: w671 -> [_ w679]
                          frame 0, Default {
                          }
                          frame 150.. {
                            n304 = Tick Count (ms)() -> (millisecond timer value=w678:u32)
                            n305 = local write "RxD"(w679) -> ()
                            n306 = local write "ms timer 2"(w678) -> ()
                          }
                        }
                      }
                    }
                  }
                  frame #1 {
                    # "Debugging Data"
                    n307 = case shown="참" w681 {
                      tunnel: w680 -> [_ w688]
                      frame False {
                      }
                      frame True {
                        # "debugging Data reception complete"
                        n308 = local read "ms timer"() -> (w697:u32)
                        n309 = local write "Rx-mon"(FALSE ("Rx-mon")) -> ()
                        n310 = local write "Rx-ROM"(FALSE ("Rx-ROM")) -> ()
                        n311 = local write "Rx-debug"(TRUE ("Rx-debug")) -> ()
                        n312 = Tick Count (ms)() -> (millisecond timer value=w696:u32)
                        n313 = call <vilib>:"Space Constant.vi"() -> ("String"=w691:string)
                        n314 = Subtract(x=w696, y=w697) -> (x-y=w694:u32)
                        n315 = local write "BLE Packet (mon)"(w688) -> ()
                        n316 = Array To Spreadsheet String(delimiter (Tab)=w691, array=w688, 3:"%02X" ("포맷 문자열")) -> (spreadsheet string=w689:string)
                        n317 = local write "ms timer"(w696) -> ()
                        n318 = local write "status string"("Receive a debugging data..." ("status string")) -> ()
                        n319 = Format Into String(format string="[%d ms] " ("포맷 문자열"), w694) -> (resulting string=w693:string)  [unwired: 2 in, 1 out]
                        n320 = local read "ms timer 2"() -> (w685:u32)
                        n321 = Tick Count (ms)() -> (millisecond timer value=w684:u32)
                        n322 = Concatenate Strings(w693, w689) -> (w692:string)
                        n323 = Subtract(x=w684, y=w685) -> (x-y=w683:u32)
                        n324 = case shown="150.." w683 {
                          tunnel: w692 -> [_ w700]
                          frame 0, Default {
                          }
                          frame 150.. {
                            n325 = Tick Count (ms)() -> (millisecond timer value=w699:u32)
                            n326 = local write "RxD"(w700) -> ()
                            n327 = local write "ms timer 2"(w699) -> ()
                          }
                        }
                      }
                    }
                  }
                  frame #2 {
                    # "Init data"
                    n328 = case shown="참" w702 {
                      tunnel: w701 -> [_ w705]
                      frame False {
                      }
                      frame True {
                        n329 = local write "Rx-mon"(FALSE ("수신 실패(T) 1")) -> ()
                        n330 = local write "Rx-debug"(FALSE ("Rx-debug")) -> ()
                        n331 = local write "Rx-ROM"(TRUE ("Rx-ROM")) -> ()
                        n332 = stacked-sequence {
                          tunnel: w705 -> [w728 _ _]
                          frame #0 {
                            # "Check data input status"
                            n333 = call "SUB-BLE Rx data (Mon)-ROM.vi"("data in"=w728) -> ("data Out"=w713:u8[], "Index"=w714:u8)  [unwired: 3 in]
                            n334 = property on="ROM Data" class="Arr (엄격한)"("Index Values"=u32[] [] ("인덱스 값")) -> ()  [unwired: 2 in, 2 out]
                            n335 = local read "ROM Data"() -> (w727:T11)
                            n336 = Bundle By Name(cluster=T17 {"RxOK"=FALSE, "ROM Data"=[], "Index"=0} ("클러스터"), "RxOK"=TRUE ("Packet Detect"), "ROM Data"=w713, "Index"=w714) -> (w725:T17)
                            n337 = Replace Array Subset(array=w727, new element=w725, index=w714) -> (w711:T11)
                            n338 = local read "Rx ROM-log"() -> (w722:string)
                            n339 = Format Into String(format string="[Packet ID]%02d  " ("포맷 문자열"), w714) -> (resulting string=w716:string)  [unwired: 2 in, 1 out]
                            n340 = for {
                              tunnel: w711 -> [w730] mode=indexing
                              tunnel: [w729] -> w710 mode=indexing
                              n341 = Unbundle By Name(w730) -> ("RxOK"=w729:bool)
                            }
                            n342 = local write "ROM Data"(w711) -> ()
                            n343 = call <vilib>:"Space Constant.vi"() -> ("String"=w715:string)
                            n344 = Array To Spreadsheet String(delimiter (Tab)=w715, array=w713, 3:"%02X" ("포맷 문자열")) -> (spreadsheet string=w718:string)
                            n345 = Format Date/Time String(time format string (%c)="%H:%M:%S%3u>  " ("상태")) -> (date/time string=w720:string)  [unwired: 2 in]
                            n346 = Concatenate Strings(w722, w716, w720, w718) -> (w721:string)
                            n347 = Boolean Array To Number(Boolean array=w710) -> (number=w709:u32)
                            n348 = local write "Rx ROM-log"(w721) -> ()
                            n349 = Equal?(x=w709, y=u32 7) -> (x = y?=w708:bool)
                            n350 = local write "Full ROM data"(w708) -> ()
                          }
                          frame #1 {
                            n351 = control-ref of="ROM Data"() -> (w732:refnum<vi>)
                            n352 = control-ref of="ROM Table"() -> (w731:refnum<vi>)
                            n353 = call "SUB-ROM Data convert to table.vi"("ROM Table Ref"=w731, "ROM Data Ref"=w732) -> ()  [unwired: 2 in, 2 out]
                          }
                          frame #2 {
                            # "Setting Info Table update"
                            n354 = property on="ROM Table" class="Tbl (엄격한)"() -> ("Column Headers[]"=w742:string[], "Row Headers[]"=w741:string[], "Value"=w734:string[][])  [unwired: 2 in, 2 out]
                            n355 = Index Array(array=w734, index (col)=1 ("비활성화된 인덱스 (열)")) -> (element=w738:string[])  [unwired: 1 in]
                            n356 = for {
                              tunnel: w738 -> [w754] mode=indexing
                              shift-right: [w749] -> w736
                              shift-left: string[][] [] -> [w748]
                              n357 = Spreadsheet String To Array(delimiter (Tab)=" " ("구분 문자(탭)"), format string="%s" ("포맷 문자열"), spreadsheet string=w754, array type (2D Dbl)=string[] []) -> (array=w750:string[])
                              n358 = Build Array (concatenate)(w748, w750) -> (w749:string[][])
                            }
                            n359 = Index Array(array=w736, index (col)=0 ("비활성화된 인덱스 (열)")) -> (element=w735:string[])  [unwired: 1 in]
                            n360 = for {
                              tunnel: w735 -> [w747] mode=indexing
                              shift-right: [w744] -> w733
                              shift-left: w734 -> [w743]
                              i -> [w745]
                              n361 = Replace Array Subset(array=w743, new element=w747, index (row)=w745, index (col)=1 ("비활성화된 인덱스 (열)")) -> (w744:string[][])
                            }
                            n362 = property on="ROM Table 2" class="Tbl (엄격한)"("Column Headers[]"=w742, "Row Headers[]"=w741, "Value"=w733) -> ()  [unwired: 2 in, 2 out]
                          }
                        }
                      }
                    }
                  }
                }
                n363 = Quotient & Remainder(x=w653, y=w656) -> (x-y*floor(x/y)=w654:i32)  [unwired: 1 out]
                n364 = Divide(x=w656, y=2) -> (x/y=w657:dbl)
                n365 = Greater?(x=w654, y=w657) -> (0:w655:bool)
                n366 = local write "ACT-Comm"(w655) -> ()
              }
            }
          }
          frame #2 {
            # "Monitoring Data"
            n367 = local read "Rx-mon"() -> (w755:bool)
            n368 = case shown="참" w755 {
              frame False {
              }
              frame True {
                # "#Processing Received Data"
                n369 = local read "ms timer 3"() -> (w760:u32)
                n370 = local read "Update(ms)"() -> (w756:u16)
                n371 = Tick Count (ms)() -> (millisecond timer value=w759:u32)
                n372 = Subtract(x=w759, y=w760) -> (x-y=w757:u32)
                n373 = Greater Or Equal?(x=w757, y=w756) -> (x >= y?=w758:bool)
                n374 = case shown="참" w758 {
                  frame False {
                  }
                  frame True {
                    n375 = local read "BLE Packet (mon)"() -> (w765:u8[])
                    n376 = call "SUB-BLE Rx data (Mon)-CDC IMU.vi"("data in"=w765) -> ("IMU data"=w762:T10, "CDC data"=w763:T9, "Bat"=w761:u16, "*Board ID"=w764:string)  [unwired: 4 in]
                    n377 = stacked-sequence {
                      seq-local: [w768 _ _ _ _ _] -> [_ _ w815 _ w846 _]
                      tunnel: w764 -> [w767 _ _ _ _ _]
                      tunnel: w763 -> [_ w786 _ _ _ _]
                      tunnel: w762 -> [_ _ _ w830 _ _]
                      tunnel: w761 -> [_ _ _ _ _ w868]
                      frame #0 {
                        # "SN"
                        n378 = Tick Count (ms)() -> (millisecond timer value=w766:u32)
                        n379 = local write "ms timer 3"(w766) -> ()
                        n380 = local write "*Board ID1"(w767) -> ()
                        n381 = local read "Graph timer 1"() -> (w769:u32)
                        n382 = Tick Count (ms)() -> (millisecond timer value=w770:u32)
                        n383 = flat-sequence {
                          tunnel: w770 -> [w775]
                          tunnel: w769 -> [w772]
                          tunnel: [w771] -> w768
                          frame #0 {
                            n384 = Subtract(x=w775, y=w772) -> (x-y=w773:u32)
                            n385 = local write "Graph timer 1"(w775) -> ()
                            n386 = Multiply(x=w773, y=0.001 ("dt")) -> (x*y=w771:dbl)
                          }
                        }
                      }
                      frame #1 {
                        # "CDC Data"
                        n387 = local read "Offset Souce"() -> (w779:enum32{"Normal", "Raw"})
                        n388 = Unbundle By Name(w786) -> ("Left Wing-A, C1/C0"=w785:dbl, "Left Wing-B, C2/C0"=w784:dbl, "Left Wing-C, C3/C0"=w783:dbl, "Right Wing-A, C4/C0"=w782:dbl, "Right Wing-B, C5/C0"=w781:dbl, "Right Wing-C, C6/C0"=w780:dbl)
                        n389 = Equal?(x=w779, y=enum32{"Normal", "Raw"}."Normal" ("Offset Souce")) -> (x = y?=w777:bool)
                        n390 = case shown="참" w777 {
                          tunnel: [_ w801] -> w776
                          frame False {
                          }
                          frame True {
                            n391 = local read "CDC Offet"() -> (w801:T9)
                          }
                        }
                        n392 = Unbundle By Name(w776) -> ("Left Wing-A, C1/C0"=w800:dbl, "Left Wing-B, C2/C0"=w799:dbl, "Left Wing-C, C3/C0"=w798:dbl, "Right Wing-A, C4/C0"=w797:dbl, "Right Wing-B, C5/C0"=w796:dbl, "Right Wing-C, C6/C0"=w795:dbl)
                        n393 = Subtract(x=w785, y=w800) -> (x-y=w792:dbl)
                        n394 = Subtract(x=w784, y=w799) -> (x-y=w791:dbl)
                        n395 = Subtract(x=w783, y=w798) -> (x-y=w790:dbl)
                        n396 = Subtract(x=w782, y=w797) -> (x-y=w789:dbl)
                        n397 = Subtract(x=w781, y=w796) -> (x-y=w788:dbl)
                        n398 = Subtract(x=w780, y=w795) -> (x-y=w787:dbl)
                        n399 = local read "CDC data"() -> (w794:T9)
                        n400 = Bundle By Name(cluster=w794, "Left Wing-A, C1/C0"=w792, "Left Wing-B, C2/C0"=w791, "Left Wing-C, C3/C0"=w790, "Right Wing-A, C4/C0"=w789, "Right Wing-B, C5/C0"=w788, "Right Wing-C, C6/C0"=w787) -> (w793:T9)
                        n401 = local write "CDC data"(w793) -> ()
                      }
                      frame #2 {
                        # "* Plot"
                        n402 = local read "CDC data"() -> (w814:T9)
                        n403 = Unbundle By Name(w814) -> ("Left Wing-A, C1/C0"=w813:dbl, "Left Wing-B, C2/C0"=w806:dbl, "Left Wing-C, C3/C0"=w805:dbl, "Right Wing-A, C4/C0"=w804:dbl, "Right Wing-B, C5/C0"=w803:dbl, "Right Wing-C, C6/C0"=w802:dbl)
                        n404 = Build Array(w813) -> (w812:dbl[])
                        n405 = Get Date/Time In Seconds() -> (seconds since 1Jan1904=w818:timestamp)
                        n406 = Build Array(w806) -> (w811:dbl[])
                        n407 = Build Array(w805) -> (w810:dbl[])
                        n408 = Build Array(w803) -> (w808:dbl[])
                        n409 = Build Array(w804) -> (w809:dbl[])
                        n410 = Build Array(w802) -> (w807:dbl[])
                        n411 = Bundle By Name("t0"=w818, "Y"=w812, "dt"=w815) -> (w823:waveform(dbl))  [unwired: 1 in]
                        n412 = Bundle By Name("t0"=w818, "Y"=w811, "dt"=w815) -> (w822:waveform(dbl))  [unwired: 1 in]
                        n413 = Bundle By Name("t0"=w818, "Y"=w810, "dt"=w815) -> (w821:waveform(dbl))  [unwired: 1 in]
                        n414 = Bundle By Name("t0"=w818, "Y"=w809, "dt"=w815) -> (w819:waveform(dbl))  [unwired: 1 in]
                        n415 = Bundle By Name("t0"=w818, "Y"=w808, "dt"=w815) -> (w817:waveform(dbl))  [unwired: 1 in]
                        n416 = Bundle By Name("t0"=w818, "Y"=w807, "dt"=w815) -> (w816:waveform(dbl))  [unwired: 1 in]
                        n417 = Build Array(w823, w822, w821, w819, w817, w816) -> (→"CDC(PCAP02) Graph":waveform(dbl)[])
                      }
                      frame #3 {
                        # "IMU Data"
                        n418 = local read "IMU Offet"() -> (w845:T10)
                        n419 = Unbundle By Name(w830) -> ("Gyroscope X"=w829:dbl, "Gyroscope Y"=w828:dbl, "Gyroscope Z"=w827:dbl, "Accelerometer X"=w826:dbl, "Accelerometer Y"=w825:dbl, "Accelerometer Z"=w824:dbl)
                        n420 = Unbundle By Name(w845) -> ("Gyroscope X"=w842:dbl, "Gyroscope Y"=w841:dbl, "Gyroscope Z"=w840:dbl, "Accelerometer X"=w839:dbl, "Accelerometer Y"=w838:dbl, "Accelerometer Z"=w837:dbl)
                        n421 = Subtract(x=w829, y=w842) -> (x-y=w836:dbl)
                        n422 = Subtract(x=w828, y=w841) -> (x-y=w835:dbl)
                        n423 = Subtract(x=w827, y=w840) -> (x-y=w834:dbl)
                        n424 = Subtract(x=w826, y=w839) -> (x-y=w833:dbl)
                        n425 = Subtract(x=w825, y=w838) -> (x-y=w832:dbl)
                        n426 = Subtract(x=w824, y=w837) -> (x-y=w831:dbl)
                        n427 = local read "IMU data"() -> (w844:T10)
                        n428 = Bundle By Name(cluster=w844, "Gyroscope X"=w836, "Gyroscope Y"=w835, "Gyroscope Z"=w834, "Accelerometer X"=w833, "Accelerometer Y"=w832, "Accelerometer Z"=w831) -> (w843:T10)
                        n429 = local write "IMU data"(w843) -> ()
                      }
                      frame #4 {
                        # "* Plot"
                        n430 = local read "IMU data"() -> (w859:T10)
                        n431 = Unbundle By Name(w859) -> ("Gyroscope X"=w858:dbl, "Gyroscope Y"=w851:dbl, "Gyroscope Z"=w850:dbl, "Accelerometer X"=w849:dbl, "Accelerometer Y"=w848:dbl, "Accelerometer Z"=w847:dbl)
                        n432 = Build Array(w858) -> (w857:dbl[])
                        n433 = Get Date/Time In Seconds() -> (seconds since 1Jan1904=w862:timestamp)
                        n434 = Build Array(w851) -> (w856:dbl[])
                        n435 = Build Array(w850) -> (w855:dbl[])
                        n436 = Build Array(w848) -> (w853:dbl[])
                        n437 = Build Array(w849) -> (w854:dbl[])
                        n438 = Build Array(w847) -> (w852:dbl[])
                        n439 = Bundle By Name("t0"=w862, "Y"=w857, "dt"=w846) -> (w866:waveform(dbl))  [unwired: 1 in]
                        n440 = Bundle By Name("t0"=w862, "Y"=w856, "dt"=w846) -> (w865:waveform(dbl))  [unwired: 1 in]
                        n441 = Bundle By Name("t0"=w862, "Y"=w855, "dt"=w846) -> (w864:waveform(dbl))  [unwired: 1 in]
                        n442 = Bundle By Name("t0"=w862, "Y"=w854, "dt"=w846) -> (w863:waveform(dbl))  [unwired: 1 in]
                        n443 = Bundle By Name("t0"=w862, "Y"=w853, "dt"=w846) -> (w861:waveform(dbl))  [unwired: 1 in]
                        n444 = Bundle By Name("t0"=w862, "Y"=w852, "dt"=w846) -> (w860:waveform(dbl))  [unwired: 1 in]
                        n445 = Build Array(w866, w865, w864, w863, w861, w860) -> (→"IMU Graph":waveform(dbl)[])
                      }
                      frame #5 {
                        # "BAT raw data"
                        n446 = local write "Bat(raw)"(w868) -> ()
                      }
                    }
                  }
                }
              }
            }
          }
          frame #3 {
            # "Debugging data"
            n447 = local read "Rx-debug"() -> (w869:bool)
            n448 = case shown="참" w869 {
              frame False {
              }
              frame True {
                # "#Processing Received Data"
                n449 = local read "ms timer 3"() -> (w874:u32)
                n450 = local read "Update(ms)"() -> (w870:u16)
                n451 = Tick Count (ms)() -> (millisecond timer value=w873:u32)
                n452 = Subtract(x=w873, y=w874) -> (x-y=w871:u32)
                n453 = Greater Or Equal?(x=w871, y=w870) -> (x >= y?=w872:bool)
                n454 = case shown="참" w872 {
                  frame False {
                  }
                  frame True {
                    n455 = local read "BLE Packet (mon)"() -> (w877:u8[])
                    n456 = call "SUB-BLE Rx data (Debug)-CDC.vi"("data in"=w877) -> ("CDC debug"=w875:T9, "CDC mon"=w876:T9)  [unwired: 6 in]
                    n457 = stacked-sequence {
                      seq-local: [w879 _ _ _ _] -> [_ _ _ w954 w973]
                      seq-local: [_ _ _ w940 _] -> [_ _ _ _ w962]
                      seq-local: [_ _ _ w939 _] -> [_ _ _ _ w982]
                      seq-local: [_ _ w913 _ _] -> [_ _ _ _ w961]
                      tunnel: w876 -> [_ w891 _ _ _]
                      tunnel: w875 -> [_ _ w914 _ _]
                      frame #0 {
                        n458 = Tick Count (ms)() -> (millisecond timer value=w878:u32)
                        n459 = local write "ms timer 3"(w878) -> ()
                        n460 = local read "Graph timer 1"() -> (w880:u32)
                        n461 = Tick Count (ms)() -> (millisecond timer value=w881:u32)
                        n462 = flat-sequence {
                          tunnel: w881 -> [w886]
                          tunnel: w880 -> [w883]
                          tunnel: [w882] -> w879
                          frame #0 {
                            n463 = Subtract(x=w886, y=w883) -> (x-y=w884:u32)
                            n464 = local write "Graph timer 1"(w886) -> ()
                            n465 = Multiply(x=w884, y=0.001 ("dt")) -> (x*y=w882:dbl)
                          }
                        }
                      }
                      frame #1 {
                        # "CDC Data"
                        n466 = local read "Offset Souce"() -> (w890:enum32{"Normal", "Raw"})
                        n467 = Unbundle By Name(w891) -> ("Left Wing-A, C1/C0"=w897:dbl, "Left Wing-B, C2/C0"=w896:dbl, "Left Wing-C, C3/C0"=w895:dbl, "Right Wing-A, C4/C0"=w894:dbl, "Right Wing-B, C5/C0"=w893:dbl, "Right Wing-C, C6/C0"=w892:dbl)
                        n468 = Equal?(x=w890, y=enum32{"Normal", "Raw"}."Normal" ("Offset Souce")) -> (x = y?=w888:bool)
                        n469 = case shown="참" w888 {
                          tunnel: [_ w912] -> w887
                          frame False {
                          }
                          frame True {
                            n470 = local read "CDC Offet"() -> (w912:T9)
                          }
                        }
                        n471 = Unbundle By Name(w887) -> ("Left Wing-A, C1/C0"=w911:dbl, "Left Wing-B, C2/C0"=w910:dbl, "Left Wing-C, C3/C0"=w909:dbl, "Right Wing-A, C4/C0"=w908:dbl, "Right Wing-B, C5/C0"=w907:dbl, "Right Wing-C, C6/C0"=w906:dbl)
                        n472 = Subtract(x=w897, y=w911) -> (x-y=w903:dbl)
                        n473 = Subtract(x=w896, y=w910) -> (x-y=w902:dbl)
                        n474 = Subtract(x=w895, y=w909) -> (x-y=w901:dbl)
                        n475 = Subtract(x=w894, y=w908) -> (x-y=w900:dbl)
                        n476 = Subtract(x=w893, y=w907) -> (x-y=w899:dbl)
                        n477 = Subtract(x=w892, y=w906) -> (x-y=w898:dbl)
                        n478 = local read "CDC data"() -> (w905:T9)
                        n479 = Bundle By Name(cluster=w905, "Left Wing-A, C1/C0"=w903, "Left Wing-B, C2/C0"=w902, "Left Wing-C, C3/C0"=w901, "Right Wing-A, C4/C0"=w900, "Right Wing-B, C5/C0"=w899, "Right Wing-C, C6/C0"=w898) -> (w904:T9)
                        n480 = local write "CDC data"(w904) -> ()
                      }
                      frame #2 {
                        n481 = local read "Offset Souce"() -> (w918:enum32{"Normal", "Raw"})
                        n482 = Unbundle By Name(w914) -> ("Left Wing-A, C1/C0"=w924:dbl, "Left Wing-B, C2/C0"=w923:dbl, "Left Wing-C, C3/C0"=w922:dbl, "Right Wing-A, C4/C0"=w921:dbl, "Right Wing-B, C5/C0"=w920:dbl, "Right Wing-C, C6/C0"=w919:dbl)
                        n483 = Equal?(x=w918, y=enum32{"Normal", "Raw"}."Raw" ("Offset Souce")) -> (x = y?=w916:bool)
                        n484 = case shown="참" w916 {
                          tunnel: [_ w938] -> w915
                          frame False {
                          }
                          frame True {
                            n485 = local read "CDC Offet"() -> (w938:T9)
                          }
                        }
                        n486 = Unbundle By Name(w915) -> ("Left Wing-A, C1/C0"=w937:dbl, "Left Wing-B, C2/C0"=w936:dbl, "Left Wing-C, C3/C0"=w935:dbl, "Right Wing-A, C4/C0"=w934:dbl, "Right Wing-B, C5/C0"=w933:dbl, "Right Wing-C, C6/C0"=w932:dbl)
                        n487 = Subtract(x=w924, y=w937) -> (x-y=w930:dbl)
                        n488 = Subtract(x=w923, y=w936) -> (x-y=w929:dbl)
                        n489 = Subtract(x=w922, y=w935) -> (x-y=w928:dbl)
                        n490 = Subtract(x=w921, y=w934) -> (x-y=w927:dbl)
                        n491 = Subtract(x=w920, y=w933) -> (x-y=w926:dbl)
                        n492 = Subtract(x=w919, y=w932) -> (x-y=w925:dbl)
                        n493 = local read "CDC data"() -> (w931:T9)
                        n494 = Bundle By Name(cluster=w931, "Left Wing-A, C1/C0"=w930, "Left Wing-B, C2/C0"=w929, "Left Wing-C, C3/C0"=w928, "Right Wing-A, C4/C0"=w927, "Right Wing-B, C5/C0"=w926, "Right Wing-C, C6/C0"=w925) -> (w913:T9)
                      }
                      frame #3 {
                        # "* Plot"
                        n495 = local read "CDC data"() -> (w953:T9)
                        n496 = Unbundle By Name(w953) -> ("Left Wing-A, C1/C0"=w952:dbl, "Left Wing-B, C2/C0"=w945:dbl, "Left Wing-C, C3/C0"=w944:dbl, "Right Wing-A, C4/C0"=w943:dbl, "Right Wing-B, C5/C0"=w942:dbl, "Right Wing-C, C6/C0"=w941:dbl)
                        n497 = Build Array(w952) -> (w951:dbl[])
                        n498 = Get Date/Time In Seconds() -> (seconds since 1Jan1904=w940:timestamp)
                        n499 = Build Array(w945) -> (w950:dbl[])
                        n500 = Build Array(w944) -> (w949:dbl[])
                        n501 = Build Array(w942) -> (w947:dbl[])
                        n502 = Build Array(w943) -> (w948:dbl[])
                        n503 = Build Array(w941) -> (w946:dbl[])
                        n504 = Bundle By Name("t0"=w940, "Y"=w951, "dt"=w954) -> (w960:waveform(dbl))  [unwired: 1 in]
                        n505 = Bundle By Name("t0"=w940, "Y"=w950, "dt"=w954) -> (w959:waveform(dbl))  [unwired: 1 in]
                        n506 = Bundle By Name("t0"=w940, "Y"=w949, "dt"=w954) -> (w958:waveform(dbl))  [unwired: 1 in]
                        n507 = Bundle By Name("t0"=w940, "Y"=w948, "dt"=w954) -> (w957:waveform(dbl))  [unwired: 1 in]
                        n508 = Bundle By Name("t0"=w940, "Y"=w947, "dt"=w954) -> (w956:waveform(dbl))  [unwired: 1 in]
                        n509 = Bundle By Name("t0"=w940, "Y"=w946, "dt"=w954) -> (w955:waveform(dbl))  [unwired: 1 in]
                        n510 = Build Array(w960, w959, w958, w957, w956, w955) -> (w939:waveform(dbl)[])
                      }
                      frame #4 {
                        n511 = Unbundle By Name(w961) -> ("Left Wing-A, C1/C0"=w980:dbl, "Left Wing-B, C2/C0"=w979:dbl, "Left Wing-C, C3/C0"=w966:dbl, "Right Wing-A, C4/C0"=w965:dbl, "Right Wing-B, C5/C0"=w964:dbl, "Right Wing-C, C6/C0"=w963:dbl)
                        n512 = Build Array(w980) -> (w981:dbl[])
                        n513 = Build Array(w965) -> (w971:dbl[])
                        n514 = Build Array(w979) -> (w978:dbl[])
                        n515 = Build Array(w966) -> (w977:dbl[])
                        n516 = Build Array(w964) -> (w974:dbl[])
                        n517 = Build Array(w963) -> (w975:dbl[])
                        n518 = Bundle By Name("t0"=w962, "Y"=w981, "dt"=w973) -> (w983:waveform(dbl))  [unwired: 1 in]
                        n519 = Bundle By Name("t0"=w962, "Y"=w978, "dt"=w973) -> (w976:waveform(dbl))  [unwired: 1 in]
                        n520 = Bundle By Name("t0"=w962, "Y"=w977, "dt"=w973) -> (w972:waveform(dbl))  [unwired: 1 in]
                        n521 = Bundle By Name("t0"=w962, "Y"=w971, "dt"=w973) -> (w970:waveform(dbl))  [unwired: 1 in]
                        n522 = Bundle By Name("t0"=w962, "Y"=w974, "dt"=w973) -> (w969:waveform(dbl))  [unwired: 1 in]
                        n523 = Bundle By Name("t0"=w962, "Y"=w975, "dt"=w973) -> (w968:waveform(dbl))  [unwired: 1 in]
                        n524 = Build Array (concatenate)(w982, w983, w976, w972, w970, w969, w968) -> (w967:waveform(dbl)[])
                        n525 = local write "CDC(PCAP02) Graph"(w967) -> ()
                      }
                    }
                  }
                }
              }
            }
          }
          frame #4 {
            # "Force Test"
            n526 = local read "Comm con status 1"() -> (w985:bool)
            n527 = local read "Test Start"() -> (w984:bool)
            n528 = case shown="참" w985 {
              tunnel: w984 -> [_ w989]
              frame False {
                n529 = local write "FTS Testing"(FALSE ("FTS 시험 진행")) -> ()
                n530 = local write "Test Start"(FALSE ("Test Start")) -> ()
                n531 = local write "FTS comm."(FALSE ("FTS 수신 정상")) -> ()
              }
              frame True {
                n532 = case shown="참" w989 {
                  frame False {
                  }
                  frame True {
                    n533 = stacked-sequence {
                      frame #0 {
                        # "Init"
                        n534 = disable-structure shown="비활성화" {
                          frame Disabled {
                            # "170125"
                            # "Test Mode"
                            # "Calibration Mode"
                            # "가로"
                            # "세로"
                            n535 = local read "Cal/Test select"() -> (w1004:bool)
                            n536 = Select(t=7, s=w1004, f=5) -> (s? t:f=w1001:i32)
                            n537 = for {
                              N: 9 -> [_]
                              tunnel: [w1008] -> w1005 mode=indexing
                              tunnel: w1001 -> [w1007]
                              # "가로"
                              n538 = for {
                                N: w1007 -> [_]
                                tunnel: ["-"] -> w1008 mode=indexing
                              }
                            }
                            n539 = local write "Test Data table"(w1005) -> ()
                          }
                          frame Enabled {
                          }
                        }
                        n540 = Wait Until Next ms Multiple(millisecond multiple=u32 100 ("ms 배수")) -> ()  [unwired: 1 out]
                        n541 = local write "Mark10 Gauge (lb)"(0.0 ("Mark10 Gauge")) -> ()
                        n542 = local write "FTS Testing"(TRUE ("FTS 시험 진행")) -> ()
                        n543 = local write "FTS comm."(FALSE ("FTS 수신 정상")) -> ()
                        n544 = local write "status string"("Force Test Mode..." ("status string")) -> ()
                        n545 = local write "FTS OP status"(T7 "Test_Start" ("FTS OP status")) -> ()
                        n546 = Format Date/Time String(time format string (%c)="%Y/%m/%d %H:%M:%S> Force Test Start\n" ("상태")) -> (date/time string=w994:string)  [unwired: 2 in]
                        n547 = local write "Test Status"(w994) -> ()
                        n548 = call "Sub-CDC_Data_Cluster_Buffer.vi"("Mode"=enum16{"Init", "Add", "Add Load", "Out"}."Init") -> ()  [unwired: 10 in, 1 out]
                        n549 = local write "FTS table index"(0 ("FTS table index")) -> ()
                        n550 = local write "Load Graph"(cluster{dbl[], dbl[]} {[], []} ("Load Graph")) -> ()
                      }
                      frame #1 {
                        # "the number of Load Test Profile"
                        # "col"
                        # "Calibration Profile Load"
                        # "170125"
                        # "#FTS_PROFILE"
                        n551 = disable-structure shown="활성화" {
                          disable-tunnel: [w1040 w1047] -> w1024
                          frame Enabled {
                            n552 = call <vilib>:"Application Directory.vi"() -> ("Application Directory"=w1039:path)
                            n553 = Build Path(base path=w1039, name or relative path="Template" ("이름 또는 상대 경로")) -> (appended path=w1042:path)
                            n554 = Build Path(base path=w1042, name or relative path="FTS Profile-OS.csv" ("이름 또는 상대 경로")) -> (appended path=w1040:path)
                          }
                          frame Disabled {
                            # "For Validation Test"
                            n555 = call <vilib>:"Application Directory.vi"() -> ("Application Directory"=w1045:path)
                            n556 = Build Path(base path=w1045, name or relative path="Template" ("이름 또는 상대 경로")) -> (appended path=w1044:path)
                            n557 = call "파일 대화 상자"("start path"=w1044) -> ("selected path"=w1047:path)  [unwired: 11 in, 3 out]
                          }
                        }
                        n558 = call "Load_Array_Data_to_File_txt.vi"("file path (use dialog)"=w1024) -> ("array"=w1017:string[][])  [unwired: 8 in, 2 out]
                        n559 = Index Array(array=w1017, index (col)=0 ("비활성화된 인덱스 (열)")) -> (element=w1022:string[])  [unwired: 1 in]
                        n560 = local write "Test profile"(w1017) -> ()
                        n561 = for {
                          tunnel: w1022 -> [w1049] mode=indexing
                          tunnel: [w1049] -> w1014 mode=indexing if=w1048
                          n562 = String Subset(string=w1049, length (rest)=4 ("길이(나머지)")) -> (substring=w1052:string)  [unwired: 1 in]
                          n563 = To Upper Case(1:w1052) -> (0:w1051:string)
                          n564 = Equal?(x=w1051, y="LOAD") -> (x = y?=w1048:bool)
                        }
                        n565 = Index Array(array=w1017, index (col)=6 ("비활성화된 인덱스 (열)")) -> (element=w1016:string[])  [unwired: 1 in]
                        n566 = for {
                          tunnel: w1016 -> [w1035] mode=indexing
                          tunnel: [w1032] -> w1015 mode=indexing if=w1032
                          n567 = Decimal String To Number(string=w1035) -> (number=w1034:i32)  [unwired: 2 in, 1 out]
                          n568 = Equal?(x=1, y=w1034) -> (x = y?=w1032:bool)
                        }
                        n569 = Array Size(array=w1014) -> (size(s)=w1013:i32)
                        n570 = Array Size(array=w1015) -> (size(s)=w1012:i32)
                        n571 = Subtract(x=w1013, y=w1012) -> (x-y=w1011:i32)
                        n572 = disable-structure shown="활성화" {
                          disable-tunnel: w1014 -> [w1028 w1031]
                          disable-tunnel: w1011 -> [w1027 _]
                          disable-tunnel: [w1025 w1031] -> w1010
                          frame Disabled {
                            n573 = Insert Into Array(array=w1028, index=w1027, new element="Offset") -> (w1026:string[])
                            n574 = Build Array (concatenate)("Offset", w1026) -> (w1025:string[])
                          }
                          frame Enabled {
                          }
                        }
                        n575 = Array Size(array=w1010) -> (size(s)=w1019:i32)
                        n576 = for {
                          N: 9 -> [_]
                          tunnel: [w1037] -> w1020 mode=indexing
                          tunnel: w1019 -> [w1036]
                          # "row"
                          n577 = for {
                            N: w1036 -> [_]
                            tunnel: ["-"] -> w1037 mode=indexing
                          }
                        }
                        n578 = local write "Test Data table"(w1020) -> ()
                        n579 = property on="Test Data table" class="Tbl (엄격한)"("Column Headers[]"=w1010) -> ()  [unwired: 2 in, 2 out]
                      }
                      frame #2 {
                        n580 = local read "Port-FTS"() -> (w1059:refnum<visa-resource-name>)
                        n581 = control-ref of="Test Status"() -> (w1055:refnum<vi>)
                        n582 = call "_Serial_Mark10-Connection_Check.vi"("Serial Port"=w1059) -> ("Normal reception"=w1058:bool, "VISA resource name out"=w1057:refnum<visa-resource-name>)  [unwired: 3 in]
                        n583 = call "SUB-Status string update.vi"("String In"="Check Serial port of Mark-10\n" ("Force Test Status"), "Add Date"=TRUE ("날짜추가"), "reference"=w1055) -> ()  [unwired: 2 in, 1 out]
                        n584 = case shown="거짓" w1058 {
                          tunnel: w1057 -> [_ _]
                          frame False {
                            # "Communication fail"
                            n585 = local write "FTS OP status"(T7 "Test_End" ("FTS OP status")) -> ()
                            n586 = One Button Dialog(message="Cannot find MARK10.\nCheck comm port." ("메시지")) -> ()  [unwired: 1 in, 1 out]
                          }
                          frame True {
                            n587 = local read "Port-FTS"() -> (w1062:refnum<visa-resource-name>)
                            n588 = call "_Serial_Mark10-Setup(Zero).vi"("Serial Port"=w1062) -> ()  [unwired: 4 in, 1 out]
                          }
                        }
                        n589 = local write "FTS comm."(w1058) -> ()
                      }
                      frame #3 {
                        n590 = while {
                          stop <- w1065 stop-if-true
                          n591 = local read "Test profile"() -> (w1064:string[][])
                          n592 = case shown="\"Proceed-Press\"" "FTS OP status" {
                            tunnel: [w1070 _ _ _ TRUE _] -> w1065
                            tunnel: w1064 -> [_ _ w1075 w1260 _ _]
                            frame "Test_Start" {
                              n593 = control-ref of="Test Status"() -> (w1068:refnum<vi>)
                              n594 = local write "FTS OP status"(T7 "Check_Before_Test" ("FTS OP status")) -> ()
                              n595 = call "SUB-Status string update.vi"("String In"="Force Test Start!\n" ("Force Test Status"), "Add Date"=TRUE ("날짜추가"), "reference"=w1068) -> ()  [unwired: 2 in, 1 out]
                              n596 = local read "stop"() -> (w1070:bool)
                            }
                            frame "Check_Before_Test" {
                              n597 = local read "Port-FTS"() -> (w1073:refnum<visa-resource-name>)
                              n598 = call "_Serial_Mark10-Data reception(Gauge).vi"("Serial Port"=w1073) -> ("data(lb)"=w1072:dbl, "Normal reception"=w1074:bool)  [unwired: 2 in, 1 out]
                              n599 = local write "Mark10 Gauge (lb)"(w1072) -> ()
                              n600 = local write "FTS comm."(w1074) -> ()
                              n601 = local write "FTS OP status"(T7 "Proceed-Press" ("FTS OP status")) -> ()
                            }
                            frame "Proceed-Press" {
                              n602 = stacked-sequence {
                                tunnel: w1075 -> [_ w1080 _]
                                frame #0 {
                                n603 = control-ref of="Test Status"() -> (w1078:refnum<vi>)
                                n604 = local write "CDC Offet"(T9 {"Left Wing-A, C1/C0"=0.0, "Left Wing-B, C2/C0"=0.0, "Left Wing-C, C3/C0"=0.0, "Right Wing-A, C4/C0"=0.0, "Right Wing-B, C5/C0"=0.0, "Right Wing-C, C6/C0"=0.0} ("CDC Offet")) -> ()
                                n605 = call "SUB-Status string update.vi"("String In"="Start Force test by Profile" ("Force Test Status"), "Add Date"=TRUE ("날짜추가"), "reference"=w1078) -> ()  [unwired: 2 in, 1 out]
                                }
                                frame #1 {
                                n606 = for {
                                tunnel: w1080 -> [w1083] mode=indexing
                                i -> [w1081]
                                stop <- w1082 continue-if-true
                                n607 = stacked-sequence {
                                seq-local: [_ w1098 _ _ _ _ _ _ _] -> [_ _ _ _ w1120 w1161 _ _ _]
                                seq-local: [w1084 _ _ _ _ _ _ _ _] -> [_ _ _ _ w1119 w1147 _ _ _]
                                seq-local: [_ _ w1105 _ _ _ _ _ _] -> [_ _ _ _ _ _ _ w1216 _]
                                tunnel: w1081 -> [w1091 _ _ _ _ _ _ w1215 _]
                                tunnel: w1083 -> [w1085 w1103 w1108 _ _ _ w1184 _ w1244]
                                tunnel: [_ w1100 _ _ _ _ _ _ _] -> w1082
                                frame #0 {
                                # "Data Aquisition?"
                                # "String for test state"
                                n608 = Index Array(array=w1085, index=4 ("인덱스")) -> (element=w1087:string)
                                n609 = Fract/Exp String To Number(string=w1087) -> (number=w1086:dbl)  [unwired: 3 in, 1 out]
                                n610 = Not Equal To 0?(x=w1086) -> (x != 0?=w1084:bool)
                                n611 = Index Array(array=w1085, index=0 ("인덱스")) -> (element=w1089:string)
                                n612 = Increment(x=w1091) -> (x+1=w1092:i32)
                                n613 = control-ref of="Test Status"() -> (w1095:refnum<vi>)
                                n614 = Format Into String(format string="Force Testing-Profile(%d)...%s" ("Force Test Status"), w1092, w1089) -> (resulting string=w1094:string)  [unwired: 2 in, 1 out]
                                n615 = call "SUB-Status string update.vi"("String In"=w1094, "Add Date"=TRUE ("날짜추가"), "reference"=w1095) -> ()  [unwired: 2 in, 1 out]
                                }
                                frame #1 {
                                # "Press"
                                n616 = Index Array(array=w1103, index=1 ("인덱스")) -> (element=w1101:string)
                                n617 = local read "Port-FTS"() -> (w1104:refnum<visa-resource-name>)
                                n618 = Fract/Exp String To Number(string=w1101) -> (number=w1098:dbl)  [unwired: 3 in, 1 out]
                                n619 = call "_Serial_Mark10-Control (Press Config).vi"("FTS Operation state"=T24 "Start pressure control", "Press Setting(lb)"=w1098, "Serial Port"=w1104) -> ("Gauge Pressure(lb)"=w1099:dbl, "Communication is normal"=w1100:bool)  [unwired: 1 out]
                                n620 = local write "Mark10 Gauge (lb)"(w1099) -> ()
                                n621 = local write "FTS comm."(w1100) -> ()
                                }
                                frame #2 {
                                # "Delay"
                                n622 = Tick Count (ms)() -> (millisecond timer value=w1107:u32)
                                n623 = Index Array(array=w1108, index=2 ("인덱스")) -> (element=w1109:string)
                                n624 = Fract/Exp String To Number(string=w1109) -> (number=w1106:dbl)  [unwired: 3 in, 1 out]
                                n625 = while {
                                tunnel: w1107 -> [w1117]
                                tunnel: w1106 -> [w1115]
                                tunnel: [w1111] -> w1105
                                stop <- w1114 stop-if-true
                                n626 = Tick Count (ms)() -> (millisecond timer value=w1118:u32)
                                n627 = Subtract(x=w1118, y=w1117) -> (x-y=w1116:u32)
                                n628 = local read "Port-FTS"() -> (w1112:refnum<visa-resource-name>)
                                n629 = Greater Or Equal?(x=w1116, y=w1115) -> (x >= y?=w1114:bool)
                                n630 = call "_Serial_Mark10-Data reception(Gauge).vi"("Serial Port"=w1112) -> ("data(lb)"=w1111:dbl)  [unwired: 2 in, 2 out]
                                n631 = local write "Mark10 Gauge (lb)"(w1111) -> ()
                                n632 = Wait Until Next ms Multiple(millisecond multiple=u32 50 ("ms 배수")) -> ()  [unwired: 1 out]
                                }
                                }
                                frame #3 {
                                # "Clear BLE Buffer"
                                n633 = call "SUB-BLE Rx data Clear.vi"() -> ()  [unwired: 6 in]
                                }
                                frame #4 {
                                n634 = case shown="참" w1119 {
                                tunnel: w1120 -> [_ w1133]
                                frame False {
                                }
                                frame True {
                                # "Rescale to the number of data"
                                # "Data Aquisition Delay & Read Gauge"
                                n635 = Equal To 0?(x=w1133) -> (x = 0?=w1129:bool)
                                n636 = Select(t=0.5, s=w1129, f=1.0) -> (s? t:f=w1127:dbl)
                                n637 = Select(t=50, s=w1129, f=100) -> (s? t:f=w1125:i32)
                                n638 = Get Date/Time In Seconds() -> (seconds since 1Jan1904=w1132:timestamp)
                                n639 = while {
                                tunnel: w1132 -> [w1138]
                                tunnel: w1127 -> [w1135]
                                tunnel: [w1134] -> w1124 mode=indexing
                                stop <- w1137 stop-if-true
                                n640 = Get Date/Time In Seconds() -> (seconds since 1Jan1904=w1139:timestamp)
                                n641 = Subtract(x=w1139, y=w1138) -> (x-y=w1136:dbl)
                                n642 = Greater Or Equal?(x=w1136, y=w1135) -> (x >= y?=w1137:bool)
                                n643 = local read "Port-FTS"() -> (w1140:refnum<visa-resource-name>)
                                n644 = call "_Serial_Mark10-Data reception(Gauge).vi"("Serial Port"=w1140) -> ("data(lb)"=w1134:dbl)  [unwired: 2 in, 2 out]
                                }
                                n645 = To Double Precision Float(number=w1125) -> (double precision float=w1123:dbl)
                                n646 = call "Sub_X_Scale_Change.vi"("Target Scale"=w1123, "input"=w1124) -> ("output"=w1121:dbl[])  [unwired: 9 in]
                                n647 = call "Sub-CDC_Data_Cluster_Buffer.vi"("Mode"=enum16{"Init", "Add", "Add Load", "Out"}."Add Load", "Input Load"=w1121) -> ()  [unwired: 9 in, 1 out]
                                }
                                }
                                }
                                frame #5 {
                                # "CDC Data acquisition"
                                n648 = Equal To 0?(x=w1161) -> (x = 0?=w1160:bool)
                                n649 = Select(t=50, s=w1160, f=100) -> (s? t:f=w1157:i32)
                                n650 = for {
                                N: w1157 -> [_]
                                tunnel: [w1174] -> w1150 mode=indexing
                                tunnel: [w1173] -> w1151 mode=indexing
                                tunnel: [w1172] -> w1152 mode=indexing
                                tunnel: [w1171] -> w1153 mode=indexing
                                tunnel: [w1170] -> w1154 mode=indexing
                                tunnel: [w1169] -> w1155 mode=indexing
                                tunnel: [w1166] -> w1148 mode=indexing
                                n651 = local read "CDC data"() -> (w1167:T9)
                                n652 = call "SUB-BLE Rx data (Mon)-Wait.vi"("Timeout(ms)"=u16 100) -> ("RxReady"=w1175:bool)  [unwired: 4 in]
                                n653 = case shown="참" w1175 {
                                tunnel: [w1179 w1182] -> w1168
                                tunnel: w1167 -> [w1179 _]
                                tunnel: [u16 0 ("Bat") w1180] -> w1166
                                frame False {
                                }
                                frame True {
                                n654 = call "SUB-BLE Rx data (Mon)-Classify.vi"() -> ("data out"=w1181:u8[])  [unwired: 5 in, 4 out]
                                n655 = call "SUB-BLE Rx data (Mon)-CDC IMU.vi"("data in"=w1181) -> ("CDC data"=w1182:T9, "Bat"=w1180:u16)  [unwired: 4 in, 2 out]
                                }
                                }
                                n656 = Unbundle By Name(w1168) -> ("Left Wing-A, C1/C0"=w1174:dbl, "Left Wing-B, C2/C0"=w1173:dbl, "Left Wing-C, C3/C0"=w1172:dbl, "Right Wing-A, C4/C0"=w1171:dbl, "Right Wing-B, C5/C0"=w1170:dbl, "Right Wing-C, C6/C0"=w1169:dbl)
                                n657 = Wait Until Next ms Multiple(millisecond multiple=u32 5 ("ms 배수")) -> ()  [unwired: 1 out]
                                }
                                n658 = call-poly <vilib>:"Mean.vi"("X"=w1150) -> ("mean"=w1146:dbl)  [unwired: 1 out]
                                n659 = call-poly <vilib>:"Mean.vi"("X"=w1151) -> ("mean"=w1145:dbl)  [unwired: 1 out]
                                n660 = call-poly <vilib>:"Mean.vi"("X"=w1152) -> ("mean"=w1144:dbl)  [unwired: 1 out]
                                n661 = call-poly <vilib>:"Mean.vi"("X"=w1153) -> ("mean"=w1143:dbl)  [unwired: 1 out]
                                n662 = call-poly <vilib>:"Mean.vi"("X"=w1154) -> ("mean"=w1142:dbl)  [unwired: 1 out]
                                n663 = call-poly <vilib>:"Mean.vi"("X"=w1155) -> ("mean"=w1141:dbl)  [unwired: 1 out]
                                n664 = Bundle By Name(cluster=T9 {"Left Wing-A, C1/C0"=0.0, "Left Wing-B, C2/C0"=0.0, "Left Wing-C, C3/C0"=0.0, "Right Wing-A, C4/C0"=0.0, "Right Wing-B, C5/C0"=0.0, "Right Wing-C, C6/C0"=0.0} ("CDC data"), "Left Wing-A, C1/C0"=w1146, "Left Wing-B, C2/C0"=w1145, "Left Wing-C, C3/C0"=w1144, "Right Wing-A, C4/C0"=w1143, "Right Wing-B, C5/C0"=w1142, "Right Wing-C, C6/C0"=w1141) -> (w1162:T9)
                                n665 = Bundle By Name(cluster=T27 {"LWA"=[], "LWB"=[], "LWC"=[], "RWA"=[], "RWB"=[], "RWC"=[], "Bat"=[]} ("Output CL"), "LWA"=w1150, "LWB"=w1151, "LWC"=w1152, "RWA"=w1153, "RWB"=w1154, "RWC"=w1155, "Bat"=w1148) -> (w1156:T27)
                                n666 = local write "CDC data"(w1162) -> ()
                                n667 = case shown="참" w1147 {
                                tunnel: w1156 -> [_ w1165]
                                frame False {
                                }
                                frame True {
                                n668 = call "Sub-CDC_Data_Cluster_Buffer.vi"("Mode"=enum16{"Init", "Add", "Add Load", "Out"}."Add", "Input CL"=w1165) -> ()  [unwired: 9 in, 1 out]
                                }
                                }
                                }
                                frame #6 {
                                n669 = Index Array(array=w1184, index=4 ("인덱스")) -> (element=w1186:string)
                                n670 = Fract/Exp String To Number(string=w1186) -> (number=w1185:dbl)  [unwired: 3 in, 1 out]
                                n671 = Not Equal To 0?(x=w1185) -> (x != 0?=w1183:bool)
                                n672 = case shown="참" w1183 {
                                frame False {
                                }
                                frame True {
                                w1202 = i16 1 ("정밀도(6)")
                                n673 = local read "CDC data"() -> (w1213:T9)
                                n674 = Unbundle By Name(w1213) -> ("Left Wing-A, C1/C0"=w1197:dbl, "Left Wing-B, C2/C0"=w1198:dbl, "Left Wing-C, C3/C0"=w1199:dbl, "Right Wing-A, C4/C0"=w1195:dbl, "Right Wing-B, C5/C0"=w1194:dbl, "Right Wing-C, C6/C0"=w1193:dbl)
                                n675 = local read "Mark10 Gauge (lb)"() -> (w1192:dbl)
                                n676 = local read "FTS table index"() -> (w1188:i32)
                                n677 = Compound Arithmetic op=ADD(w1199, w1198, w1197) -> (w1200:dbl)
                                n678 = Compound Arithmetic op=ADD(w1195, w1194, w1193) -> (w1196:dbl)
                                n679 = Number To Fractional String(number=w1197, precision (6)=w1202) -> (F-format string=w1212:string)  [unwired: 2 in]
                                n680 = Number To Fractional String(number=w1198, precision (6)=w1202) -> (F-format string=w1211:string)  [unwired: 2 in]
                                n681 = Number To Fractional String(number=w1192, precision (6)=i16 2 ("정밀도(6)")) -> (F-format string=w1190:string)  [unwired: 2 in]
                                n682 = Number To Fractional String(number=w1199, precision (6)=w1202) -> (F-format string=w1210:string)  [unwired: 2 in]
                                n683 = Number To Fractional String(number=w1200, precision (6)=w1202) -> (F-format string=w1203:string)  [unwired: 2 in]
                                n684 = Number To Fractional String(number=w1195, precision (6)=w1202) -> (F-format string=w1209:string)  [unwired: 2 in]
                                n685 = Number To Fractional String(number=w1194, precision (6)=w1202) -> (F-format string=w1208:string)  [unwired: 2 in]
                                n686 = Number To Fractional String(number=w1193, precision (6)=w1202) -> (F-format string=w1207:string)  [unwired: 2 in]
                                n687 = Number To Fractional String(number=w1196, precision (6)=w1202) -> (F-format string=w1201:string)  [unwired: 2 in]
                                n688 = local read "Test Data table"() -> (w1204:string[][])
                                n689 = Increment(x=w1188) -> (x+1=w1189:i32)
                                n690 = Build Array(w1190, w1212, w1211, w1210, w1203, w1209, w1208, w1207, w1201) -> (w1206:string[])
                                n691 = local write "FTS table index"(w1189) -> ()
                                n692 = Replace Array Subset(array=w1204, new element=w1206, index (col)=w1188) -> (w1205:string[][])  [unwired: 1 in]
                                n693 = local write "Test Data table"(w1205) -> ()
                                }
                                }
                                }
                                frame #7 {
                                # "Load Graph"
                                n694 = local read "Test Data table"() -> (w1217:string[][])
                                n695 = disable-structure shown="활성화" {
                                disable-tunnel: [w1225 w1235] -> w1214
                                disable-tunnel: w1217 -> [w1224 _]
                                disable-tunnel: w1216 -> [_ w1238]
                                disable-tunnel: w1215 -> [_ w1242]
                                frame Disabled {
                                n696 = local read "FTS table index"() -> (w1220:i32)
                                n697 = Decrement(x=w1220) -> (x-1=w1219:i32)
                                n698 = Array Subset(array=w1224, index (col)=1 ("비활성화된 인덱스 (열)"), length (col)=w1219) -> (w1221:string[][])  [unwired: 2 in]
                                n699 = Fract/Exp String To Number(string=w1221) -> (number=w1223:dbl[][])  [unwired: 3 in, 1 out]
                                n700 = for {
                                N: 8 -> [_]
                                tunnel: [w1233] -> w1225 mode=indexing
                                tunnel: w1223 -> [w1232]
                                i -> [w1230]
                                # "Y"
                                # "X"
                                n701 = Add(x=1, y=w1230) -> (x+y=w1228:i32)
                                n702 = Index Array(array=w1232, index (row)=0 ("비활성화된 인덱스 (열)")) -> (element=w1227:dbl[])  [unwired: 1 in]
                                n703 = Index Array(array=w1232, index (row)=w1228) -> (element=w1226:dbl[])  [unwired: 1 in]
                                n704 = Bundle(w1227, w1226) -> (w1233:cluster{dbl[], dbl[]})  [unwired: 1 in]
                                }
                                }
                                frame Enabled {
                                n705 = To Double Precision Float(number=w1242) -> (double precision float=w1240:dbl)
                                n706 = property on="Load Graph" class="XYGraph (엄격한)"() -> ("Value"=w1234:cluster{dbl[], dbl[]})  [unwired: 2 in, 2 out]
                                n707 = Unbundle(w1234) -> (w1241:dbl[], w1239:dbl[])
                                n708 = Build Array (concatenate)(w1239, w1238) -> (w1236:dbl[])
                                n709 = Build Array (concatenate)(w1241, w1240) -> (w1237:dbl[])
                                n710 = Bundle(w1237, w1236) -> (w1235:cluster{dbl[], dbl[]})  [unwired: 1 in]
                                }
                                }
                                "Load Graph" <- w1214
                                }
                                frame #8 {
                                n711 = Index Array(array=w1244, index=5 ("인덱스")) -> (element=w1246:string)
                                n712 = Fract/Exp String To Number(string=w1246) -> (number=w1245:dbl)  [unwired: 3 in, 1 out]
                                n713 = Not Equal To 0?(x=w1245) -> (x != 0?=w1243:bool)
                                n714 = case shown="참" w1243 {
                                frame False {
                                }
                                frame True {
                                n715 = stacked-sequence {
                                seq-local: [w1249 _] -> [_ w1255]
                                frame #0 {
                                n716 = local read "Port-FTS"() -> (w1249:refnum<visa-resource-name>)
                                n717 = control-ref of="Test Status"() -> (w1251:refnum<vi>)
                                n718 = call "_Serial_Mark10-Control (Press Config).vi"("FTS Operation state"=T24 "Move Header Up", "Serial Port"=w1249) -> ("Gauge Pressure(lb)"=w1253:dbl, "Communication is normal"=w1254:bool)  [unwired: 1 in, 1 out]
                                n719 = call "SUB-Status string update.vi"("String In"="Head Up" ("Force Test Status"), "Add Date"=TRUE ("날짜추가"), "reference"=w1251) -> ()  [unwired: 2 in, 1 out]
                                n720 = local write "Mark10 Gauge (lb)"(w1253) -> ()
                                n721 = local write "FTS comm."(w1254) -> ()
                                }
                                frame #1 {
                                n722 = call "_Serial_Mark10-Setup(Zero).vi"("Serial Port"=w1255) -> ()  [unwired: 4 in, 1 out]
                                }
                                }
                                }
                                }
                                }
                                }
                                }
                                }
                                frame #2 {
                                n723 = local write "FTS OP status"(T7 "Gen_Report" ("FTS OP status")) -> ()
                                n724 = control-ref of="Test Status"() -> (w1258:refnum<vi>)
                                n725 = call "SUB-Status string update.vi"("String In"="Done Force test by Profile\n" ("Force Test Status"), "Add Date"=TRUE ("날짜추가"), "reference"=w1258) -> ()  [unwired: 2 in, 1 out]
                                }
                              }
                            }
                            frame "Check_After_Test" {
                              n726 = disable-structure shown="비활성화" {
                                disable-tunnel: w1260 -> [w1262 _]
                                frame Disabled {
                                # "LAT"
                                # "CAL"
                                # "Test End & \nSave Measurement data"
                                n727 = stacked-sequence {
                                seq-local: [_ w1288 _] -> [_ _ w1298]
                                seq-local: [w1276 _ _] -> [_ w1287 _]
                                seq-local: [w1270 _ _] -> [_ _ w1297]
                                seq-local: [w1267 _ _] -> [_ _ w1296]
                                seq-local: [w1266 _ _] -> [_ _ w1295]
                                tunnel: w1262 -> [w1269 _ _]
                                frame #0 {
                                w1284 = T31 1 items=["사용자 홈"=0, "사용자 데스크탑"=1, "사용자 문서"=2, "사용자 어플리케이션 데이터"=3, "사용자 환경"=4, "사용자 임시"=5, "퍼블릭 문서"=6, "퍼블릭 어플리케이션 데이터"=7, "퍼블릭 환경"=8, "퍼블릭 캐시"=13, "시스템 코어 라이브러리"=9, "시스템 설치된 라이브러리"=10, "어플리케이션 파일"=11, "부팅 볼륨 루트"=12] ("system directory type")
                                n728 = local read "Test Data table"() -> (w1268:string[][])
                                n729 = call "SUB-FTS_Result_divide.vi"("Table Value"=w1268, "Test profile"=w1269) -> ("Load Test data"=w1266:string[][], "Cal data"=w1267:string[][])  [unwired: 8 in]
                                n730 = call "SUB-module-Current VI Path.vi"() -> ("현재 VI 경로"=w1273:path)
                                n731 = call <vilib>:"Get System Directory.vi"("system directory type"=w1284) -> ("system directory"=w1283:path)  [unwired: 10 in]
                                n732 = Path To String(path=w1273) -> (string=w1272:string)
                                n733 = Path To String(path=w1283) -> (string=w1282:string)
                                n734 = Concatenate Strings(w1272, "\\Template" ("이름 또는 상대 경로"), "\\GEN4 FTS Test Report rev2.xlsx" ("이름 또는 상대 경로")) -> (w1271:string)
                                n735 = String To Path(string=w1271) -> (path=w1270:path)
                                n736 = Concatenate Strings(w1282, "\\GEN4-GUI Test data" ("상태")) -> (w1276:string)
                                n737 = String To Path(string=w1276) -> (path=w1280:path)
                                n738 = call <vilib>:"Check if File or Folder Exists.vi"("path"=w1280) -> ("error out"=w1277:errorcluster, "file or folder exists?"=w1279:bool, "dup path"=w1278:path)  [unwired: 8 in]
                                n739 = case shown="거짓" w1279 {
                                tunnel: w1278 -> [w1286 _]
                                tunnel: w1277 -> [w1285 _]
                                frame False {
                                n740 = Create Folder(path (use dialog)=w1286, error in=w1285) -> ()  [unwired: 1 in, 3 out]
                                }
                                frame True {
                                }
                                }
                                }
                                frame #1 {
                                # "* Filename(rev)-date (trst name)"
                                # "파일 저장 경로"
                                n741 = local read "Test name"() -> (w1293:string)
                                n742 = Format Date/Time String(time format string (%c)="%Y%m%d %H%M%S" ("상태")) -> (date/time string=w1292:string)  [unwired: 2 in]
                                n743 = Format Into String(format string="\\\\GEN4 FTS (PP3A)-%s (%s).xlsx" ("상태"), w1292, w1293) -> (resulting string=w1289:string)  [unwired: 2 in, 1 out]
                                n744 = Concatenate Strings(w1287, w1289) -> (w1294:string)
                                n745 = String To Path(string=w1294) -> (path=w1288:path)
                                }
                                frame #2 {
                                n746 = call <vilib>:"New Report.vi"("window state (normal)"=T20."normal", "report type"=T19."Excel", "template (empty)"=w1297) -> ("report out"=w1301:refnum<class "NI_report.lvclass">, "error out"=w1302:errorcluster)  [unwired: 11 in]
                                n747 = stacked-sequence {
                                tunnel: w1301 -> [w1306 w1331 w1333 w1359]
                                tunnel: w1302 -> [w1305 w1330 w1334 w1358]
                                tunnel: [w1306 _ _ _] -> w1304
                                tunnel: [w1305 _ _ _] -> w1303
                                tunnel: w1296 -> [_ _ _ w1357]
                                tunnel: w1295 -> [_ _ _ w1356]
                                frame #0 {
                                }
                                frame #1 {
                                w1309 = 11 ("column")
                                w1316 = 2 ("row")
                                w1323 = 1 items=["top", "center", "bottom"] ("vertical alignment (top)")
                                # "Date"
                                # "박스의 좌측 상단 좌표"
                                n748 = Add(x=w1309, y=3) -> (x+y=w1307:i32)
                                n749 = Increment(x=w1316) -> (x+1=w1311:i32)
                                n750 = Bundle By Name(cluster=cluster{"row":i32, "column":i32} {"row"=3, "column"=10} ("start (-1, -1)"), "row"=w1311, "column"=w1307) -> (w1310:cluster{"row":i32, "column":i32})
                                n751 = Bundle By Name(cluster=cluster{"row":i32, "column":i32} {"row"=3, "column"=10} ("start (-1, -1)"), "row"=w1311, "column"=w1309) -> (w1317:cluster{"row":i32, "column":i32})
                                n752 = Format Date/Time String(time format string (%c)="%Y/%m/%d-%H:%M:%S" ("상태")) -> (date/time string=w1329:string)  [unwired: 2 in]
                                n753 = call <vilib>:"Excel Easy Text.vi"("report in"=w1331, "font"=T21 {"font name"="", "font size"=11.0, "bold"=1, "italic"=0, "underline"=0, "strike through"=0, "font color"=16777216}, "text"=w1329, "start (-1, -1)"=w1317, "end (-1, -1)"=w1310, "error in (no error)"=w1330) -> ("report out"=w1327:refnum<class "NI_report.lvclass">, "next cell bottom-left"=w1325:cluster{"row":i32, "column":i32}, "next cell top-right"=w1324:cluster{"row":i32, "column":i32}, "error out"=w1326:errorcluster)  [unwired: 5 in, 1 out]
                                n754 = Bundle By Name(cluster=cluster{"row":i32, "column":i32} {"row"=3, "column"=10} ("start (-1, -1)"), "row"=w1316, "column"=w1309) -> (w1315:cluster{"row":i32, "column":i32})
                                n755 = call <vilib>:"Excel Set Cell Alignment.vi"("report in"=w1327, "vertical alignment (top)"=w1323, "horizontal alignment (left)"=w1323, "start (-1, -1)"=w1325, "end (-1, -1)"=w1324, "error in (no error)"=w1326) -> ("report out"=w1322:refnum<class "NI_report.lvclass">, "error out"=w1321:errorcluster)  [unwired: 8 in]
                                n756 = call <vilib>:"Excel Set Cell Color and Border.vi"("report in"=w1322, "outside border"=T22 {"on/off"=TRUE, "weight"=2, "color"=0}, "background color (w)"=u32 16777215, "start (-1, -1)"=w1315, "end (-1, -1)"=w1310, "error in (no error)"=w1321) -> ()  [unwired: 8 in, 2 out]
                                }
                                frame #2 {
                                w1337 = 1 ("column")
                                w1344 = 4 ("row")
                                w1351 = 1 items=["top", "center", "bottom"] ("vertical alignment (top)")
                                # "Device No."
                                # "박스의 좌측 상단 좌표"
                                n757 = local read "Test name"() -> (w1332:string)
                                n758 = Increment(x=w1337) -> (x+1=w1336:i32)
                                n759 = Increment(x=w1344) -> (x+1=w1339:i32)
                                n760 = Increment(x=w1336) -> (x+1=w1338:i32)
                                n761 = Bundle By Name(cluster=cluster{"row":i32, "column":i32} {"row"=3, "column"=10} ("start (-1, -1)"), "row"=w1339, "column"=w1338) -> (w1335:cluster{"row":i32, "column":i32})
                                n762 = Bundle By Name(cluster=cluster{"row":i32, "column":i32} {"row"=3, "column"=10} ("start (-1, -1)"), "row"=w1339, "column"=w1337) -> (w1345:cluster{"row":i32, "column":i32})
                                n763 = call <vilib>:"Excel Easy Text.vi"("report in"=w1333, "font"=T21 {"font name"="", "font size"=11.0, "bold"=1, "italic"=0, "underline"=0, "strike through"=0, "font color"=16777216}, "text"=w1332, "start (-1, -1)"=w1345, "end (-1, -1)"=w1335, "error in (no error)"=w1334) -> ("report out"=w1355:refnum<class "NI_report.lvclass">, "next cell bottom-left"=w1353:cluster{"row":i32, "column":i32}, "next cell top-right"=w1352:cluster{"row":i32, "column":i32}, "error out"=w1354:errorcluster)  [unwired: 5 in, 1 out]
                                n764 = Bundle By Name(cluster=cluster{"row":i32, "column":i32} {"row"=3, "column"=10} ("start (-1, -1)"), "row"=w1344, "column"=w1337) -> (w1343:cluster{"row":i32, "column":i32})
                                n765 = call <vilib>:"Excel Set Cell Alignment.vi"("report in"=w1355, "vertical alignment (top)"=w1351, "horizontal alignment (left)"=w1351, "start (-1, -1)"=w1353, "end (-1, -1)"=w1352, "error in (no error)"=w1354) -> ("report out"=w1350:refnum<class "NI_report.lvclass">, "error out"=w1349:errorcluster)  [unwired: 8 in]
                                n766 = call <vilib>:"Excel Set Cell Color and Border.vi"("report in"=w1350, "outside border"=T22 {"on/off"=TRUE, "weight"=2, "color"=0}, "background color (w)"=u32 16777215, "start (-1, -1)"=w1343, "end (-1, -1)"=w1335, "error in (no error)"=w1349) -> ()  [unwired: 8 in, 2 out]
                                }
                                frame #3 {
                                n767 = stacked-sequence {
                                seq-local: [w1361 _] -> [_ w1400]
                                seq-local: [w1360 _] -> [_ w1401]
                                tunnel: w1359 -> [w1364 _]
                                tunnel: w1358 -> [w1363 _]
                                tunnel: w1357 -> [w1362 _]
                                tunnel: w1356 -> [_ w1402]
                                frame #0 {
                                # "Cal-mode"
                                n768 = stacked-sequence {
                                tunnel: w1364 -> [w1376 w1397]
                                tunnel: w1363 -> [w1375 w1396]
                                tunnel: w1362 -> [w1365 w1379]
                                tunnel: [_ w1378] -> w1361
                                tunnel: [_ w1377] -> w1360
                                frame #0 {
                                # "Load(lb)"
                                n769 = Index Array(array=w1365, index (row)=0 ("인덱스 (행)")) -> (element=w1372:string[])  [unwired: 1 in]
                                n770 = Replace Array Subset(array=w1372, new element="Offset" ("새 원소/부분배열"), index=0 ("인덱스")) -> (w1369:string[])
                                n771 = Build Array(w1369) -> (w1368:string[][])
                                n772 = Transpose 2D Array(2D array=w1368) -> (transposed array=w1367:string[][])
                                n773 = call-poly <vilib>:"Excel Easy Table.vi"("report in"=w1376, "font"=T21 {"font name"="", "font size"=11.0, "bold"=0, "italic"=0, "underline"=0, "strike through"=0, "font color"=16777216}, "start (0, 0)"=cluster{"row":i32, "column":i32} {"row"=15, "column"=1}, "text data"=w1367, "error in (no error)"=w1375) -> ()  [unwired: 6 in, 5 out]
                                }
                                frame #1 {
                                # "Load(lb)"
                                n774 = Index Array(array=w1379, index (row) #1=1 ("인덱스 (행)"), index (row) #2=2 ("인덱스 (행)"), index (row) #3=3 ("인덱스 (행)")) -> (element #1=w1390:string[], element #2=w1389:string[], element #3=w1388:string[])  [unwired: 3 in]
                                n775 = Index Array(array=w1379, index (row) #1=5 ("인덱스 (행)"), index (row) #2=6 ("인덱스 (행)"), index (row) #3=7 ("인덱스 (행)")) -> (element #1=w1387:string[], element #2=w1386:string[], element #3=w1385:string[])  [unwired: 3 in]
                                n776 = Build Array(w1387, w1386, w1385) -> (w1383:string[][])
                                n777 = Build Array(w1390, w1389, w1388) -> (w1384:string[][])
                                n778 = Build Array (concatenate)(w1384, w1383) -> (w1382:string[][])
                                n779 = Transpose 2D Array(2D array=w1382) -> (transposed array=w1381:string[][])
                                n780 = call-poly <vilib>:"Excel Easy Table.vi"("report in"=w1397, "font"=T21 {"font name"="", "font size"=11.0, "bold"=0, "italic"=0, "underline"=0, "strike through"=0, "font color"=16777216}, "start (0, 0)"=cluster{"row":i32, "column":i32} {"row"=15, "column"=3}, "text data"=w1381, "error in (no error)"=w1396) -> ("report out"=w1378:refnum<class "NI_report.lvclass">, "error out"=w1377:errorcluster)  [unwired: 6 in, 3 out]
                                }
                                }
                                }
                                frame #1 {
                                # "Test-mode"
                                n781 = stacked-sequence {
                                tunnel: w1400 -> [w1414 w1433]
                                tunnel: w1401 -> [w1413 w1432]
                                tunnel: w1402 -> [w1403 w1415]
                                frame #0 {
                                # "Load(lb)"
                                n782 = Index Array(array=w1403, index (row)=0 ("인덱스 (행)")) -> (element=w1410:string[])  [unwired: 1 in]
                                n783 = Replace Array Subset(array=w1410, new element="Offset" ("새 원소/부분배열"), index=0 ("인덱스")) -> (w1407:string[])
                                n784 = Build Array(w1407) -> (w1406:string[][])
                                n785 = Transpose 2D Array(2D array=w1406) -> (transposed array=w1405:string[][])
                                n786 = call-poly <vilib>:"Excel Easy Table.vi"("report in"=w1414, "font"=T21 {"font name"="", "font size"=11.0, "bold"=0, "italic"=0, "underline"=0, "strike through"=0, "font color"=16777216}, "start (0, 0)"=cluster{"row":i32, "column":i32} {"row"=25, "column"=1}, "text data"=w1405, "error in (no error)"=w1413) -> ()  [unwired: 6 in, 5 out]
                                }
                                frame #1 {
                                # "Load(lb)"
                                n787 = Index Array(array=w1415, index (row) #1=1 ("인덱스 (행)"), index (row) #2=2 ("인덱스 (행)"), index (row) #3=3 ("인덱스 (행)")) -> (element #1=w1426:string[], element #2=w1425:string[], element #3=w1424:string[])  [unwired: 3 in]
                                n788 = Index Array(array=w1415, index (row) #1=5 ("인덱스 (행)"), index (row) #2=6 ("인덱스 (행)"), index (row) #3=7 ("인덱스 (행)")) -> (element #1=w1423:string[], element #2=w1422:string[], element #3=w1421:string[])  [unwired: 3 in]
                                n789 = Build Array(w1423, w1422, w1421) -> (w1419:string[][])
                                n790 = Build Array(w1426, w1425, w1424) -> (w1420:string[][])
                                n791 = Build Array (concatenate)(w1420, w1419) -> (w1418:string[][])
                                n792 = Transpose 2D Array(2D array=w1418) -> (transposed array=w1417:string[][])
                                n793 = call-poly <vilib>:"Excel Easy Table.vi"("report in"=w1433, "font"=T21 {"font name"="", "font size"=11.0, "bold"=0, "italic"=0, "underline"=0, "strike through"=0, "font color"=16777216}, "start (0, 0)"=cluster{"row":i32, "column":i32} {"row"=25, "column"=3}, "text data"=w1417, "error in (no error)"=w1432) -> ()  [unwired: 6 in, 5 out]
                                }
                                }
                                }
                                }
                                }
                                }
                                n794 = call-dynamic "Save Report to File.vi"("report in"=w1304, "report file path"=w1298, "error in (no error)"=w1303) -> ()  [unwired: 11 in, 2 out]
                                }
                                }
                                n795 = control-ref of="Test Status"() -> (w1264:refnum<vi>)
                                n796 = call "SUB-Status string update.vi"("String In"="Result Data Process\n" ("Force Test Status"), "Add Date"=TRUE ("날짜추가"), "reference"=w1264) -> ()  [unwired: 2 in, 1 out]
                                n797 = local write "FTS OP status"(T7 "Test_End" ("FTS OP status")) -> ()
                                }
                                frame Enabled {
                                }
                              }
                            }
                            frame "Test_End", Default {
                              # "Test_End"
                              n798 = control-ref of="Test Status"() -> (w1439:refnum<vi>)
                              n799 = local write "Mark10 Gauge (lb)"(0.0 ("Mark10 Gauge")) -> ()
                              n800 = local write "Clear graph 1"(TRUE ("그래프 지우기")) -> ()
                              n801 = call "SUB-Status string update.vi"("String In"="Test complete." ("Force Test Status"), "Add Date"=TRUE ("날짜추가"), "reference"=w1439) -> ()  [unwired: 2 in, 1 out]
                              n802 = call <vilib>:"Beep.vi"() -> ()  [unwired: 12 in]
                              n803 = call "SUB-BLE Rx data Clear.vi"() -> ()  [unwired: 6 in]
                            }
                            frame "Gen_Report" {
                              n804 = local read "Test name"() -> (w1448:string)
                              n805 = Format Date/Time String(time format string (%c)="%Y%m%d %H%M%S" ("상태")) -> (date/time string=w1447:string)  [unwired: 2 in]
                              n806 = control-ref of="Test Status"() -> (w1450:refnum<vi>)
                              n807 = Format Into String(format string="GEN4 FTS-%s (%s).xlsm" ("상태"), w1447, w1448) -> (resulting string=w1445:string)  [unwired: 2 in, 1 out]
                              n808 = call "SUB-Status string update.vi"("String In"="Result Data Process\n" ("Force Test Status"), "Add Date"=TRUE ("날짜추가"), "reference"=w1450) -> ()  [unwired: 2 in, 1 out]
                              n809 = call "Sub_Report_Generation.vi"("File Name"=w1445) -> ("error out"=w1444:errorcluster)  [unwired: 10 in]
                              n810 = case shown="에러" w1444 {
                                frame No Error {
                                }
                                frame Error {
                                n811 = One Button Dialog(message="Report Generation Error" ("메시지")) -> ()  [unwired: 1 in, 1 out]
                                }
                              }
                              n812 = local write "FTS OP status"(T7 "Test_End" ("FTS OP status")) -> ()
                            }
                          }
                        }
                      }
                      frame #4 {
                        n813 = local write "FTS comm."(FALSE ("FTS 수신 정상")) -> ()
                        n814 = local write "Test Start"(FALSE ("Test Start")) -> ()
                        n815 = local write "FTS Testing"(FALSE ("FTS 시험 진행")) -> ()
                      }
                    }
                  }
                }
              }
            }
          }
          frame #5 {
            # "Battery Calibration"
            n816 = local read "Comm con status 1"() -> (w1456:bool)
            n817 = case shown="거짓" w1456 {
              frame False {
              }
              frame True {
                n818 = stacked-sequence {
                  frame #0 {
                    # "ADC Linearity Start"
                    n819 = case shown="거짓" "ADC Linearity Start" {
                      frame False {
                      }
                      frame True {
                        w1458 = dbl[] []
                        n820 = while {
                          shift-right: [w1465] -> _
                          shift-left: 2.1 ("Voltage(V)") -> [w1466]
                          shift-right: [w1464] -> _
                          shift-left: w1458 -> [w1463]
                          shift-right: [w1462] -> _
                          shift-left: w1458 -> [w1461]
                          stop <- w1469 stop-if-true
                          n821 = case shown="\"Measurement\"" "Linerity State" {
                            tunnel: [w1470 _ errorcluster {"status"=TRUE, "code"=0, "source"=""} ("error out")] -> w1467
                            tunnel: w1466 -> [w1471 w1481 w1520]
                            tunnel: [w1471 w1491 w1520] -> w1465
                            tunnel: [w1474 w1487 _] -> w1464
                            tunnel: w1463 -> [_ w1490 _]
                            tunnel: [w1474 w1486 _] -> w1462
                            tunnel: w1461 -> [_ w1488 _]
                            frame "Initial", Default {
                              w1474 = dbl[] []
                              n822 = control-ref of="Linearity monitoring graph"() -> (w1480:refnum<vi>)
                              n823 = call "EX382280_Interface.vi"("mode"=382280_mode."Open", "error in (no error)"=errorcluster {"status"=FALSE, "code"=0, "source"=""}, "VISA resource name"="Power Supply Port") -> ("error out"=w1470:errorcluster)  [unwired: 7 in, 1 out]
                              n824 = property class="XYGraph (엄격한)"(reference=w1480, "Value"=cluster{dbl[], dbl[]} {[], []} ("값")) -> ()  [unwired: 1 in, 2 out]
                              n825 = Unbundle By Name(w1470) -> ("status"=→"Port Error":bool)
                              n826 = control-ref of="Linerity State"() -> (w1477:refnum<vi>)
                              n827 = property class="Enum (엄격한)"(reference=w1477, "Value"=Linerity_State."Measurement" ("Linerity State")) -> ()  [unwired: 1 in, 2 out]
                            }
                            frame "Measurement" {
                              n828 = Greater Or Equal?(x=w1481, y=3.2) -> (x >= y?=w1482:bool)
                              n829 = call "EX382280_Interface.vi"("mode"=382280_mode."V SET", "Voltage(V)"=w1481) -> ("error out"=w1484:errorcluster)  [unwired: 8 in, 1 out]
                              n830 = case shown="에러 없음" w1484 {
                                tunnel: [w1495 0.0] -> w1489
                                tunnel: w1482 -> [w1494 _]
                                frame No Error {
                                n831 = stacked-sequence {
                                tunnel: [_ _ _ w1498 _] -> w1495
                                tunnel: w1494 -> [_ _ _ _ w1509]
                                frame #0 {
                                # "Wait for 1sec to Voltage Stable"
                                n832 = Wait (ms)(milliseconds to wait=u32 3500 ("대기 시간(ms)")) -> ()  [unwired: 1 out]
                                }
                                frame #1 {
                                # "BLE Rx Buffer Clear"
                                n833 = call "SUB-BLE Rx data Clear.vi"() -> ()  [unwired: 6 in]
                                }
                                frame #2 {
                                # "500ms data received (50 Packets at 10ms interval time)"
                                n834 = Wait (ms)(milliseconds to wait=u32 500 ("대기 시간(ms)")) -> ()  [unwired: 1 out]
                                }
                                frame #3 {
                                # "Rx data & Average"
                                n835 = for {
                                N: 50 -> [_]
                                tunnel: [w1503] -> w1501 mode=indexing
                                n836 = call "SUB-BLE Rx data (Mon)-Wait.vi"("Timeout(ms)"=u16 100) -> ("RxReady"=w1505:bool)  [unwired: 4 in]
                                n837 = case shown="참" w1505 {
                                tunnel: [u16 0 ("Bat") w1507] -> w1503
                                frame False {
                                }
                                frame True {
                                n838 = call "SUB-BLE Rx data (Mon)-Classify.vi"() -> ("data out"=w1508:u8[])  [unwired: 5 in, 4 out]
                                n839 = call "SUB-BLE Rx data (Mon)-CDC IMU.vi"("data in"=w1508) -> ("Bat"=w1507:u16)  [unwired: 4 in, 3 out]
                                }
                                }
                                }
                                n840 = To Double Precision Float(number=w1501) -> (double precision float=w1500:dbl[])
                                n841 = call-poly <vilib>:"Mean.vi"("X"=w1500) -> ("mean"=w1499:dbl)  [unwired: 1 out]
                                n842 = Round Toward -Infinity(1:w1499) -> (0:w1498:dbl)
                                }
                                frame #4 {
                                n843 = case shown="참" w1509 {
                                tunnel: [Linerity_State."End" ("Linerity State") Linerity_State."Measurement" ("Linerity State")] -> w1510
                                frame True {
                                }
                                frame False {
                                }
                                }
                                n844 = control-ref of="Linerity State"() -> (w1511:refnum<vi>)
                                n845 = property class="Enum (엄격한)"(reference=w1511, "Value"=w1510) -> ()  [unwired: 1 in, 2 out]
                                }
                                }
                                }
                                frame Error {
                                n846 = control-ref of="Linerity State"() -> (w1515:refnum<vi>)
                                n847 = property class="Enum (엄격한)"(reference=w1515, "Value"=Linerity_State."End" ("Linerity State")) -> ()  [unwired: 1 in, 2 out]
                                }
                              }
                              n848 = Add(x=w1481, y=0.1 ("x")) -> (x+y=w1491:dbl)
                              n849 = Build Array (concatenate)(w1490, w1481) -> (w1487:dbl[])
                              n850 = Build Array (concatenate)(w1488, w1489) -> (w1486:dbl[])
                              n851 = Bundle(w1487, w1486) -> (→"Linearity monitoring graph":cluster{dbl[], dbl[]})  [unwired: 1 in]
                            }
                            frame "End" {
                              n852 = call "EX382280_Interface.vi"("mode"=382280_mode."V SET", "Voltage(V)"=3.0) -> ("error out"=w1518:errorcluster)  [unwired: 8 in, 1 out]
                              n853 = One Button Dialog(message="Done!!" ("메시지")) -> ()  [unwired: 1 in, 1 out]
                              n854 = control-ref of="Linerity State"() -> (w1524:refnum<vi>)
                              n855 = property class="Enum (엄격한)"(reference=w1524, "Value"=Linerity_State."Initial" ("Linerity State")) -> ()  [unwired: 1 in, 2 out]
                              n856 = call "Delay_ms.vi"("error in (no error)"=w1518) -> ("error out"=w1517:errorcluster)  [unwired: 10 in]
                              n857 = call "EX382280_Interface.vi"("mode"=382280_mode."Close", "error in (no error)"=w1517) -> ()  [unwired: 8 in, 2 out]
                            }
                          }
                          n858 = Or(x=w1467, y="ADC Linearity Stop") -> (x .or. y?=w1469:bool)
                        }
                      }
                    }
                  }
                }
              }
            }
          }
          frame #6 {
            # "Read at Manual Test"
            n859 = call "SUB-BLE Rx data (Set)-Classify.vi"() -> ("data out"=w1527:u8[], "Rx-data"=w1528:bool)  [unwired: 4 in]
            n860 = case shown="참" w1528 {
              tunnel: w1527 -> [_ w1531]
              frame False {
              }
              frame True {
                n861 = flat-sequence {
                  tunnel: w1531 -> [w1533]
                  tunnel: [w1533] -> w1529
                  tunnel: [w1535] -> w1530
                  tunnel: w1529 -> [w1535]
                  tunnel: w1530 -> [w1537]
                  frame #0 {
                    n862 = local write "Data_mon(h)"("" ("Data_mon")) -> ()
                  }
                  frame #1 {
                    n863 = Wait (ms)(milliseconds to wait=u32 20 ("대기 시간(ms)")) -> ()  [unwired: 1 out]
                  }
                  frame #2 {
                    n864 = Byte Array To String(unsigned byte array=w1537) -> (string=→"Data_mon(h)":string)
                    n865 = local read "Data Log"() -> (w1536:string)
                    n866 = call <vilib>:"Space Constant.vi"() -> ("String"=w1542:string)
                    n867 = Format Date/Time String(time format string (%c)="%H:%M:%S%3u>  " ("상태")) -> (date/time string=w1541:string)  [unwired: 2 in]
                    n868 = Array To Spreadsheet String(delimiter (Tab)=w1542, array=w1537, 3:"%02X" ("포맷 문자열")) -> (spreadsheet string=w1539:string)
                    n869 = Concatenate Strings(w1541, w1539, w1536) -> (w1538:string)
                    n870 = local write "Data Log"(w1538) -> ()
                  }
                }
              }
            }
          }
          frame #7 {
            n871 = local read "Comm con status 1"() -> (w1545:bool)
            n872 = case shown="거짓" w1545 {
              frame False {
              }
              frame True {
              }
            }
          }
          frame #8 {
            # "Reset"
            n873 = local read "Comm con status 1"() -> (w1551:bool)
            n874 = local read "Clear graph 1"() -> (w1550:bool)
            n875 = Not(x=w1551) -> (.not. x?=w1548:bool)
            n876 = case shown="참" w1548 {
              frame False {
              }
              frame True {
                n877 = local write "status string"("Ready (available after the communication connection)" ("status string")) -> ()
              }
            }
            n878 = case shown="참" w1550 {
              frame False {
              }
              frame True {
                n879 = local write "Clear graph 1"(FALSE ("그래프 지우기")) -> ()
                n880 = call "SUB-BLE Rx data Clear.vi"() -> ()  [unwired: 6 in]
                n881 = property on="CDC(PCAP02) Graph" class="WFChart (엄격한)"("History Data"=waveform(dbl)[][] [] ("히스토리 데이터")) -> ()  [unwired: 2 in, 2 out]
              }
            }
            n882 = local read "Export graph 1"() -> (w1549:bool)
            n883 = local read "Export graph2"() -> (w1547:bool)
            n884 = local read "Clear graph 2"() -> (w1546:bool)
            n885 = case shown="참" w1547 {
              frame False {
              }
              frame True {
                n886 = invoke on="IMU Graph" class="WFChart (엄격한)" method="Export Data to Excel"() -> ()  [unwired: 3 in, 3 out]
                n887 = local write "Export graph2"(FALSE ("그래프 반출")) -> ()
              }
            }
            n888 = case shown="참" w1549 {
              frame False {
              }
              frame True {
                n889 = invoke on="CDC(PCAP02) Graph" class="WFChart (엄격한)" method="Export Data to Excel"() -> ()  [unwired: 3 in, 3 out]
                n890 = local write "Export graph 1"(FALSE ("그래프 반출")) -> ()
              }
            }
            n891 = case shown="참" w1546 {
              frame False {
              }
              frame True {
                n892 = local write "Clear graph 2"(FALSE ("그래프 지우기")) -> ()
                n893 = call "SUB-BLE Rx data Clear.vi"() -> ()  [unwired: 6 in]
                n894 = property on="IMU Graph" class="WFChart (엄격한)"("History Data"=waveform(dbl)[][] [] ("히스토리 데이터")) -> ()  [unwired: 2 in, 2 out]
              }
            }
          }
          frame #9 {
            # "Offset (Save)"
            n895 = local read "Comm con status 1"() -> (w1561:bool)
            n896 = local read "Comm con status 1"() -> (w1562:bool)
            n897 = local read "Offset 2"() -> (w1560:bool)
            n898 = local read "Offset 1"() -> (w1563:bool)
            n899 = And(x=w1561, y=w1560) -> (x .and. y?=w1559:bool)
            n900 = And(x=w1562, y=w1563) -> (x .and. y?=w1564:bool)
            n901 = case shown="참" w1559 {
              frame False {
                n902 = local write "Offset 2"(FALSE ("Offset 1")) -> ()
              }
              frame True {
                n903 = local write "Offset 2"(FALSE ("Offset 1")) -> ()
                n904 = local write "Clear graph 2"(TRUE ("그래프 지우기")) -> ()
                n905 = for {
                  N: 50 -> [_]
                  tunnel: [w1635] -> w1613 mode=indexing
                  tunnel: [w1634] -> w1614 mode=indexing
                  tunnel: [w1633] -> w1615 mode=indexing
                  tunnel: [w1632] -> w1616 mode=indexing
                  tunnel: [w1631] -> w1617 mode=indexing
                  tunnel: [w1630] -> w1618 mode=indexing
                  n906 = local read "IMU Offet"() -> (w1629:T10)
                  n907 = call "SUB-BLE Rx data (Mon)-Wait.vi"("Timeout(ms)"=u16 200) -> ("RxReady"=w1636:bool)  [unwired: 4 in]
                  n908 = case shown="참" w1636 {
                    tunnel: [w1639 w1641] -> w1628
                    tunnel: w1629 -> [w1639 _]
                    frame False {
                    }
                    frame True {
                      n909 = call "SUB-BLE Rx data (Mon)-Classify.vi"() -> ("data out"=w1642:u8[], "Rx-mon"=w1640:bool)  [unwired: 5 in, 3 out]
                      n910 = case shown="참" w1640 {
                        tunnel: w1642 -> [_ w1644]
                        tunnel: [_ w1643] -> w1641
                        frame False {
                        }
                        frame True {
                          n911 = call "SUB-BLE Rx data (Mon)-CDC IMU.vi"("data in"=w1644) -> ("IMU data"=w1643:T10)  [unwired: 4 in, 3 out]
                        }
                      }
                    }
                  }
                  n912 = Unbundle By Name(w1628) -> ("Gyroscope X"=w1635:dbl, "Gyroscope Y"=w1634:dbl, "Gyroscope Z"=w1633:dbl, "Accelerometer X"=w1632:dbl, "Accelerometer Y"=w1631:dbl, "Accelerometer Z"=w1630:dbl)
                  n913 = Wait Until Next ms Multiple(millisecond multiple=u32 20 ("ms 배수")) -> ()  [unwired: 1 out]
                }
                n914 = call-poly <vilib>:"Mean.vi"("X"=w1613) -> ("mean"=w1620:dbl)  [unwired: 1 out]
                n915 = call-poly <vilib>:"Mean.vi"("X"=w1614) -> ("mean"=w1621:dbl)  [unwired: 1 out]
                n916 = call-poly <vilib>:"Mean.vi"("X"=w1615) -> ("mean"=w1622:dbl)  [unwired: 1 out]
                n917 = call-poly <vilib>:"Mean.vi"("X"=w1616) -> ("mean"=w1623:dbl)  [unwired: 1 out]
                n918 = call-poly <vilib>:"Mean.vi"("X"=w1617) -> ("mean"=w1624:dbl)  [unwired: 1 out]
                n919 = call-poly <vilib>:"Mean.vi"("X"=w1618) -> ("mean"=w1625:dbl)  [unwired: 1 out]
                n920 = Bundle By Name(cluster=T10 {"Gyroscope X"=0.0, "Gyroscope Y"=0.0, "Gyroscope Z"=0.0, "Accelerometer X"=0.0, "Accelerometer Y"=0.0, "Accelerometer Z"=0.0} ("IMU data"), "Gyroscope X"=w1620, "Gyroscope Y"=w1621, "Gyroscope Z"=w1622, "Accelerometer X"=w1623, "Accelerometer Y"=w1624, "Accelerometer Z"=w1625) -> (w1619:T10)
                n921 = local write "IMU Offet"(w1619) -> ()
              }
            }
            n922 = case shown="참" w1564 {
              frame False {
                n923 = local write "Offset 1"(FALSE ("Offset 1")) -> ()
              }
              frame True {
                n924 = local write "Offset 1"(FALSE ("Offset 1")) -> ()
                n925 = local write "Clear graph 1"(TRUE ("그래프 지우기")) -> ()
                n926 = local read "Offset Souce"() -> (w1568:enum32{"Normal", "Raw"})
                n927 = Equal?(x=w1568, y=enum32{"Normal", "Raw"}."Normal" ("Offset Souce")) -> (x = y?=w1566:bool)
                n928 = for {
                  N: 50 -> [_]
                  tunnel: [w1594] -> w1582 mode=indexing
                  tunnel: [w1593] -> w1581 mode=indexing
                  tunnel: [w1592] -> w1580 mode=indexing
                  tunnel: [w1591] -> w1579 mode=indexing
                  tunnel: [w1590] -> w1578 mode=indexing
                  tunnel: [w1589] -> w1577 mode=indexing
                  tunnel: w1566 -> [w1586]
                  n929 = local read "CDC Offet"() -> (w1587:T9)
                  n930 = call "SUB-BLE Rx data (Mon)-Wait.vi"("Timeout(ms)"=u16 200) -> ("RxReady"=w1595:bool)  [unwired: 4 in]
                  n931 = case shown="참" w1595 {
                    tunnel: [w1598 w1601] -> w1588
                    tunnel: w1587 -> [w1598 _]
                    tunnel: w1586 -> [_ w1599]
                    frame False {
                    }
                    frame True {
                      n932 = call "SUB-BLE Rx data (Mon)-Classify.vi"() -> ("data out"=w1602:u8[], "Rx-mon"=w1600:bool)  [unwired: 5 in, 3 out]
                      n933 = case shown="거짓" w1600 {
                        tunnel: w1602 -> [w1607 w1609]
                        tunnel: [w1606 w1608] -> w1601
                        tunnel: w1599 -> [w1605 _]
                        frame False {
                          n934 = call "SUB-BLE Rx data (Debug)-CDC.vi"("data in"=w1607) -> ("CDC debug"=w1603:T9, "CDC mon"=w1604:T9)  [unwired: 6 in]
                          n935 = Select(t=w1604, s=w1605, f=w1603) -> (s? t:f=w1606:T9)
                        }
                        frame True {
                          n936 = call "SUB-BLE Rx data (Mon)-CDC IMU.vi"("data in"=w1609) -> ("CDC data"=w1608:T9)  [unwired: 4 in, 3 out]
                        }
                      }
                    }
                  }
                  n937 = Unbundle By Name(w1588) -> ("Left Wing-A, C1/C0"=w1594:dbl, "Left Wing-B, C2/C0"=w1593:dbl, "Left Wing-C, C3/C0"=w1592:dbl, "Right Wing-A, C4/C0"=w1591:dbl, "Right Wing-B, C5/C0"=w1590:dbl, "Right Wing-C, C6/C0"=w1589:dbl)
                  n938 = Wait Until Next ms Multiple(millisecond multiple=u32 20 ("ms 배수")) -> ()  [unwired: 1 out]
                }
                n939 = call-poly <vilib>:"Mean.vi"("X"=w1582) -> ("mean"=w1574:dbl)  [unwired: 1 out]
                n940 = call-poly <vilib>:"Mean.vi"("X"=w1581) -> ("mean"=w1573:dbl)  [unwired: 1 out]
                n941 = call-poly <vilib>:"Mean.vi"("X"=w1580) -> ("mean"=w1572:dbl)  [unwired: 1 out]
                n942 = call-poly <vilib>:"Mean.vi"("X"=w1579) -> ("mean"=w1571:dbl)  [unwired: 1 out]
                n943 = call-poly <vilib>:"Mean.vi"("X"=w1578) -> ("mean"=w1570:dbl)  [unwired: 1 out]
                n944 = call-poly <vilib>:"Mean.vi"("X"=w1577) -> ("mean"=w1569:dbl)  [unwired: 1 out]
                n945 = Bundle By Name(cluster=T9 {"Left Wing-A, C1/C0"=0.0, "Left Wing-B, C2/C0"=0.0, "Left Wing-C, C3/C0"=0.0, "Right Wing-A, C4/C0"=0.0, "Right Wing-B, C5/C0"=0.0, "Right Wing-C, C6/C0"=0.0} ("CDC data"), "Left Wing-A, C1/C0"=w1574, "Left Wing-B, C2/C0"=w1573, "Left Wing-C, C3/C0"=w1572, "Right Wing-A, C4/C0"=w1571, "Right Wing-B, C5/C0"=w1570, "Right Wing-C, C6/C0"=w1569) -> (w1575:T9)
                n946 = local write "CDC Offet"(w1575) -> ()
              }
            }
          }
          frame #10 {
            # "Logging-GUI data"
            n947 = disable-structure shown="비활성화" {
              frame Disabled {
                n948 = local read "Data Logging"() -> (w1645:bool)
                n949 = case shown="참" w1645 {
                  frame False {
                    n950 = local read "Logging No."() -> (w1647:u32)
                    n951 = Not Equal To 0?(x=w1647) -> (x != 0?=w1646:bool)
                    n952 = case shown="참" w1646 {
                      frame False {
                      }
                      frame True {
                        n953 = local read "log refnum"() -> (w1649:refnum<file>)
                        n954 = local write "Logging No."(u32 0 ("Logging No.")) -> ()
                        n955 = Close File(refnum=w1649) -> ()  [unwired: 1 in, 2 out]
                      }
                    }
                  }
                  frame True {
                    n956 = stacked-sequence {
                      seq-local: [w1650 _] -> [_ w1702]
                      frame #0 {
                        n957 = local read "IMU data"() -> (w1653:T10)
                        n958 = local read "CDC data"() -> (w1670:T9)
                        n959 = Unbundle By Name(w1670) -> ("Left Wing-A, C1/C0"=w1667:dbl, "Left Wing-B, C2/C0"=w1666:dbl, "Left Wing-C, C3/C0"=w1665:dbl, "Right Wing-A, C4/C0"=w1664:dbl, "Right Wing-B, C5/C0"=w1663:dbl, "Right Wing-C, C6/C0"=w1662:dbl)
                        n960 = Unbundle By Name(w1653) -> ("Gyroscope X"=w1656:dbl, "Gyroscope Y"=w1657:dbl, "Gyroscope Z"=w1658:dbl, "Accelerometer X"=w1659:dbl, "Accelerometer Y"=w1660:dbl, "Accelerometer Z"=w1661:dbl)
                        n961 = Format Into String(format string="%.7f,%.7f,%.7f,%.7f,%.7f,%.7f," ("포맷 문자열"), initial string=",,(GUI) CDC Data," ("포맷 문자열"), w1667, w1666, w1665, w1664, w1663, w1662) -> (resulting string=w1652:string)  [unwired: 1 in, 1 out]
                        n962 = Format Into String(format string="%.6f,%.6f,%.6f,%.6f,%.6f,%.6f," ("포맷 문자열"), initial string=",(GUI) IMU Data," ("포맷 문자열"), w1656, w1657, w1658, w1659, w1660, w1661) -> (resulting string=w1651:string)  [unwired: 1 in, 1 out]
                        n963 = Concatenate Strings(w1652, w1651) -> (w1650:string)
                      }
                      frame #1 {
                        w1696 = T31 1 items=["사용자 홈"=0, "사용자 데스크탑"=1, "사용자 문서"=2, "사용자 어플리케이션 데이터"=3, "사용자 환경"=4, "사용자 임시"=5, "퍼블릭 문서"=6, "퍼블릭 어플리케이션 데이터"=7, "퍼블릭 환경"=8, "퍼블릭 캐시"=13, "시스템 코어 라이브러리"=9, "시스템 설치된 라이브러리"=10, "어플리케이션 파일"=11, "부팅 볼륨 루트"=12] ("system directory type")
                        # "첫행(타이틀)"
                        n964 = local read "Log no"() -> (w1671:string)
                        n965 = local read "Logging No."() -> (w1685:u32)
                        n966 = Format Date/Time String(time format string (%c)="Data Logging Start...  %Y/%m/%d %H:%M:%S" ("상태")) -> (date/time string=w1676:string)  [unwired: 2 in]
                        n967 = Format Into String(format string="\\\\GEN4 Data Logging(%s).csv" ("문자열"), w1671) -> (resulting string=w1672:string)  [unwired: 2 in, 1 out]
                        n968 = local read "RxD"() -> (w1706:string)
                        n969 = call <vilib>:"Get System Directory.vi"("system directory type"=w1696) -> ("system directory"=w1695:path)  [unwired: 10 in]
                        n970 = Format Into String(format string="\\r\\n\\r\\n%s\\r\\n%s\\r\\n" ("포맷 문자열"), w1676, "No.,Time,,Type,F/W ver.,(Raw)Left Wing-A,(Raw)Left Wing-B,(Raw)Left Wing-C,(Raw)Right Wing-A,(Raw)Right Wing-B,(Raw)Right Wing-C,(Raw)CDC Status,(Raw)Gyroscope X,(Raw)Gyroscope Y,(Raw)Gyroscope Z,(Raw)Accelerometer X,(Raw)Accelerometer Y,(Raw)Accelerometer Z,,Type,(GUI)Left Wing-A,(GUI)Left Wing-B,(GUI)Left Wing-C,(GUI)Right Wing-A,(GUI)Right Wing-B,(GUI)Right Wing-C,,Type,(GUI)Gyroscope X,(GUI)Gyroscope Y,(GUI)Gyroscope Z,(GUI)Accelerometer X,(GUI)Accelerometer Y,(GUI)Accelerometer Z" ("문자열")) -> (resulting string=w1674:string)  [unwired: 2 in, 1 out]
                        n971 = Increment(x=w1685) -> (x+1=w1701:u32)
                        n972 = Path To String(path=w1695) -> (string=w1694:string)
                        n973 = Equal To 0?(x=w1685) -> (x = 0?=w1683:bool)
                        n974 = Format Date/Time String(time format string (%c)="%Y/%m/%d %H:%M:%S%3u,,RXD Raw Data," ("상태")) -> (date/time string=w1708:string)  [unwired: 2 in]
                        n975 = Match Pattern(string=w1706, regular expression="#:" ("검색 문자열")) -> (after substring=w1704:string)  [unwired: 1 in, 3 out]
                        n976 = Format Into String(format string="%d," ("포맷 문자열"), w1685) -> (resulting string=w1699:string)  [unwired: 2 in, 1 out]
                        n977 = Concatenate Strings(w1694, w1672) -> (w1693:string)
                        n978 = local write "Logging No."(w1701) -> ()
                        n979 = String To Path(string=w1693) -> (path=w1692:path)
                        n980 = Open/Create/Replace File(file path (use dialog)=w1692, operation (0:open)=T29."open or create" ("동작(0:open)"), access (0:read/write)=enum16{"read/write", "read-only", "write-only"}."read/write" ("접근(0:읽기/쓰기)")) -> (refnum out=w1687:refnum<file>, error out=w1686:errorcluster)  [unwired: 3 in, 1 out]
                        n981 = Select(t=w1674, s=w1683, f="") -> (s? t:f=w1682:string)
                        n982 = Concatenate Strings(w1699, w1708, w1704, w1702, "\r\n") -> (w1681:string)
                        n983 = Get File Position(4:w1686, 7:w1687) -> (0:w1697:errorcluster, 2:w1684:i64, 3:w1698:refnum<file>)
                        n984 = Concatenate Strings(w1682, w1681) -> (w1680:string)
                        n985 = call <vilib>:"Write File+ (string).vi"("string"=w1680, "error in (no error)"=w1697, "pos offset (bytes:0)"=w1684, "refnum"=w1698) -> ("error out"=w1688:errorcluster, "dup refnum"=w1689:refnum<file>)  [unwired: 3 in, 1 out]
                        "log refnum" <- w1689
                        n986 = disable-structure shown="비활성화" {
                          disable-tunnel: w1689 -> [w1710 _]
                          disable-tunnel: w1688 -> [w1709 _]
                          frame Disabled {
                            n987 = Close File(refnum=w1710, error in=w1709) -> ()  [unwired: 2 out]
                          }
                          frame Enabled {
                          }
                        }
                      }
                    }
                  }
                }
              }
              frame Enabled {
              }
            }
          }
          frame #11 {
            # "Logging-BLE data"
            n988 = disable-structure shown="비활성화" {
              disable-tunnel: [w1715 _] -> _
              frame Disabled {
                n989 = local read "Timer-ble log"() -> (w1718:u32)
                n990 = Tick Count (ms)() -> (millisecond timer value=w1719:u32)
                n991 = Subtract(x=w1719, y=w1718) -> (x-y=w1717:u32)
                n992 = Greater Or Equal?(x=w1717, y=u32 3000) -> (x >= y?=w1715:bool)
              }
              frame Enabled {
              }
            }
            n993 = Compound Arithmetic op=AND ("복합 연산")("File Path Done", "Data Logging", "log data1") -> (w1714:bool)
            n994 = case shown="참" w1714 {
              frame False {
              }
              frame True {
                n995 = stacked-sequence {
                  seq-local: [w1720 _ _] -> [_ _ w1725]
                  frame #0 {
                    n996 = local read "log ble buf"() -> (w1720:string)
                  }
                  frame #1 {
                    n997 = Tick Count (ms)() -> (millisecond timer value=w1723:u32)
                    n998 = local write "Timer-ble log"(w1723) -> ()
                    n999 = local write "log data1"(FALSE ("log data1")) -> ()
                    n1000 = local write "log ble buf"("" ("log ble buf")) -> ()
                  }
                  frame #2 {
                    n1001 = String Length(string=w1725) -> (length=w1724:i32)
                    n1002 = case shown="1.." w1724 {
                      selector: w1724 -> [_ w1727]
                      tunnel: w1725 -> [_ w1729]
                      frame 0, Default {
                      }
                      frame 1.. {
                        n1003 = To Quad Integer(1:w1727) -> (0:w1726:i64)
                        n1004 = call "File_Interface.vi"("Number of byte"=w1726, "Mode"=File_Control_mode."Write", "Buffer"=w1729) -> ()  [unwired: 8 in, 1 out]
                      }
                    }
                  }
                }
              }
            }
          }
          frame #12 {
            n1005 = local write "Rx-mon"(FALSE) -> ()
            n1006 = local write "Rx-debug"(FALSE ("Rx-debug")) -> ()
          }
          frame #13 {
            # "Maximize window for debug"
            # "Maximize window"
            n1007 = local read "Maximize window"() -> (w1732:bool)
            n1008 = case shown="참" w1732 {
              frame False {
              }
              frame True {
                n1009 = First Call?() -> (First Call?: T/F=w1734:bool)
                n1010 = case shown="거짓" w1734 {
                  frame False {
                  }
                  frame True {
                    w1751 = 250  # 확장 창 크기
                    n1011 = Current VI's Path() -> (path=w1741:path)
                    n1012 = Open VI Reference(vi path=w1741) -> (vi reference=w1742:refnum<vi>, error out=w1743:errorcluster)  [unwired: 5 in]
                    n1013 = property class="VI"(reference=w1742, error in=w1743) -> (reference out=w1740:refnum<vi>, error out=w1738:errorcluster, "Front Panel.PanelBounds"=w1736:T32)
                    n1014 = Unbundle By Name(w1736) -> ("Left"=w1750:i16, "Top"=w1748:i16, "Right"=w1746:i16, "Bottom"=w1747:i16)
                    n1015 = expression code="x/2"(w1751) -> (w1745:i32)
                    n1016 = Add(x=w1746, y=w1745) -> (x+y=w1744:i32)
                    n1017 = Subtract(x=w1750, y=w1745) -> (x-y=w1749:i32)
                    n1018 = Bundle By Name(cluster=w1736, "Left"=w1749, "Top"=w1748, "Right"=w1744, "Bottom"=w1747) -> (w1735:T32)
                    n1019 = property class="VI"(reference=w1740, error in=w1738, "Front Panel.PanelBounds"=w1735) -> (reference out=w1739:refnum<vi>, error out=w1737:errorcluster)
                    n1020 = Close Reference(reference=w1739, error in (no error)=w1737) -> ()  [unwired: 1 out]
                  }
                }
                n1021 = local write "Maximize window"(FALSE ("창크게")) -> ()
              }
            }
          }
          frame #14 {
            n1022 = local read "Comm con status 1"() -> (w1753:bool)
            n1023 = case shown="참" w1753 {
              frame False {
              }
              frame True {
                n1024 = local read "ms timer 5"() -> (w1760:u32)
                n1025 = Tick Count (ms)() -> (millisecond timer value=w1759:u32)
                n1026 = Subtract(x=w1759, y=w1760) -> (x-y=w1761:u32)
                n1027 = Greater Or Equal?(x=w1761, y=u32 100) -> (x >= y?=w1757:bool)
                n1028 = case shown="참" w1757 {
                  frame False {
                  }
                  frame True {
                    n1029 = property on="BLE Interval buf" class="WFChart (엄격한)"() -> ("History Data"=w1765:u32[])  [unwired: 2 in, 2 out]
                    n1030 = local read "Port-act 1"() -> (w1770:refnum<visa-resource-name>)
                    n1031 = Array Size(array=w1765) -> (size(s)=w1764:i32)
                    n1032 = Tick Count (ms)() -> (millisecond timer value=w1766:u32)
                    n1033 = Greater?(x=w1764, y=20) -> (0:w1763:bool)
                    n1034 = local write "ms timer 5"(w1766) -> ()
                    n1035 = property class="Instr"(reference=w1770) -> ("Serial Settings:Number of Bytes at Serial Port"=w1769:u32)  [unwired: 1 in, 2 out]
                    n1036 = case shown="참" w1763 {
                      tunnel: w1765 -> [_ w1772]
                      frame False {
                      }
                      frame True {
                        n1037 = call-poly <vilib>:"Mean.vi"("X"=w1772) -> ("mean"=w1771:dbl)  [unwired: 1 out]
                        "BLE AVG-Interval Graph" <- w1771
                        n1038 = local write "BLE Interval Time(ms)"(w1771) -> ()
                      }
                    }
                    n1039 = case shown="0, 기본" w1769 {
                      frame 0, Default {
                        w1774 = T4 3 items=["System", "Persistent Store", "Attribute database", "Connection", "Attribute client", "Security Manager", "Generic Access Profile", "Hardware"] ("Command Class (System)")
                        w1777 = T3 0 items=["Command / Response"=0, "Event"=128] ("Message Type (Command / Response)")
                        # "Get Rssi"
                        n1040 = local read "Port-act 1"() -> (w1778:refnum<visa-resource-name>)
                        n1041 = Build Array(u8 0 ("Message ID (0x00)")) -> (w1775:u8[])
                        n1042 = call "ble_write_message.vi"("Command Class (System)"=w1774, "Message Type (Command / Response)"=w1777, "Payload(Empty)"=w1775, "Message ID (0x00)"=u8 1, "COM Bluegiga in"=w1778) -> ()  [unwired: 4 in, 3 out]
                      }
                      frame 1 {
                      }
                    }
                    n1043 = property on="BLE RSSI buf" class="WFChart (엄격한)"() -> ("History Data"=w1768:i16[])  [unwired: 2 in, 2 out]
                    n1044 = call-poly <vilib>:"Mean.vi"("X"=w1768) -> ("mean"=w1767:dbl)  [unwired: 1 out]
                    "BLE RSSI Graph" <- w1767
                    n1045 = local write "BLE RSSI (dBm)"(w1767) -> ()
                  }
                }
              }
            }
            n1046 = case shown="참" "Grahp Clear" {
              frame False {
              }
              frame True {
                n1047 = local write "BLE Interval Time(ms)"(0.0 ("BLE Interval Time(ms)")) -> ()
                n1048 = property on="BLE Interval buf" class="WFChart (엄격한)"("History Data"=u32[] [] ("히스토리 데이터")) -> ()  [unwired: 2 in, 2 out]
                n1049 = property on="BLE Interval Graph" class="WFChart (엄격한)"("History Data"=dbl[] [] ("히스토리 데이터")) -> ()  [unwired: 2 in, 2 out]
                n1050 = property on="BLE RSSI buf" class="WFChart (엄격한)"("History Data"=i16[] [] ("히스토리 데이터")) -> ()  [unwired: 2 in, 2 out]
                n1051 = local write "BLE RSSI (dBm)"(0.0 ("BLE RSSI (dBm)")) -> ()
                n1052 = property on="BLE RSSI Graph" class="WFChart (엄격한)"("History Data"=i16[] [] ("히스토리 데이터")) -> ()  [unwired: 2 in, 2 out]
                n1053 = call "SUB-BLE Rx data Clear.vi"() -> ()  [unwired: 6 in]
              }
            }
            n1054 = case shown="참" "CDC Graph plot" {
              frame False {
              }
              frame True {
                n1055 = control-ref of="CDC(PCAP02) Graph"() -> (w1756:refnum<vi>)
                n1056 = local write "Clear graph 1"(TRUE ("그래프 지우기")) -> ()
                n1057 = call "SUB-Graph plot select.vi"("CDC(PCAP02) Graph 2"=w1756) -> ()  [unwired: 3 in]
              }
            }
          }
          frame #15 {
            n1058 = case shown="참" "All Graph data save" {
              frame False {
              }
              frame True {
                n1059 = control-ref of="BLE AVG-Interval Graph"() -> (w1793:refnum<vi>)
                n1060 = control-ref of="BLE RSSI Graph"() -> (w1794:refnum<vi>)
                n1061 = property class="WFChart (엄격한)"(reference=w1793) -> ("History Data"=w1788:dbl[])  [unwired: 1 in, 2 out]
                n1062 = property class="WFChart (엄격한)"(reference=w1794) -> ("History Data"=w1789:dbl[])  [unwired: 1 in, 2 out]
                n1063 = Array Size(array=w1789) -> (size(s)=w1792:i32)
                n1064 = for {
                  N: w1792 -> [_]
                  tunnel: [w1797] -> w1791 mode=indexing
                  i -> [w1797]
                }
                n1065 = To Double Precision Float(number=w1791) -> (double precision float=w1790:dbl[])
                n1066 = Build Array(w1790, w1789, w1788) -> (w1787:dbl[][])
                n1067 = Transpose 2D Array(2D array=w1787) -> (transposed array=w1786:dbl[][])
                n1068 = call "Save_Array_Data_to_File.vi"("Header Array"=string[] ["Index", "RSSI(dB)", "Interval Time(ms)"], "Array"=w1786, "file path (use dialog)"="File path") -> ()  [unwired: 8 in, 1 out]
              }
            }
          }
        }
        n1069 = Wait Until Next ms Multiple(millisecond multiple=u32 4 ("ms 배수")) -> ()  [unwired: 1 out]
        n1070 = local read "stop"() -> (w573:bool)
      }
      n1071 = local read "Disconnection ocurrence"() -> (w342:refnum<k4>)
      n1072 = while {
        stop <- w526 stop-if-true
        # "If the value has changed Data Transfer Flag = On"
        # "Event"
        n1073 = event shown="[1] \"PWR OFF\": 값 변경" {
          selector: _ -> [_ _ _ _ _ _ _]
          dyn-events: _ -> [_ _ _ _ _ _ _]
          timeout: 50 -> [_ _ _ _ _ _ _]
          event Timeout {
            n1074 = event-data() -> ()  [unwired: 3 out]
          }
          event "PWR OFF": Value Change {
            n1075 = event-data() -> ("NewVal"=w527:bool)  [unwired: 1 out]
            n1076 = case shown="참" w527 {
              frame False {
              }
              frame True {
                n1077 = stacked-sequence {
                  frame #0 {
                    n1078 = local write "Handle"(u8 15 ("Handle")) -> ()
                    n1079 = local write "Data(h)"("DYSKIM" ("Data(h)")) -> ()
                  }
                  frame #1 {
                    n1080 = control-ref of="Send"() -> (w531:refnum<vi>)
                    n1081 = property class="Bool (엄격한)"(reference=w531, "Value"=TRUE ("값(신호)")) -> ()  [unwired: 1 in, 2 out]
                  }
                  frame #2 {
                    n1082 = Wait (ms)(milliseconds to wait=u32 200 ("대기 시간(ms)")) -> ()  [unwired: 1 out]
                  }
                  frame #3 {
                    n1083 = control-ref of="Comm con 1"() -> (w533:refnum<vi>)
                    n1084 = property class="Bool (엄격한)"(reference=w533, "Val(Sgnl)"=FALSE ("값(신호)")) -> ()  [unwired: 1 in, 2 out]
                  }
                  frame #4 {
                    n1085 = control-ref of="PWR OFF"() -> (w535:refnum<vi>)
                    n1086 = property class="Bool (엄격한)"(reference=w535, "Val(Sgnl)"=FALSE ("값(신호)")) -> ()  [unwired: 1 in, 2 out]
                  }
                }
              }
            }
          }
          event Key Down {
            # "Ctrl + 1"
            n1087 = event-data() -> ("Char"=w544:i16, "VKey"=w542:T25, "Mods"=w546:cluster{"Num Pad":bool, "Menu Key":bool})  [unwired: 6 out]
            n1088 = Unbundle By Name(w546) -> ("Menu Key"=w538:bool)
            n1089 = Equal?(x=eventvkey."ASCII" ("V 키"), y=w542) -> (x = y?=w540:bool)
            n1090 = Equal?(x=i16 49 ("문자"), y=w544) -> (x = y?=w541:bool)
            n1091 = And(x=w541, y=w540) -> (x .and. y?=w539:bool)
            n1092 = And(x=w539, y=w538) -> (x .and. y?=w537:bool)
            n1093 = case shown="거짓" w537 {
              frame False {
              }
              frame True {
                n1094 = local write "Maximize window"(TRUE ("창크게")) -> ()
              }
            }
          }
          event "Comm con 1": Value Change {
            n1095 = event-data() -> ("NewVal"=w548:bool)  [unwired: 6 out]
            n1096 = case shown="참" w548 {
              frame False {
                # "BLE Close"
                n1097 = local write "Port open 1"(FALSE) -> ()
                n1098 = local write "Port close 1"(TRUE) -> ()
              }
              frame True {
                # "BLE Open"
                n1099 = local write "Port open 1"(TRUE) -> ()
                n1100 = local write "Port close 1"(FALSE) -> ()
              }
            }
          }
          event "Setting load": Value Change {
            n1101 = event-data() -> ("NewVal"=w553:bool)  [unwired: 6 out]
            n1102 = case shown="참" w553 {
              frame False {
              }
              frame True {
                n1103 = local write "Setting load(led)"(TRUE ("Power On Flag")) -> ()
              }
            }
          }
          event "Data Logging": Value Change {
            n1104 = event-data() -> ("OldVal"=w555:bool)  [unwired: 6 out]
            n1105 = stacked-sequence {
              seq-local: [w558 _ _] -> [_ w563 _]
              tunnel: w555 -> [w559 _ _]
              frame #0 {
                n1106 = Equal?(x=w559, y=FALSE) -> (x = y?=w558:bool)
                n1107 = case shown="거짓" w558 {
                  tunnel: [File_Control_mode."Close" ("Mode") File_Control_mode."Open" ("Mode")] -> w557
                  frame False {
                  }
                  frame True {
                  }
                }
                n1108 = control-ref of="Log no"() -> (w556:refnum<vi>)
                n1109 = call "File_Interface.vi"("Mode"=w557, "Log no"=w556) -> ()  [unwired: 9 in, 1 out]
              }
              frame #1 {
                n1110 = control-ref of="File Path Done"() -> (w564:refnum<vi>)
                n1111 = property class="Bool (엄격한)"(reference=w564, "Value"=w563) -> ()  [unwired: 1 in, 2 out]
              }
              frame #2 {
                n1112 = Tick Count (ms)() -> (millisecond timer value=w565:u32)
                n1113 = local write "Timer-ble log"(w565) -> ()
              }
            }
          }
          event Panel Close? {
            n1114 = event-data() -> ()  [unwired: 5 out]
            n1115 = stacked-sequence {
              frame #0 {
                n1116 = local read "Disconnection ocurrence"() -> (w568:refnum<k4>)
                n1117 = Set Occurrence(w568) -> ()
              }
              frame #1 {
                n1118 = Wait (ms)(milliseconds to wait=u32 500 ("대기 시간(ms)")) -> ()  [unwired: 1 out]
              }
              frame #2 {
                n1119 = local read "Disconnection ocurrence"() -> (w570:refnum<k4>)
                n1120 = Set Occurrence(w570) -> ()
              }
            }
            n1121 = local write "stop"(TRUE ("stop")) -> ()
            n1122 = event-data("Discard?"=TRUE ("stop")) -> ()  [unwired: 1 in, 1 out]
          }
        }
        n1123 = local read "stop"() -> (w526:bool)
      }
      n1124 = while {
        stop <- w389 stop-if-true
        # "BLE RxD handle"
        n1125 = local read "Comm con status 1"() -> (w388:bool)
        n1126 = local read "Port-act 1"() -> (w387:refnum<visa-resource-name>)
        n1127 = case shown="참" w388 {
          tunnel: w387 -> [_ w394]
          frame False {
          }
          frame True {
            n1128 = property class="Instr"(reference=w394) -> (reference out=w393:refnum<visa-resource-name>, error out=w392:errorcluster, "Serial Settings:Number of Bytes at Serial Port"=w391:u32)  [unwired: 1 in]
            n1129 = case shown="4.." w391 {
              tunnel: w393 -> [_ w435]
              tunnel: w392 -> [_ w434]
              frame 0, Default {
                # "BLE Tx sender"
                n1130 = local read "Comm con status 1"() -> (w396:bool)
                n1131 = And(x="Send", y=w396) -> (x .and. y?=w401:bool)
                n1132 = And(x=w396, y="Mode Selection") -> (x .and. y?=w400:bool)
                n1133 = And(x=w396, y="Save") -> (x .and. y?=w399:bool)
                n1134 = And(x=w396, y="Set Inverval Time") -> (x .and. y?=w395:bool)
                n1135 = case shown="참" w401 {
                  frame False {
                  }
                  frame True {
                    (unwired) u16 12 ("Handle")
                    # "데이터 전송\n- 핸들/0x01"
                    n1136 = control-ref of="Send"() -> (w427:refnum<vi>)
                    n1137 = property class="Bool (엄격한)"(reference=w427, "Value"=FALSE ("값(신호)")) -> ()  [unwired: 1 in, 2 out]
                    n1138 = local read "Data(h)"() -> (w429:string)
                    n1139 = local read "Connection Status"() -> (w430:T5)
                    n1140 = local read "Port-act 1"() -> (w431:refnum<visa-resource-name>)
                    n1141 = String To Byte Array(string=w429) -> (unsigned byte array=w428:u8[])
                    n1142 = local read "Handle"() -> (w432:u8)
                    n1143 = call-poly "ble_write_by_handle.vi"("Connection Status"=w430, "Handle"=w432, "data (uint8array)"=w428, "COM Bluegiga in"=w431) -> ()  [unwired: 6 in, 2 out]
                  }
                }
                n1144 = case shown="참" w400 {
                  frame False {
                  }
                  frame True {
                    # "데이터 전송\n- 핸들 0x0B"
                    n1145 = control-ref of="Mode Selection"() -> (w418:refnum<vi>)
                    n1146 = property class="Bool (엄격한)"(reference=w418, "Value"=FALSE) -> ()  [unwired: 1 in, 2 out]
                    n1147 = case shown="\"Debugging 1\"" "Operation Mode" {
                      tunnel: ["imt" ("문자열") "JsP" ("문자열") "NFT" ("문자열")] -> w415
                      frame "Normal Operation", Default {
                      }
                      frame "Debugging 1" {
                      }
                      frame "Debugging 2" {
                      }
                    }
                    n1148 = local read "Connection Status"() -> (w421:T5)
                    n1149 = local read "Port-act 1"() -> (w422:refnum<visa-resource-name>)
                    n1150 = String To Byte Array(string=w415) -> (unsigned byte array=w420:u8[])
                    n1151 = call-poly "ble_write_by_handle.vi"("Connection Status"=w421, "Handle"=u16 11, "data (uint8array)"=w420, "COM Bluegiga in"=w422) -> ()  [unwired: 6 in, 2 out]
                  }
                }
                n1152 = case shown="참" w395 {
                  frame False {
                  }
                  frame True {
                    n1153 = local read "Connection Status"() -> (w408:T5)
                    n1154 = call "SUB_Write_GEN4_Init_data_V2_0_1.vi"("Interval Time"="Interval Time", "Mode"=write_mode."Interval Change", "Connection Status"=w408) -> ()  [unwired: 9 in]
                    n1155 = property on="BLE Interval Graph" class="WFChart (엄격한)"("History Data"=dbl[] [] ("히스토리 데이터")) -> ()  [unwired: 2 in, 2 out]
                    n1156 = property on="BLE Interval buf" class="WFChart (엄격한)"("History Data"=u32[] [] ("히스토리 데이터")) -> ()  [unwired: 2 in, 2 out]
                  }
                }
                n1157 = case shown="참" w399 {
                  frame False {
                  }
                  frame True {
                    n1158 = local read "Connection Status"() -> (w413:T5)
                    n1159 = property on="ROM Table 2" class="Tbl (엄격한)"() -> ("Value"=w414:string[][])  [unwired: 2 in, 2 out]
                    n1160 = call "SUB_Parsing_from_table_to_cluster.vi"("ROM Table"=w414) -> ("PCAP zero information"=w410:T33, "Cal information"=w411:T34, "Device information"=w412:T35)  [unwired: 8 in]
                    n1161 = call "SUB_Write_GEN4_Init_data_V2_0_1.vi"("PCAP zero information"=w410, "Mode"=enum16{"Save Flash", "Visa save"}."Save Flash", "Connection Status"=w413, "Cal information"=w411, "Device information"=w412) -> ()  [unwired: 7 in]
                  }
                }
              }
              frame 4.. {
                # "Rx Packet Data - Process"
                n1162 = call "ble_read_message.vi"("error in (no error)"=w434, "COM Bluegiga in"=w435) -> ("message package"=w433:u8[])  [unwired: 7 in, 2 out]
                n1163 = stacked-sequence {
                  seq-local: [_ w439 _ _ _ _] -> [_ _ w467 w477 w481 w492]
                  tunnel: w433 -> [_ w440 _ _ _ _]
                  frame #0 {
                    n1164 = local write "Packet Detect"(FALSE ("Packet Detect")) -> ()
                  }
                  frame #1 {
                    # "ble_evt_attclient_attribute_value"
                    n1165 = call "BLED1112-Rx Packet parser (EVENT-Attribute Client).vi"("message package"=w440) -> ("message out"=w439:u8[], "Packet OK"=w438:bool, "Data Structure"=w437:T2)  [unwired: 2 in]
                    n1166 = case shown="참" w438 {
                      tunnel: w437 -> [_ w445]
                      frame False {
                      }
                      frame True {
                        n1167 = local read "Data Logging"() -> (w444:bool)
                        n1168 = Unbundle By Name(w445) -> ("Attribute value (data)"=w446:u8[])
                        n1169 = local write "Packet Detect"(TRUE ("Packet Detect")) -> ()
                        n1170 = Byte Array To String(unsigned byte array=w446) -> (string=w449:string)
                        n1171 = local write "Rx buf 1"(w449) -> ()
                        n1172 = call "SUB-BLE Rx data save.vi"("Rx Packet Structure"=w445, "BLE RxD"=w446) -> ("Full packet"=w441:u8[], "Mon Packet?"=w442:bool)  [unwired: 1 in, 1 out]
                        n1173 = And(x=w442, y=w444) -> (x .and. y?=w443:bool)
                        n1174 = case shown="참" w442 {
                          frame False {
                          }
                          frame True {
                            n1175 = local read "ms timer 4"() -> (w453:u32)
                            n1176 = Tick Count (ms)() -> (millisecond timer value=w451:u32)
                            n1177 = Subtract(x=w451, y=w453) -> (x-y=→"BLE Interval buf":u32)
                            n1178 = local write "ms timer 4"(w451) -> ()
                          }
                        }
                        n1179 = local read "Rx Cnt"() -> (w447:i32)
                        n1180 = case shown="참" w443 {
                          tunnel: w441 -> [_ w458]
                          tunnel: w447 -> [_ w455]
                          frame False {
                          }
                          frame True {
                            # "Save log data"
                            n1181 = local read "log ble buf"() -> (w463:string)
                            n1182 = Format Into String(format string="%06d," ("포맷 문자열"), w455) -> (resulting string=w456:string)  [unwired: 2 in, 1 out]
                            n1183 = Array To Spreadsheet String(delimiter (Tab)="," ("포맷 문자열"), array=w458, 3:"%02X" ("포맷 문자열")) -> (spreadsheet string=w459:string)
                            n1184 = Format Date/Time String(time format string (%c)="%H:%M:%S%3u," ("상태")) -> (date/time string=w461:string)  [unwired: 2 in]
                            n1185 = Concatenate Strings(w463, w456, w461, w459) -> (w462:string)
                            n1186 = local write "log ble buf"(w462) -> ()
                            n1187 = local write "log data1"(TRUE ("log data1")) -> ()
                          }
                        }
                        n1188 = Increment(x=w447) -> (x+1=w450:i32)
                        n1189 = local write "Rx Cnt"(w450) -> ()
                        "Rx Packet Structure" <- w445
                      }
                    }
                  }
                  frame #2 {
                    # "Rx Packet parser (EVENT-Connection status)"
                    n1190 = local read "Packet Detect"() -> (w466:bool)
                    n1191 = case shown="거짓" w466 {
                      tunnel: w467 -> [w470 _]
                      frame False {
                        n1192 = call "BLED1112-Rx Packet parser (EVENT-Connection status).vi"("message package"=w470) -> ("Packet OK"=w469:bool, "Data Structure"=w468:T36)  [unwired: 2 in, 1 out]
                        n1193 = case shown="참" w469 {
                          tunnel: w468 -> [_ w475]
                          frame False {
                          }
                          frame True {
                            n1194 = Unbundle By Name(w475) -> ("bonding(0xFF)"=w474:u8)
                            n1195 = local write "Packet Detect"(TRUE ("Packet Detect")) -> ()
                            n1196 = Not Equal?(x=w474, y=255 ("Rx Cnt")) -> (x != y?=w472:bool)
                            n1197 = local write "Disconnected"(w472) -> ()
                          }
                        }
                      }
                      frame True {
                      }
                    }
                  }
                  frame #3 {
                    # "Rx Packet parser (RESPONSE GAP)"
                    n1198 = local read "Packet Detect"() -> (w476:bool)
                    n1199 = case shown="참" w476 {
                      tunnel: w477 -> [w479 _]
                      frame False {
                        n1200 = call "BLED1112-Rx Packet parser (RESPONSE-GAP).vi"("message package"=w479) -> ("Packet OK"=w478:bool)  [unwired: 2 in, 2 out]
                        n1201 = case shown="거짓" w478 {
                          frame False {
                          }
                          frame True {
                            n1202 = local write "Packet Detect"(TRUE ("Packet Detect")) -> ()
                          }
                        }
                      }
                      frame True {
                      }
                    }
                  }
                  frame #4 {
                    # "Rx Packet parser (EVENT-Disconnected)"
                    n1203 = local read "Packet Detect"() -> (w482:bool)
                    n1204 = case shown="참" w482 {
                      tunnel: w481 -> [w484 _]
                      frame False {
                        n1205 = call "BLED1112-Rx Packet parser (EVENT-Disconnected).vi"("message package"=w484) -> ("Packet OK"=w483:bool)  [unwired: 2 in, 2 out]
                        n1206 = case shown="참" w483 {
                          frame False {
                          }
                          frame True {
                            n1207 = local write "Packet Detect"(TRUE ("Packet Detect")) -> ()
                            n1208 = local write "Disconnected"(TRUE ("Packet Detect")) -> ()
                            n1209 = local write "Comm con status 1"(FALSE ("Packet Detect")) -> ()
                            n1210 = local write "Comm con 1"(FALSE ("Packet Detect")) -> ()
                            n1211 = local write "ACT-Comm"(FALSE ("Packet Detect")) -> ()
                            n1212 = local read "Disconnection ocurrence"() -> (w485:refnum<k4>)
                            n1213 = disable-structure shown="비활성화" {
                              frame Disabled {
                                n1214 = One Button Dialog(message="BLE Disconnected!" ("메시지")) -> ()  [unwired: 1 in, 1 out]
                              }
                              frame Enabled {
                              }
                            }
                            n1215 = Set Occurrence(w485) -> ()
                          }
                        }
                      }
                      frame True {
                      }
                    }
                  }
                  frame #5 {
                    # "Rx Packet parser (Get Rssi))"
                    n1216 = local read "Packet Detect"() -> (w493:bool)
                    n1217 = case shown="거짓" w493 {
                      tunnel: w492 -> [w496 _]
                      frame False {
                        n1218 = call "BLED1112-Rx Packet parser (Get Rssi).vi"("message package"=w496) -> ("Packet OK"=w495:bool, "Data Structure"=w494:T37)  [unwired: 2 in, 1 out]
                        n1219 = case shown="참" w495 {
                          tunnel: w494 -> [_ w498]
                          frame False {
                          }
                          frame True {
                            n1220 = local write "Packet Detect"(TRUE ("Packet Detect")) -> ()
                            n1221 = Unbundle By Name(w498) -> ("rssi"=→"BLE RSSI buf":i16)
                          }
                        }
                      }
                      frame True {
                      }
                    }
                  }
                }
              }
            }
          }
        }
        n1222 = Wait Until Next ms Multiple(millisecond multiple=u32 1 ("ms 배수")) -> ()  [unwired: 1 out]
        n1223 = local read "stop"() -> (w389:bool)
      }
      n1224 = while {
        tunnel: w342 -> [w345]
        stop <- w343 stop-if-true
        # "Auto Reconneciton"
        n1225 = Wait on Occurrence(2:w345) -> (0:w344:bool)  [unwired: 2 in]
        n1226 = stacked-sequence {
          seq-local: [w346 _] -> [_ w352]
          tunnel: w344 -> [_ _]
          tunnel: [_ w352] -> w343
          frame #0 {
            n1227 = local read "stop"() -> (w346:bool)
            n1228 = case shown="거짓" w346 {
              frame False {
                n1229 = Wait (ms)(milliseconds to wait=u32 100 ("대기 시간(ms)")) -> ()  [unwired: 1 out]
                n1230 = call "SUB-Text_Blink.vi"("Timeout"=3.0, "text color"=u32 16711680, "Message"="\nDisconnected") -> ()  [unwired: 9 in]
              }
              frame True {
              }
            }
          }
          frame #1 {
            n1231 = Or(x="PWR OFF", y=w352) -> (x .or. y?=w353:bool)
            n1232 = case shown="거짓" w353 {
              frame False {
                n1233 = control-ref of="Connection Status"() -> (w362:refnum<vi>)
                n1234 = property class="Clust (엄격한)"(reference=w362) -> ("Value"=w361:T5)  [unwired: 1 in, 2 out]
                n1235 = Unbundle By Name(w361) -> ("MAC Address"=w359:string, "Address Type"=w358:T6)
                n1236 = local read "Port-act 1"() -> (w360:refnum<visa-resource-name>)
                n1237 = call "BLED1112_auto-connection.vi"("COM Bluegiga in"=w360, "MAC Address"=w359, "Address Type"=w358) -> ("Connection Ok"=w357:bool, "Device Name"=w355:string, "Connection Status"=w354:T5)  [unwired: 7 in, 3 out]
                n1238 = Not(x=w357) -> (.not. x?=w356:bool)
                n1239 = local write "Rx-mon"(w356) -> ()
                n1240 = case shown="참" w356 {
                  tunnel: w355 -> [_ w369]
                  tunnel: w354 -> [_ w368]
                  frame True {
                    # "Received data error status"
                    n1241 = local read "Port-act 1"() -> (w366:refnum<visa-resource-name>)
                    n1242 = VISA Close(VISA resource name=w366) -> ()  [unwired: 1 in, 1 out]
                    n1243 = local write "Comm con status 1"(FALSE ("Connected")) -> ()
                    n1244 = local write "*Board ID1"("None...." ("*Board ID")) -> ()
                    n1245 = local write "Comm con 1"(FALSE ("보드 통신 연결 1")) -> ()
                    n1246 = local write "Rx-mon"(TRUE ("수신 실패(T) 2")) -> ()
                  }
                  frame False {
                    n1247 = local write "Connection Status"(w368) -> ()
                    n1248 = local write "Device Name"(w369) -> ()
                    n1249 = stacked-sequence {
                      frame #0 {
                        # "BLE 버퍼 클리어"
                        n1250 = call "SUB-BLE Rx data Clear.vi"() -> ()  [unwired: 6 in]
                        n1251 = Wait Until Next ms Multiple(millisecond multiple=u32 200 ("ms 타이머 값")) -> ()  [unwired: 1 out]
                      }
                      frame #1 {
                        n1252 = local write "Comm con status 1"(TRUE ("Connected")) -> ()
                      }
                    }
                    n1253 = local write "*Board ID1"("" ("*Board ID")) -> ()
                    n1254 = local write "Setting load(led)"(FALSE ("Power On Flag")) -> ()
                    n1255 = local write "Comm err cnt 1"(0 ("통신에러카운트")) -> ()
                    n1256 = local write "Clear graph 1"(FALSE ("그래프 지우기")) -> ()
                    n1257 = local write "Clear graph 2"(FALSE ("그래프 지우기")) -> ()
                    n1258 = local write "Comm con 1"(TRUE ("포트 연결")) -> ()
                    n1259 = local write "RxD"("Connection. OK....." ("status string")) -> ()
                    n1260 = disable-structure shown="비활성화" {
                      frame Disabled {
                        w380 = T9 {"Left Wing-A, C1/C0"=0.0, "Left Wing-B, C2/C0"=0.0, "Left Wing-C, C3/C0"=0.0, "Right Wing-A, C4/C0"=0.0, "Right Wing-B, C5/C0"=0.0, "Right Wing-C, C6/C0"=0.0} ("CDC data")
                        w379 = T10 {"Gyroscope X"=0.0, "Gyroscope Y"=0.0, "Gyroscope Z"=0.0, "Accelerometer X"=0.0, "Accelerometer Y"=0.0, "Accelerometer Z"=0.0} ("IMU data")
                        n1261 = local write "Data Log"("" ("Data Log")) -> ()
                        n1262 = local write "Data_mon(h)"("" ("Data_mon")) -> ()
                        n1263 = local write "CDC Offet"(w380) -> ()
                        n1264 = local write "CDC data"(w380) -> ()
                        n1265 = local write "IMU data"(w379) -> ()
                        n1266 = local write "IMU Offet"(w379) -> ()
                      }
                      frame Enabled {
                      }
                    }
                  }
                }
              }
              frame True {
                n1267 = control-ref of="PWR OFF"() -> (w383:refnum<vi>)
                n1268 = property class="Bool (엄격한)"(reference=w383, "Value"=FALSE ("값(신호)")) -> ()  [unwired: 1 in, 2 out]
                n1269 = disable-structure shown="비활성화" {
                  frame Disabled {
                    n1270 = control-ref of="Comm con 1"() -> (w385:refnum<vi>)
                    n1271 = property class="Bool (엄격한)"(reference=w385, "Val(Sgnl)"=FALSE ("값(신호)")) -> ()  [unwired: 1 in, 2 out]
                  }
                  frame Enabled {
                  }
                }
              }
            }
          }
        }
      }
      n1272 = while {
        stop <- w509 stop-if-true
        # "Load test-one time"
        n1273 = stacked-sequence {
          frame #0 {
            n1274 = local read "Force Set"() -> (w511:bool)
            n1275 = case shown="참" w511 {
              frame False {
              }
              frame True {
                n1276 = stacked-sequence {
                  frame #0 {
                    n1277 = local read "Port-FTS"() -> (w515:refnum<visa-resource-name>)
                    n1278 = local read "Load(lb)"() -> (w514:dbl)
                    n1279 = call "_Serial_Mark10-Control (Press Config).vi"("FTS Operation state"=T24 "Start pressure control" ("FTS 제어 상태"), "Press Setting(lb)"=w514, "Serial Port"=w515) -> ("Communication is normal"=w513:bool)  [unwired: 2 out]
                    n1280 = case shown="거짓" w513 {
                      frame False {
                        n1281 = One Button Dialog(message="Can't find equipment!" ("메시지")) -> ()  [unwired: 1 in, 1 out]
                      }
                      frame True {
                      }
                    }
                  }
                  frame #1 {
                    n1282 = local write "Force Set"(FALSE ("Force Set")) -> ()
                  }
                }
              }
            }
          }
          frame #1 {
            n1283 = local read "Head Up"() -> (w518:bool)
            n1284 = case shown="참" w518 {
              frame False {
              }
              frame True {
                n1285 = stacked-sequence {
                  frame #0 {
                    n1286 = local read "Port-FTS"() -> (w522:refnum<visa-resource-name>)
                    n1287 = local read "Load(lb)"() -> (w521:dbl)
                    n1288 = call "_Serial_Mark10-Control (Press Config).vi"("FTS Operation state"=T24 "Move Header Up", "Press Setting(lb)"=w521, "Serial Port"=w522) -> ("Communication is normal"=w520:bool)  [unwired: 2 out]
                    n1289 = case shown="거짓" w520 {
                      frame False {
                        n1290 = One Button Dialog(message="Can't find equipment!" ("메시지")) -> ()  [unwired: 1 in, 1 out]
                      }
                      frame True {
                      }
                    }
                  }
                  frame #1 {
                    n1291 = local write "Head Up"(FALSE ("Force Set")) -> ()
                  }
                }
              }
            }
          }
        }
        n1292 = Wait Until Next ms Multiple(millisecond multiple=u32 300 ("ms 배수")) -> ()  [unwired: 1 out]
        n1293 = local read "stop"() -> (w509:bool)
      }
      n1294 = while {
        stop <- w504 stop-if-true
        # "test-LED blink"
        n1295 = local read "Force Set"() -> (w502:bool)
        n1296 = local read "Test Start"() -> (w503:bool)
        n1297 = local read "Head Up"() -> (w500:bool)
        n1298 = Compound Arithmetic op=OR ("복합 연산")(w503, w502, w500) -> (w501:bool)
        n1299 = case shown="참" w501 {
          frame False {
            n1300 = local write "FTS Testing"(FALSE ("FTS 시험 진행")) -> ()
          }
          frame True {
            n1301 = local read "FTS Testing"() -> (w508:bool)
            n1302 = Not(x=w508) -> (.not. x?=w507:bool)
            n1303 = local write "FTS Testing"(w507) -> ()
          }
        }
        n1304 = Wait Until Next ms Multiple(millisecond multiple=u32 300 ("ms 배수")) -> ()  [unwired: 1 out]
        n1305 = local read "stop"() -> (w504:bool)
      }
    }
    frame #6 {
      # "Close Serial Port"
      n1306 = local read "Comm con 1"() -> (w1798:bool)
      n1307 = case shown="참" w1798 {
        frame False {
        }
        frame True {
          # "BLE 통신 종료"
          n1308 = local read "Port-act 1"() -> (w1799:refnum<visa-resource-name>)
          n1309 = local read "Connection Status"() -> (w1804:T5)
          n1310 = call "_Serial_buf clear.vi"("Serial Port"=w1799) -> ("에러 출력"=w1802:errorcluster, "Serial Port 2"=w1803:refnum<visa-resource-name>)  [unwired: 3 in]
          n1311 = call "ble_disconnect_device.vi"("Connection Status"=w1804, "error in (no error)"=w1802, "COM Bluegiga in"=w1803) -> ("error out"=w1801:errorcluster, "COM Bluegiga out"=w1800:refnum<visa-resource-name>)  [unwired: 7 in]
          n1312 = VISA Close(VISA resource name=w1800, error in (no error)=w1801) -> ()  [unwired: 1 out]
        }
      }
    }
    frame #7 {
      # "Save Program Configuration to File"
      n1313 = call <vilib>:"Open Config Data.vi"("configuration file path"=w1809) -> ("error out"=w1812:errorcluster, "refnum"=w1811:T30)  [unwired: 2 in, 7 out]
      n1314 = stacked-sequence {
        tunnel: w1811 -> [w1816 w1819 w1824 w1829 w1834]
        tunnel: w1812 -> [w1815 w1818 w1823 w1828 w1833]
        tunnel: "GUI Setting" ("section") -> [w1817 w1820 w1825 w1830 _]
        tunnel: [_ _ _ _ w1834] -> w1808
        tunnel: [_ _ _ _ w1833] -> w1807
        frame #0 {
          w1814 = "Com Port-Board1"  # Key 1
          n1315 = local read "Port-set 1"() -> (w1813:refnum<visa-resource-name>)
          n1316 = call-poly <vilib>:"Write Key.vi"("section"=w1817, "error in (no error)"=w1815, "value"=w1813, "key"=w1814, "refnum"=w1816) -> ()  [unwired: 1 in, 6 out]
        }
        frame #1 {
          w1822 = "Com Port-FTS"  # Key 1
          n1317 = local read "Port-FTS"() -> (w1821:refnum<visa-resource-name>)
          n1318 = call-poly <vilib>:"Write Key.vi"("section"=w1820, "error in (no error)"=w1818, "value"=w1821, "key"=w1822, "refnum"=w1819) -> ()  [unwired: 1 in, 6 out]
        }
        frame #2 {
          w1827 = "Logno"  # Key 1
          n1319 = local read "Log no"() -> (w1826:string)
          n1320 = call-poly <vilib>:"Write Key.vi"("section"=w1825, "error in (no error)"=w1823, "value"=w1826, "key"=w1827, "refnum"=w1824) -> ()  [unwired: 1 in, 6 out]
        }
        frame #3 {
          w1832 = "Interval(ms)"  # Key 1
          n1321 = local read "Update(ms)"() -> (w1831:u16)
          n1322 = call-poly <vilib>:"Write Key.vi"("section"=w1830, "error in (no error)"=w1828, "value"=w1831, "key"=w1832, "refnum"=w1829) -> ()  [unwired: 7 out]
        }
        frame #4 {
        }
      }
      n1323 = call <vilib>:"Close Config Data.vi"("error in (no error)"=w1807, "refnum"=w1808) -> ()  [unwired: 1 in, 9 out]
      n1324 = call "Read and Write Controls to Automatic Config File.vi"("Action"=RWC_Actions."Write", "Control References"=w1805) -> ()  [unwired: 9 in, 1 out]
    }
    frame #8 {
      # "End"
      n1325 = call "SUB-Exit.vi"() -> ()  [unwired: 4 in]
    }
  }
  n1326 = control-ref of="Log no"() -> (w2:refnum<vi>)
  n1327 = local write "Mode"(TRUE ("Mode")) -> ()
  n1328 = local write "Rx-debug"(FALSE ("Rx-debug")) -> ()
  n1329 = local write "Offset Souce"(enum32{"Normal", "Raw"}."Normal" ("Offset Souce")) -> ()
  n1330 = control-ref of="Linerity State"() -> (w3:refnum<vi>)
  n1331 = property class="Enum (엄격한)"(reference=w3, "Value"=Linerity_State."Initial" ("Linerity State")) -> ()  [unwired: 1 in, 2 out]
  n1332 = local write "Packet No."(0 ("Packet No.")) -> ()
  n1333 = property class="Str"(reference=w2, "DisabledEnum"=T13."Enabled" ("비활성화")) -> ()  [unwired: 1 in, 2 out]
